vi "myRIO_BRig_RT_v0,60__PortC.vi"() -> ()   [LabVIEW 2014]
uses:
  myRIO_BRig_RT__Case_Exp_stateList.ctl
  myRIO_BRig_RT__Case_NonExp_stateList.ctl
  <vilib>/Platform/TimedLoop/XDataNode/timing_clust.ctl
  <vilib>/Platform/TimedLoop/XDataNode/nitl_modes.ctl
  <vilib>/Platform/TimedLoop/XDataNode/wakeup.ctl
  <vilib>/WebDAVClient/Advanced/SessionHandle.ctl
  <vilib>/myRIO/Common/Instrument Driver Framework/myRIO v1.0/UART/vis/myRIO v1.0 Close UART.vi
  <vilib>/FPGAPlugInAG/myRIO-1900/niLvFpga_Open_myRIO-1900.vi
  <vilib>/rvi/interface/common/dynamic/niFpgaDynamicAddResources.vi
  <vilib>/Utility/error.llb/Error Cluster From Error Code.vi
  <vilib>/rvi/errors/niLvFpgaAdjustHostInterfaceError.vi
  <vilib>/FPGAPlugInAG/Dynamic/niLvFpga_Close_Dynamic.vi
  <vilib>/myRIO/Common/Instrument Driver Framework/Utilities/vis/FPGA Ref Manager.vi
  <vilib>/myRIO/Common/Instrument Driver Framework/myRIO v1.0/myRIO v1.0 Reset FPGA.vi
  <vilib>/myRIO/Common/Instrument Driver Framework/myRIO v1.0/IRQ/vis/myRIO v1.0 IRQ Info FGV.vi
  <vilib>/myRIO/Common/Instrument Driver Framework/myRIO v1.0/IRQ/vis/myRIO v1.0 Timer IRQ Info FGV.vi
  <vilib>/myRIO/Common/Instrument Driver Framework/myRIO v1.0/IRQ/vis/myRIO v1.0 ISR Agent.vi
  <vilib>/rvi/interface/nirviOpenFPGA/nirviOpenFPGA.xnode
  FPGA Bitfiles/myRIOBRig_FPGATarget_myRIOBRigFPGAv3,_GOpVR-pcl6w.lvbitx
  myRIO_BRig_FPGA_v3,51__PortC__testWarmup.vi
  <vilib>/rvi/interface/nirviReadWriteControl/nirviReadWriteControl.xnode
  <vilib>/Platform/TimedLoop/XDataNode/XDataNode.xnode
  <vilib>/rvi/interface/nirviCloseFPGA/nirviCloseFPGA.xnode
  <vilib>/Platform/TimedLoop/XDataNode/XDNodeRunTimeDep.lvlib
  <vilib>/rvi/interface/Simulation/niFpgaSimulationCallBeginRW.vi
  <vilib>/myRIO/Instrument Drivers/Utilities/Utilities.lvlib
  <vilib>/WebDAVClient/NI_WebDAV.lvlib
  NiFpgaLv.dll
panel:
  in  "count_warmup_R_reset":bool
  in  "count_warmup_L_reset":bool
  out "count_warmup_R":u16
  out "count_warmup_L":u16
  out "SolenoidReward":bool
  in  "SolenoidProbability_L":u16=50 caption="Reward Time [ms]" min=1 max=1000 step=1
  in  "SolenoidProbability_R":u16=50 caption="Reward Time [ms]" min=1 max=1000 step=1
  out "output_PortA":dbl
  out "error out 4":errorcluster
  in  "laser_power_step":dbl
  in  "laser_power_max":dbl
  in  "Recording_p2":bool
  in  "Recording":bool
  out "error out 3":errorcluster
  out "error out 2":errorcluster
  in  "laser_power_min":dbl
  in  "f_millisec2count":dbl=159.0
  in  "laser_Tshutter":dbl=2.0
  in  "laser_Freq":dbl=10.0
  in  "laser_Tpeak":dbl=2.0
  in  "laser_duration":u16
  out "error out":errorcluster
  in  "LC_Cue1_All_Count":u16
  in  "LC_Cue1_First_Count":u16
  in  "LC_Cue1_All_delayOpt":bool
  in  "LC_ENL1_All_delayOpt":bool
  in  "LC_ENL1_All_Count":u16
  in  "LC_ENL1_First_Count":u16
  in  "LC_Cue1_First_delayOpt":bool
  in  "LC_ENL1_First_delayOpt":bool
  in  "Tcycle_Cue_max":u16=1000 caption="Max [ms]" min=5 max=5000 step=5
  in  "Tcycle_Cue_min":u16=1000 caption="Min [ms]" min=5 max=5000 step=5
  in  "SendData":bool
  out "cSpout":enum16{"Left", "Right"}(ring) caption="Left or Right Spout"
  out "A4":u32 caption="LickCounter_Right"
  out "A2":u32 caption="LickCounter_Left"
  in  "laserResponse_wrong_LED":bool
  out "error_initTrial":errorcluster
  out "error_Selection_pre":errorcluster
  out "error_Selection":errorcluster
  out "SelectWrong":bool
  out "SelectReward":bool
  in  "Left(F)_or_Right(T)":bool
  in  "ignoreWrong":bool
  in  "SelectionState":bool
  in  "laserResponse_wrong":bool
  in  "laserResponse_reward":bool
  in  "laserResponse_reward_LED":bool
  out "nRewards_Right":u16 caption="# Rewards Total (Right)"
  out "nRewards_Left":u16 caption="# Rewards Total (Left)"
  out "nRewards_cur":u16 caption="# Rewards in Current Block"
  out "TpB_target":u16 caption="Target Trials Per Block"
  out "cState_NonExp":T1 caption="NonExperimental State"
  out "iBlock":u16 caption="Current Block"
  out "cState":T2 caption="Experimental State"
  out "iTrial":u16 caption="Current Trial"
  in  "warmupType":u8(slide) max=2 step=1 scale=0.0..2.0
  in  "TestConnection":bool
  in  "warmup":bool caption="WarmUp"
  in  "Host Filename Prefix":string="Exp1_TM2"
  out "Connected To Host?":bool
  in  "Host Password":string="sabalab"
  in  "Host UserName":string="Test2"
  in  "sp_RightSpout":u16(slide)=2 max=2 step=1 scale=0.0..2.0
  in  "sp_LeftSpout":u16(slide)=2 max=2 step=1 scale=0.0..2.0
  in  "BUR_max":u16 caption="Count Reward Structure  (0 = off)"
  in  "LC_Wrong_Probability":u16
  in  "LC_Wrong_Trial":u16(slide) max=2 step=1 scale=0.0..2.0
  in  "LC_Wrong_Block":u16(slide) max=2 step=1 scale=0.0..2.0
  in  "LC_Wrong_OnOff":bool
  in  "LC_Reward_Probability":u16
  in  "LC_Reward_Trial":u16(slide) max=2 step=1 scale=0.0..2.0
  in  "LC_Reward_Block":u16(slide) max=2 step=1 scale=0.0..2.0
  in  "LC_Reward_OnOff":bool
  in  "LC_Cue1_All_Probability":u16
  in  "LC_Cue1_All_Block":u16(slide) max=2 step=1 scale=0.0..2.0
  in  "LC_Cue1_All_OnOff":bool
  in  "LC_Cue1_First_Probability":u16
  in  "LC_Cue1_First_Block":u16(slide) max=2 step=1 scale=0.0..2.0
  in  "LC_Cue1_First_OnOff":bool
  in  "LC_ENL1_All_Probability":u16 max=100 step=1
  in  "LC_ENL1_All_Block":u16(slide) max=2 step=1 scale=0.0..2.0
  in  "LC_ENL1_All_OnOff":bool
  in  "LC_ENL1_First_Probability":u16 max=100 step=1
  in  "LC_ENL1_First_Block":u16(slide) max=2 step=1 scale=0.0..2.0
  in  "Tcycle_Timeout":u16=1000 caption="Timeout Time [ms]" min=10 max=10000 step=1
  in  "Tcycle_Wrong":u16=1000 caption="Wrong Time [ms]" min=10 max=10000 step=1
  in  "Tcycle_Selection":u16=1000 caption="Answer Time [ms]" min=1 max=10000 step=1
  in  "Tcycle_RewardPost":u16=1000 caption="Consumption Time [ms]" min=250 max=10000 step=250
  in  "Tcycle_Reward_L":u16=500 caption="Reward Time [ms]" min=1 max=1000 step=1
  in  "Tcycle_Reward_R":u16=500 caption="Reward Time [ms]" min=1 max=1000 step=1
  in  "TpB_Max_R":u16=4 caption="Max TrialsPerBlock" min=1 max=12 step=1
  in  "TpB_Min_R":u16=4 caption="Min TrialsPerBlock" min=1 max=12 step=1
  in  "TpB_Max_L":u16=4 caption="Max TrialsPerBlock" min=1 max=12 step=1
  in  "TpB_Min_L":u16=4 caption="Min TrialsPerBlock" min=1 max=12 step=1
  in  "BUR_min":u16 caption="Count Reward Structure  (0 = off)"
  in  "TrialUntilReward":bool caption="Ignore Wrong \nSelection"
  in  "CueCycles":u16=1 caption="Cue Structure" min=1 max=1 step=1
  in  "MTrig_Laser_Tcycle":u16=10 caption="Time [ms]"
  in  "MTrig_Laser_trig":bool
  in  "MTrig_Audio_trig__R":bool caption="Trigger Audio"
  in  "MTrig_Audio_trig__L":bool caption="Trigger Audio"
  in  "RewCalib_Trig_R":bool caption="Calibrate_R"
  in  "RewCalib_Trig_L":bool caption="Calibrate_L"
  in  "MTrig_Solenoid_Tcycle__R":u16=300 caption="Time [ms]"
  in  "MTrig_Solenoid_Tcycle__L":u16=300 caption="Time [ms]"
  in  "MTrig_Solenoid_trig__R":bool caption="Solenoid"
  in  "MTrig_Solenoid_trig__L":bool caption="Solenoid"
  in  "STOP_abort":bool caption="Stop LabView\n(Stops myRio and FPGA)"
  in  "STOP_endBlock":bool caption="Stop Experiment\n@ End of Block"
  in  "STOP_endTrial":bool caption="Stop Experiment\n@ End of Trial"
  in  "START":bool caption="Start Experiment"
  in  "Tcycle_CuePenalty":u16=1000 caption="Penalty [ms]" min=1 max=10000 step=1
  in  "Audio_Amp__R":u16=100 caption="Amp"
  in  "Audio_Freq__R":u8=5 caption="Freq [kHz]" max=14 step=1
  in  "Audio_Amp__L":u16=100 caption="Amp"
  in  "Audio_Freq__L":u8=5 caption="Freq [kHz]" max=14 step=1
  in  "LC_Wrong_Tdelay":u16
  in  "LC_Cue1_All_Tdelay":u16
  in  "LC_ENL1_All_Tdelay":u16
  in  "LC_Reward_Tdelay":u16
  in  "LC_Cue1_First_Tdelay":u16
  in  "LC_ENL1_First_Tdelay":u16
  in  "LC_ENL1_First_OnOff":bool
  in  "Tcycle_ENLPenalty":u16=100 caption="Penalty [ms]" min=10 max=10000 step=10
  in  "Tcycle_ENL_max":u16=1000 caption="Max [ms]" min=250 max=10000 step=250
  in  "Tcycle_ENL_min":u16=1000 caption="Min [ms]" min=250 max=10000 step=250
  # "Manual Control"
  # "Task Structure"
  # "Task Timing"
  # "Laser Control\n\n                                                    On/Off      Block        Probability [%]   Delay [ms]                              Count"
  # "Manual Solenoid Trigger\nLeft              Right"
  # "Master Structure"
  # "Enforced NonLick"
  # "Enforced NonLick 1"
  # "from end"
  # "Time = Cue Min"
  # "Min\n \n  \nMax"
  # "Switch Trial"
  # "from start"
  # "(1) = Switching\n(2) = Two Choice"
  # "from end"
  # "NonSwitch Trials"
  # "Cue"
  # "from start"
  # "Cue 1"
  # "from end"
  # "Switch Trial"
  # "from start"
  # "Min"
  # "Max"
  # "from end"
  # "NonSwitch Trials"
  # "Trial Per Block Structure\n       Left                    Right"
  # "from start"
  # "Spout Selection Control"
  # "Manual Speaker Trigger\nLeft              Right"
  # "Selection Reward"
  # "Answer Time\n         [ms]\n\n  \nWrong Choice Penalty\n         [ms]\n \n \nChoice Timeout Penalty\n         [ms]"
  # "Selection Wrong"
  # "Cue Control"
  # "Left              Right"
  # "State"
  # "Manual Laser Trigger"
  # "Freq [kHz]\n \n \nAmp\n \n\n \n\nSpeaker\nSetting"
  # "Reward Control\n                 Left              Right"
  # "Min = 1\nMax = 32k"
  # "Reward Time\n         [ms]\n\nWater Prob"
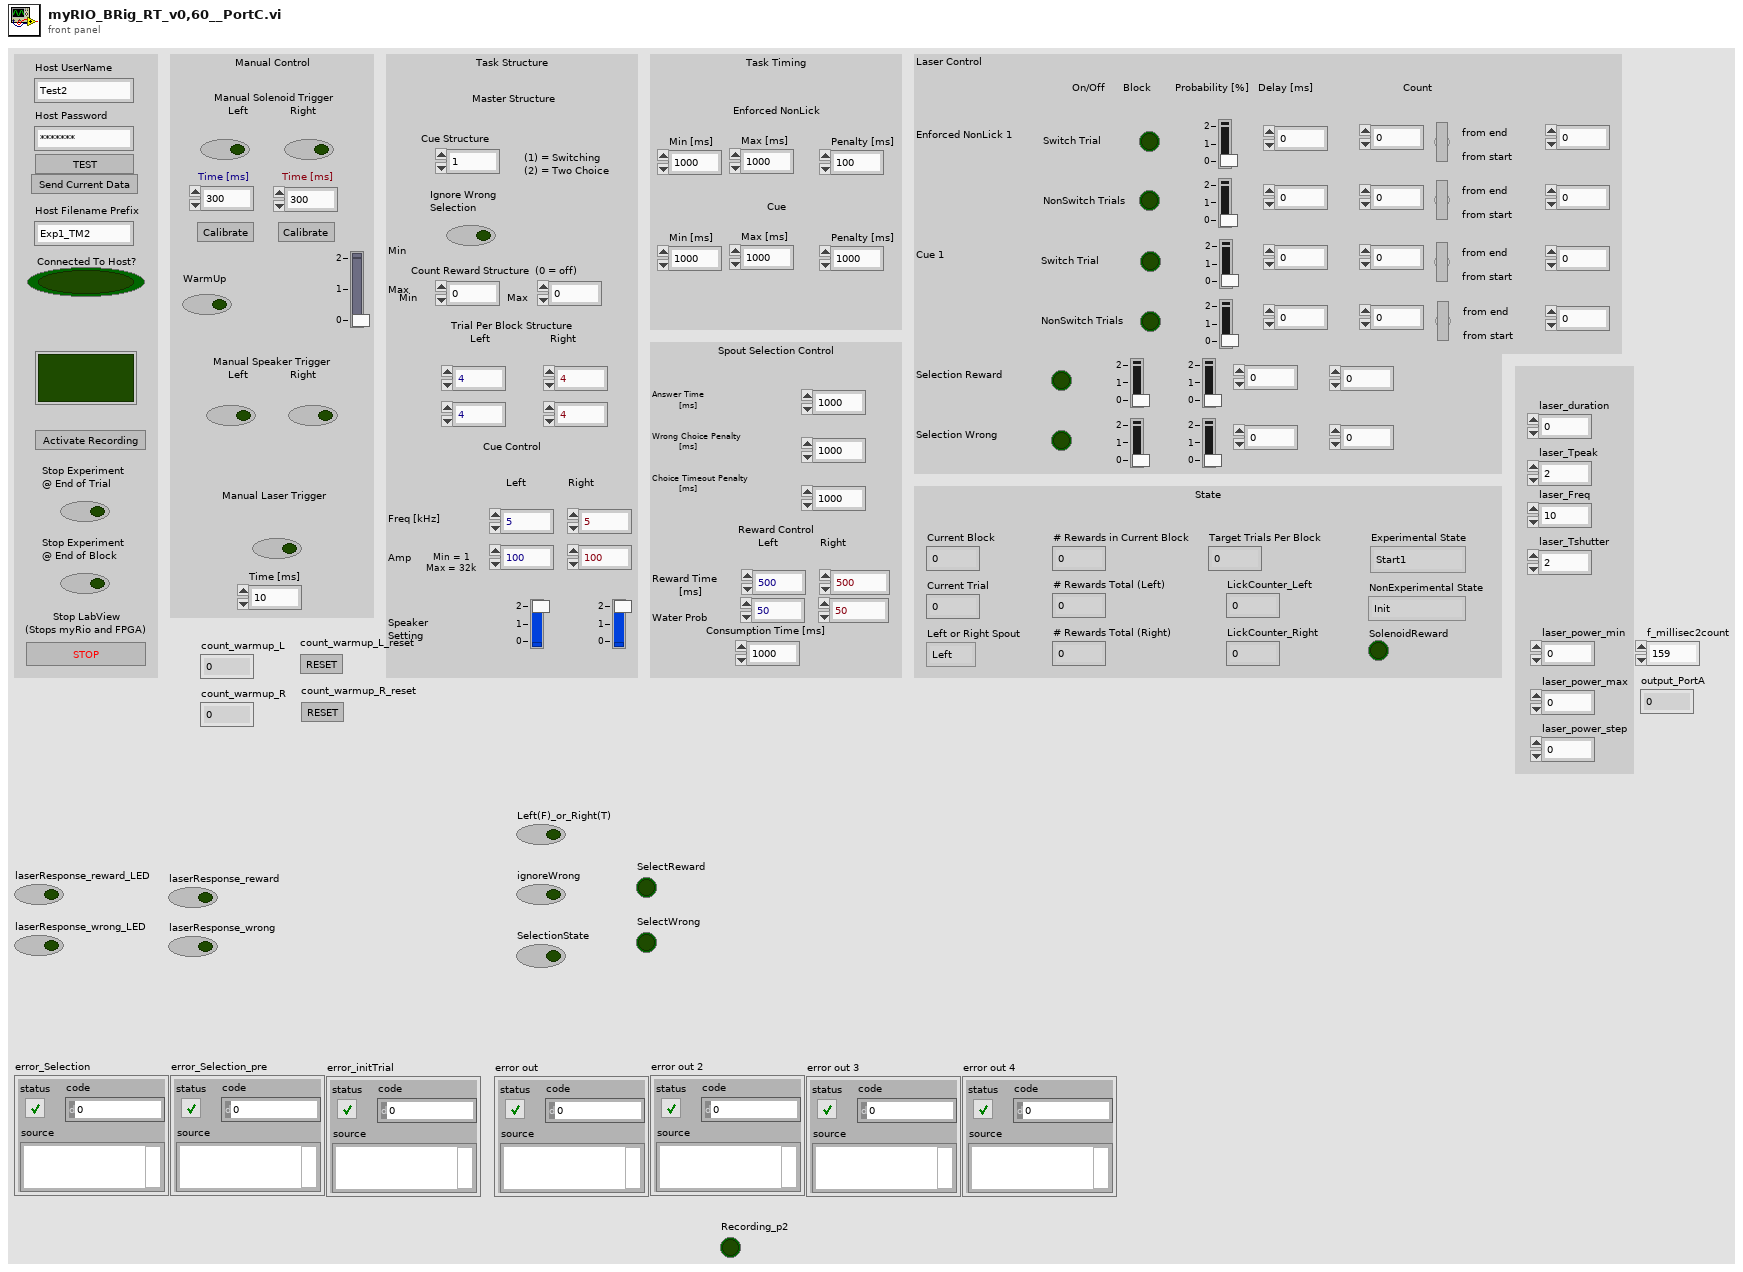
[diagram p1: front panel]
types:
  T1 = typedef "myRIO_BRig_RT__Case_NonExp_stateList.ctl" = enum16{"Init", "UploadSettings_pre", "UploadSettings_Read_dataExp", "UploadSettings_dataExp_1", "UploadSettings_Read_dataLC", "UploadSettings_dataLC_1", "UploadSettings_dataLC_2", "UploadSettings_Read_dataMTrig", "UploadSettings_dataMTrig_1", "UploadSettings_post", "Idle_pre", "IdleEmpty", "IdleEmpty2", "IdleEmpty3", "IdleEmpty4", "Idle", "Idle_2", "Idle_3", "Idle_4", "Idle_post", "Cue_pre__pre", "Cue_pre", "Cue", "Cue_post", "RewardCalibration_pre", "DispenseWater_pre__pre", "DispenseWater_pre", "DispenseWater", "DispenseWater_post", "TestConnection", "SendData", "End"}
  T2 = typedef "myRIO_BRig_RT__Case_Exp_stateList.ctl" = enum16{"Start1", "Start2", "Start3", "saveSettings1", "saveSettings2", "saveSettings3", "saveSettings4_LC_ENL", "saveSettings5_LC_Cue", "saveSettings6_LC_Other", "setSettings_Audio", "setSettings_Laser", "initBlock_pre", "initBlock", "initBlock2", "initBlock_post", "initTrial_pre", "initTrial", "initTrial2", "initTrial3", "initTrial4", "initTrial_LC_ENL1", "initTrial_LC_Cue1", "initTrial_post", "ENL1_pre", "ENL1", "ENL1_post", "ENL1Penalty_pre", "ENL1Penalty", "ENL2_pre", "ENL2", "ENL2Penalty_pre", "ENL2Penalty", "Cue1_pre", "Cue1", "Cue1_post", "Cue1Penalty_pre", "Cue1Penalty", "Cue2_pre", "Cue2", "Cue2Penalty_pre", "Cue2Penalty", "Selection_pre", "Selection", "Select_post", "SelectReward_pre", "SelectReward", "SelectRewardPost_pre", "SelectRewardPost", "SelectWrong_pre", "SelectWrong", "SelectWrong_post", "SelectTimeout_pre", "SelectTimeout", "SelectTimeout_post", "endTrial_pre", "endTrial1", "endTrial2", "endTrial3", "endTrial_post", "endBlock_pre", "endBlock", "endBlock_post", "endExp", "commConnect", "commUpload_pre", "commUpload_dataBlock", "commUpload_dataCurrent", "commUpload_dataExp", "commUpload_dataLC", "commUpload_dataTrial", "commUpload_post", "saveData_pre", "saveData_dataBlock", "saveData_dataCurrent", "saveData_dataExp", "saveData_dataLC", "saveData_dataTrial", "saveData_post", "empty_endBlock1", "empty_endBlock2", "empty_endTrial1", "empty_endTrial2", "empty_endTrial3", "empty_endTrial4", "empty_endTrial5"}
  T3 = typedef "XDNodeRunTimeDep.lvlib/timing_clust.ctl" = cluster{"Expected End [f-1]":u64, "Actual End [f-1]":u64, "Finished Late? [f-1]":bool, "Expected End [i-1]":u64, "Actual End [i-1]":u64, "Finished Late? [i-1]":bool, "Expected Start [i]":u64, "Actual Start [i]":u64, "Expected Start [f]":u64, "Actual Start [f]":u64, "Source Name":string, "Structure Name":string, "Period":i64, "Deadline":i64, "Offset":i64, "Start":i64, "Priority":i32, "Timeout":i32, "Mode":T4, "Wakeup Reason":T5, "Error":errorcluster, "Source Type":string, "Secondary Source Type":string, "Global End Time":u64, "Global Start Time":u64, "Frame Duration":u64, "Iteration Duration":u64, "Assigned CPU":i32, "I/O Scan Engine Mode":u32}
  T4 = typedef "XDNodeRunTimeDep.lvlib/nitl_modes.ctl" = enum32{"No Change", "Process missed periods, maintain original phase", "Discard missed periods, maintain original phase", "Process missed periods, ignore original phase", "Discard missed periods, ignore original phase"}
  T5 = typedef "XDNodeRunTimeDep.lvlib/wakeup.ctl" = enum32{"Normal", "Aborted", "Asynchronous wakeup", "Timing source error", "Timed loop error", "Timeout"}
  T6 = typedef "NI_WebDAV.lvlib/SessionHandle.ctl" = refnum<k1>
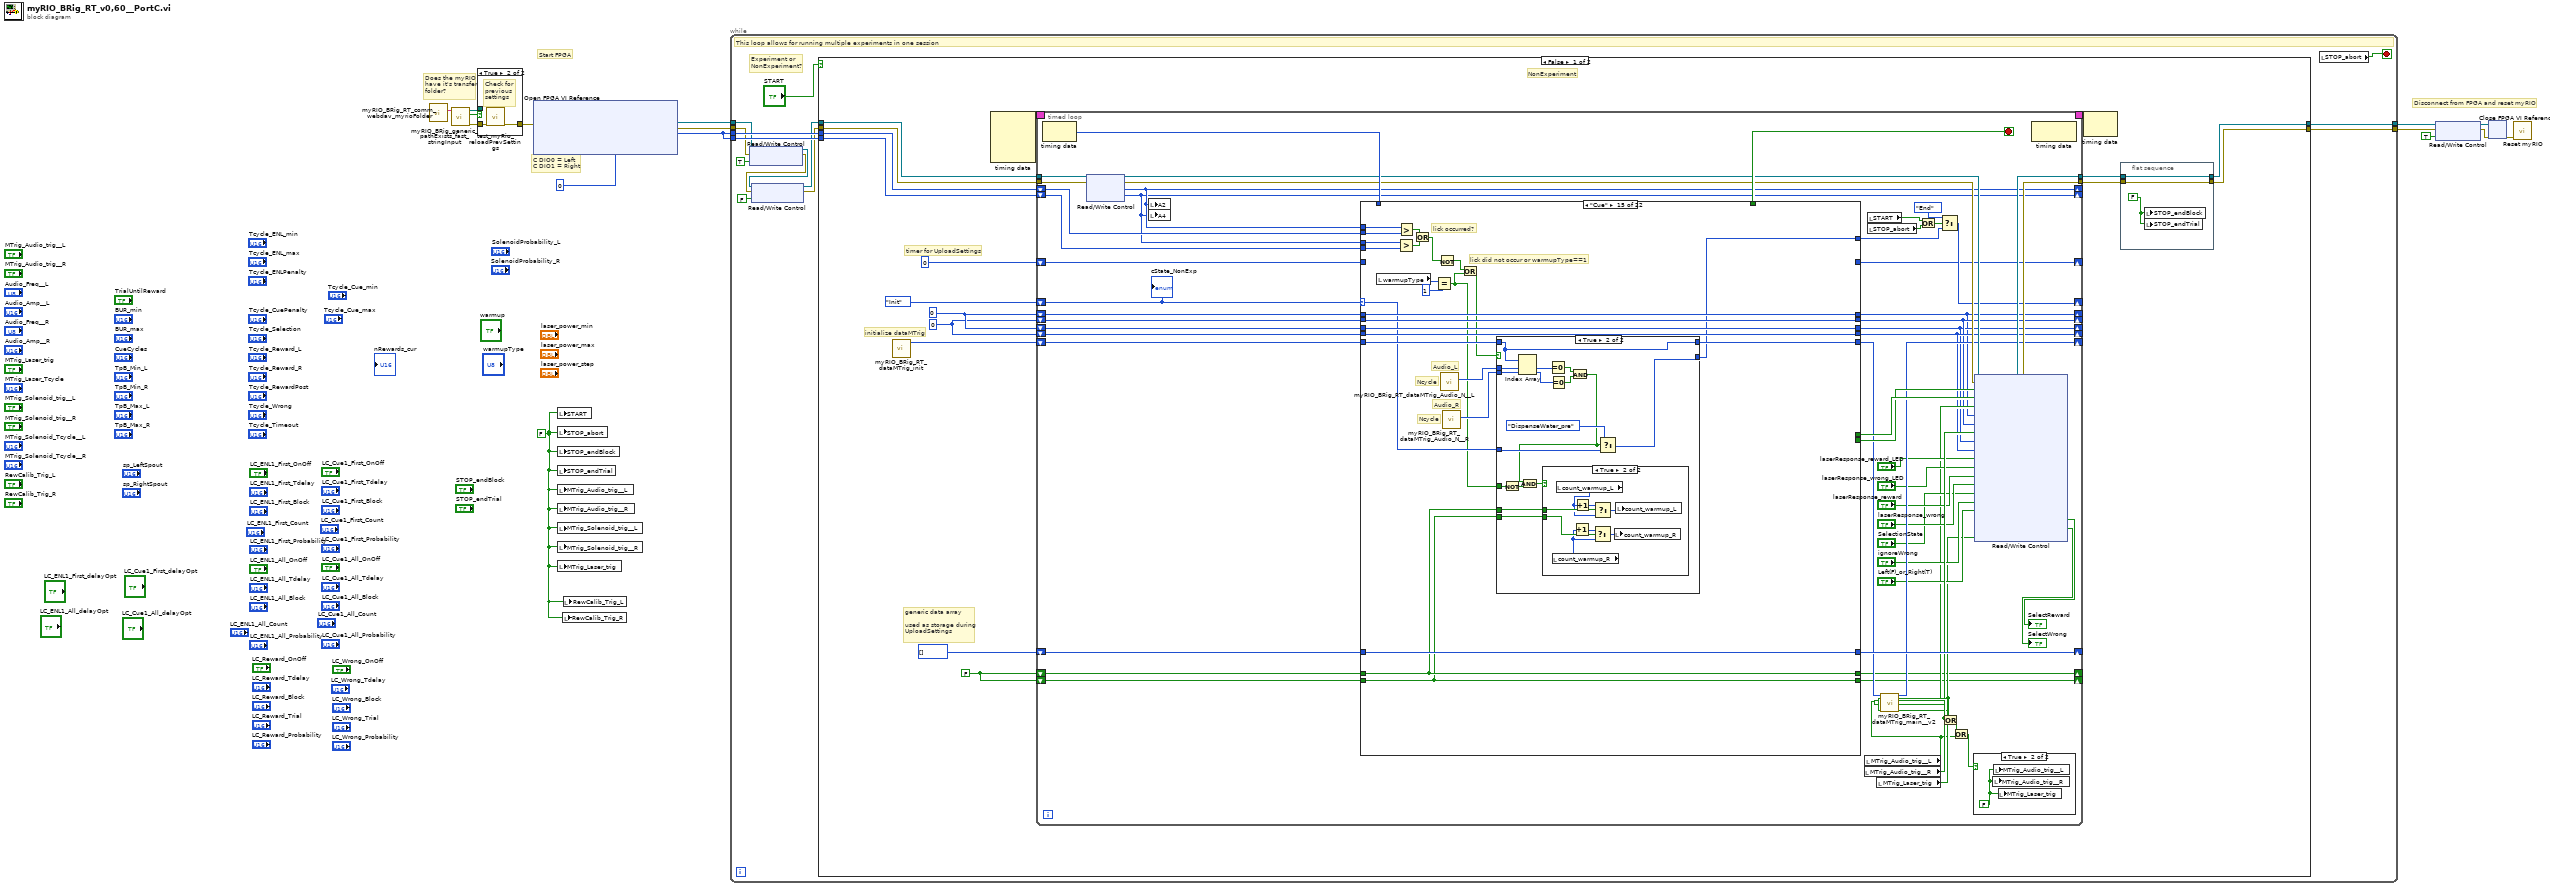
[diagram p0: block diagram]
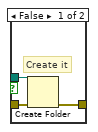
[diagram p2: hidden frame]
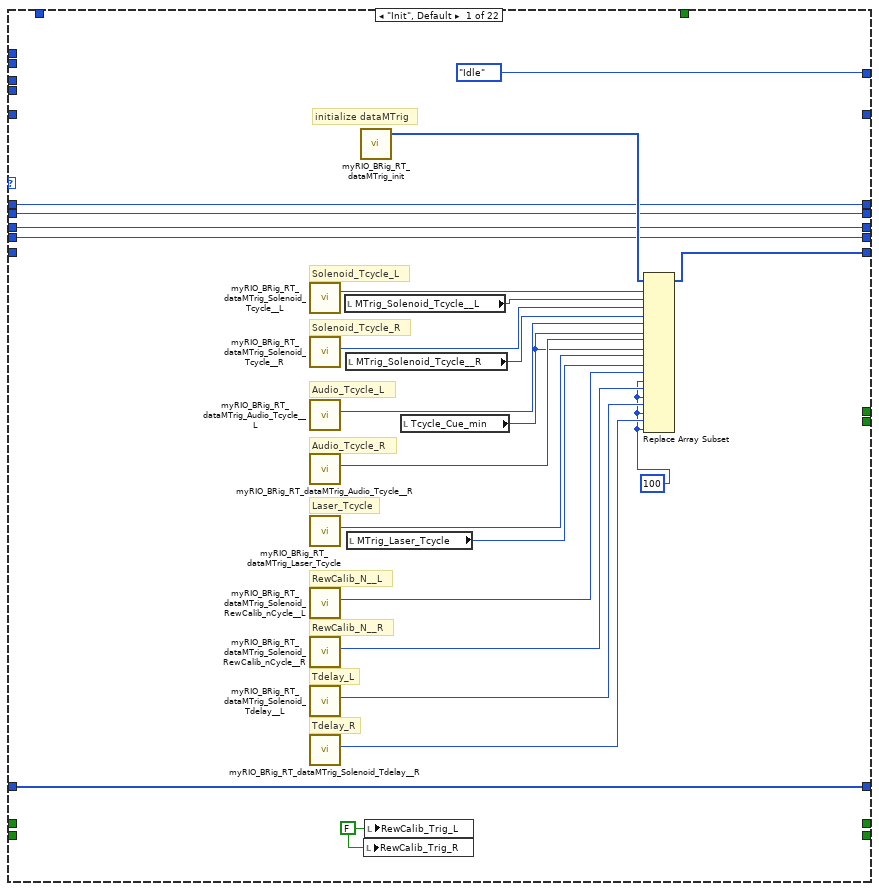
[diagram p4: hidden frame]
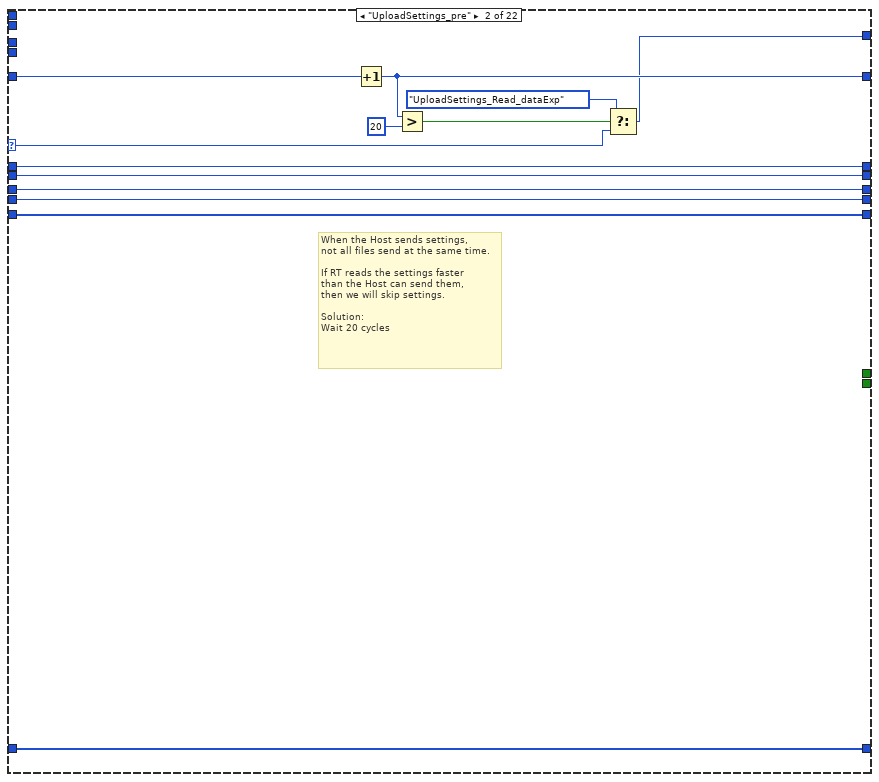
[diagram p5: hidden frame]
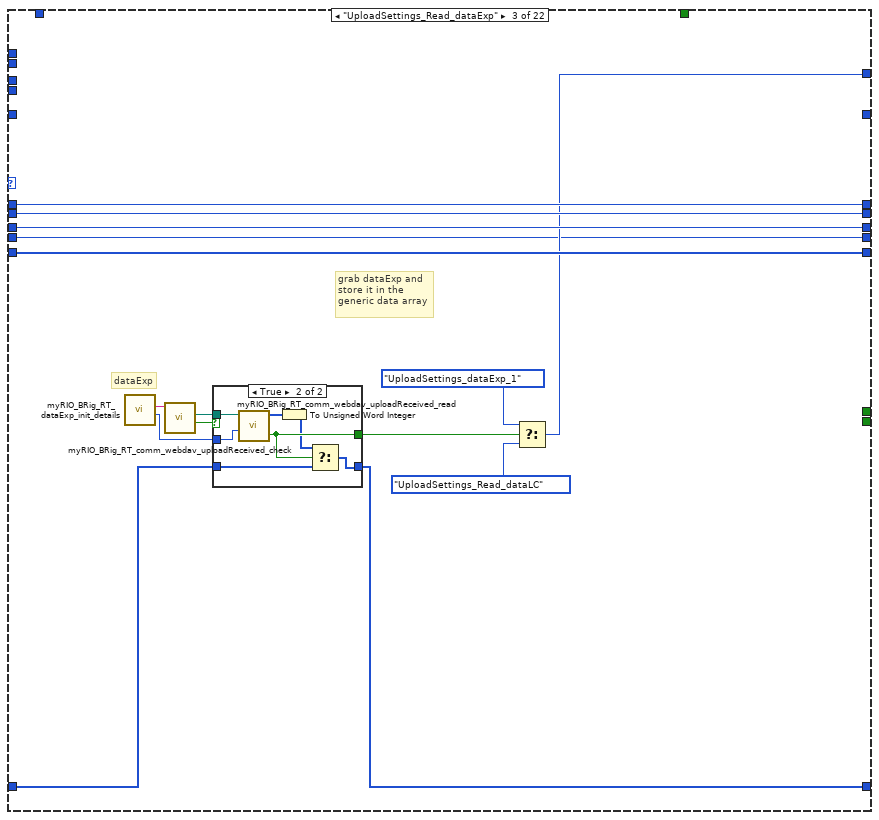
[diagram p6: hidden frame]
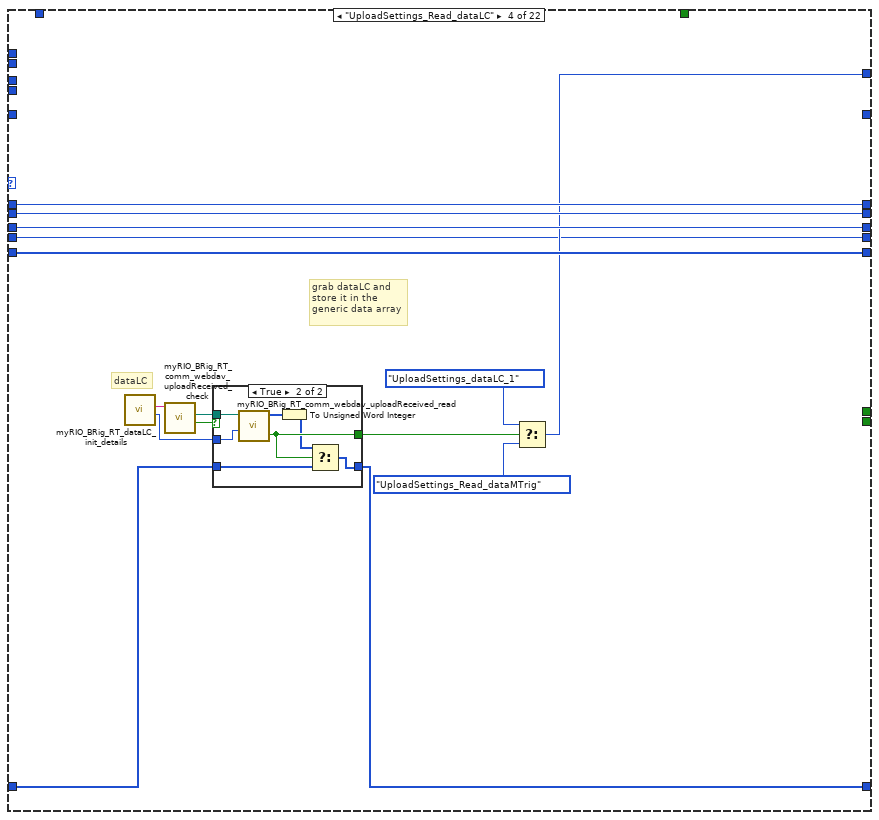
[diagram p8: hidden frame]
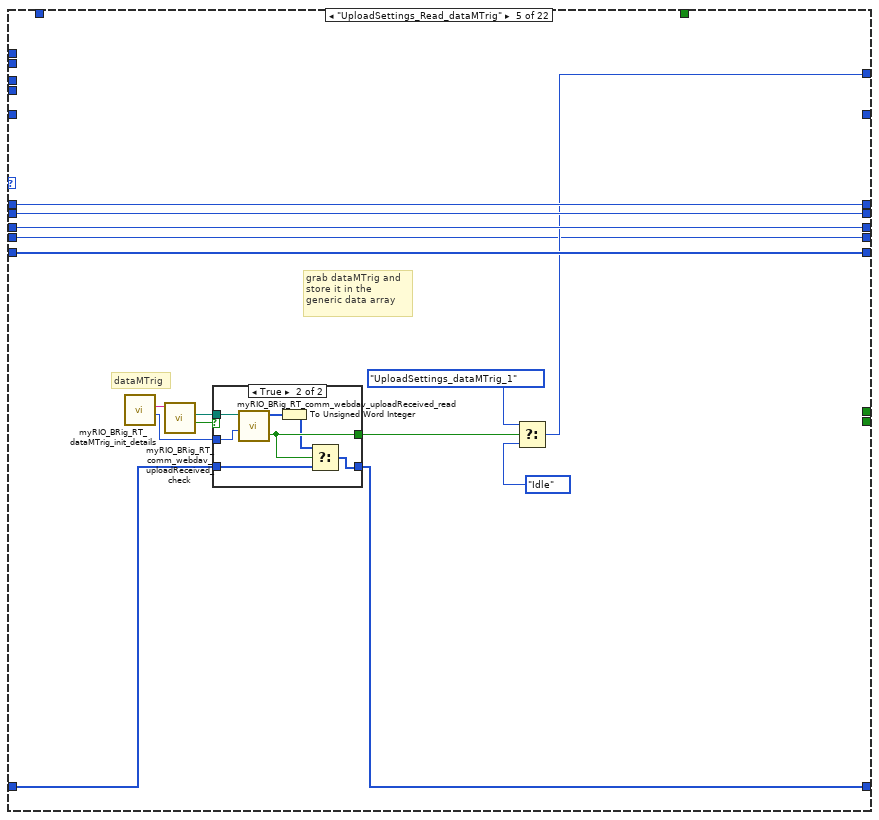
[diagram p10: hidden frame]
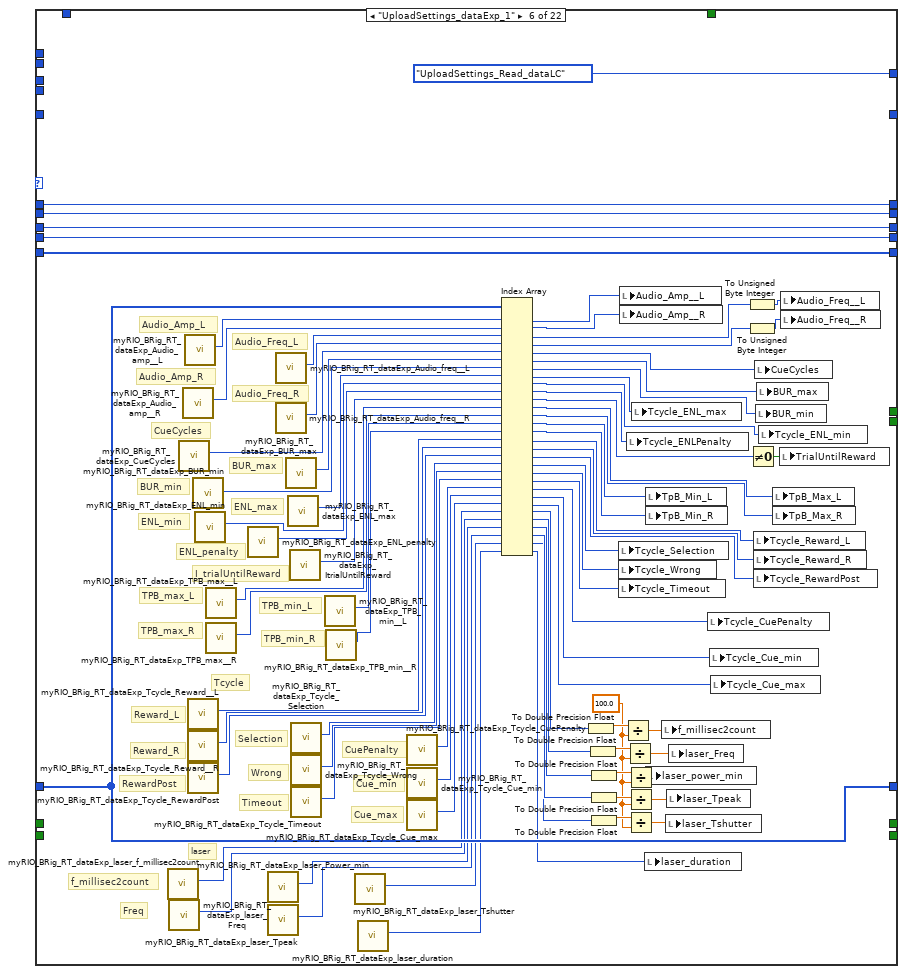
[diagram p12: hidden frame]
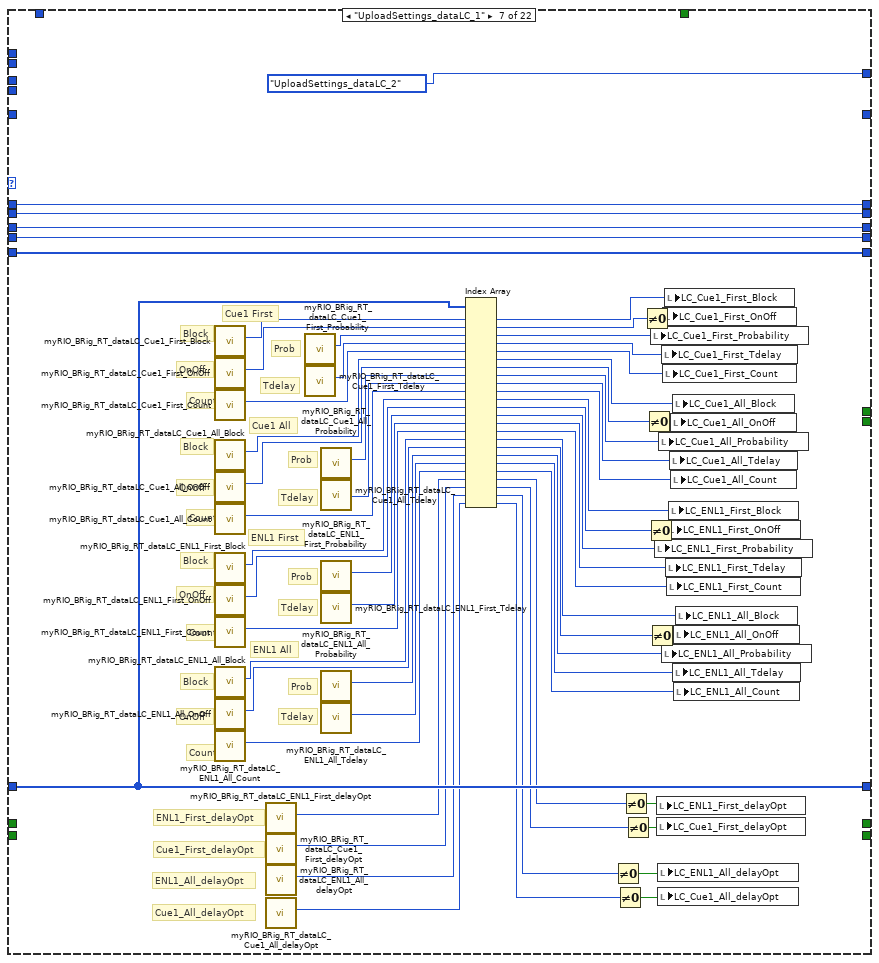
[diagram p13: hidden frame]
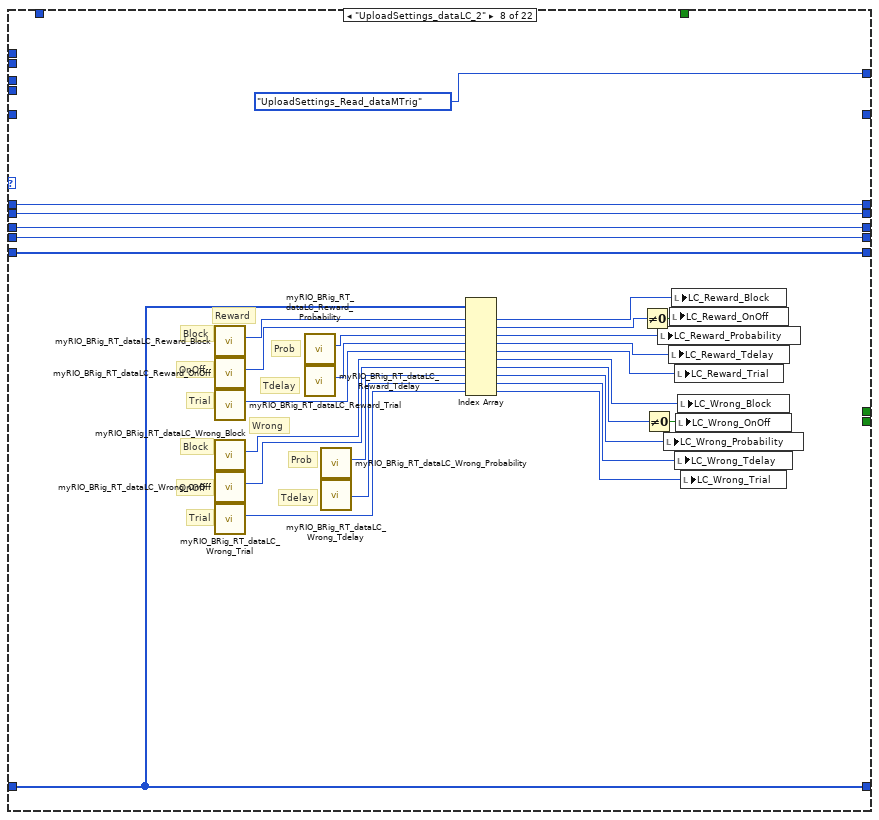
[diagram p14: hidden frame]
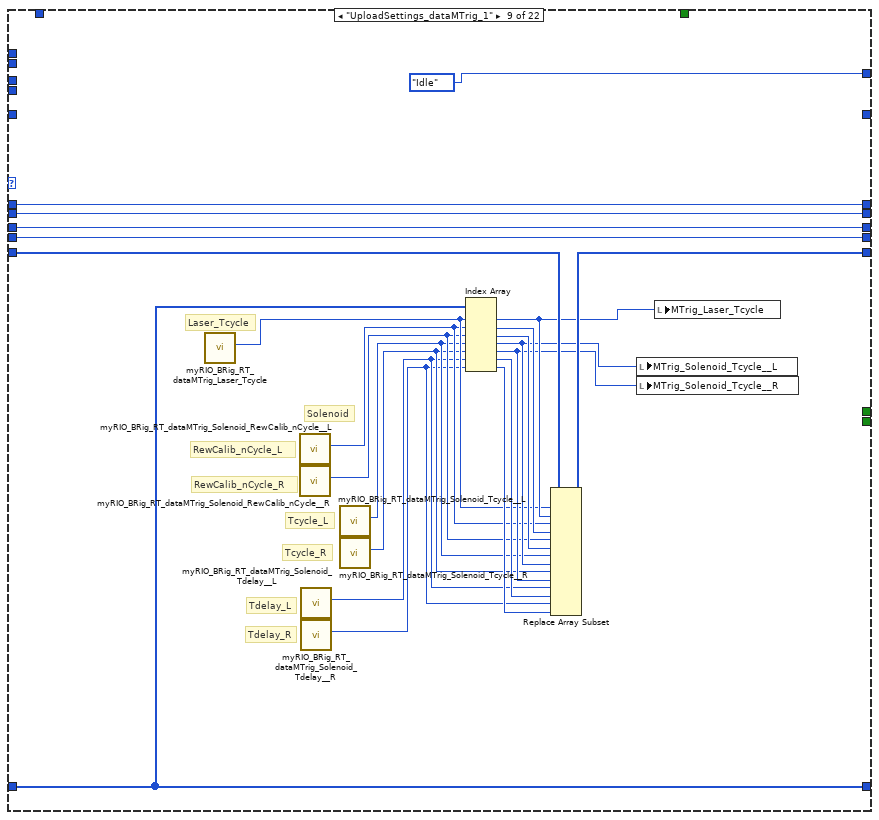
[diagram p15: hidden frame]
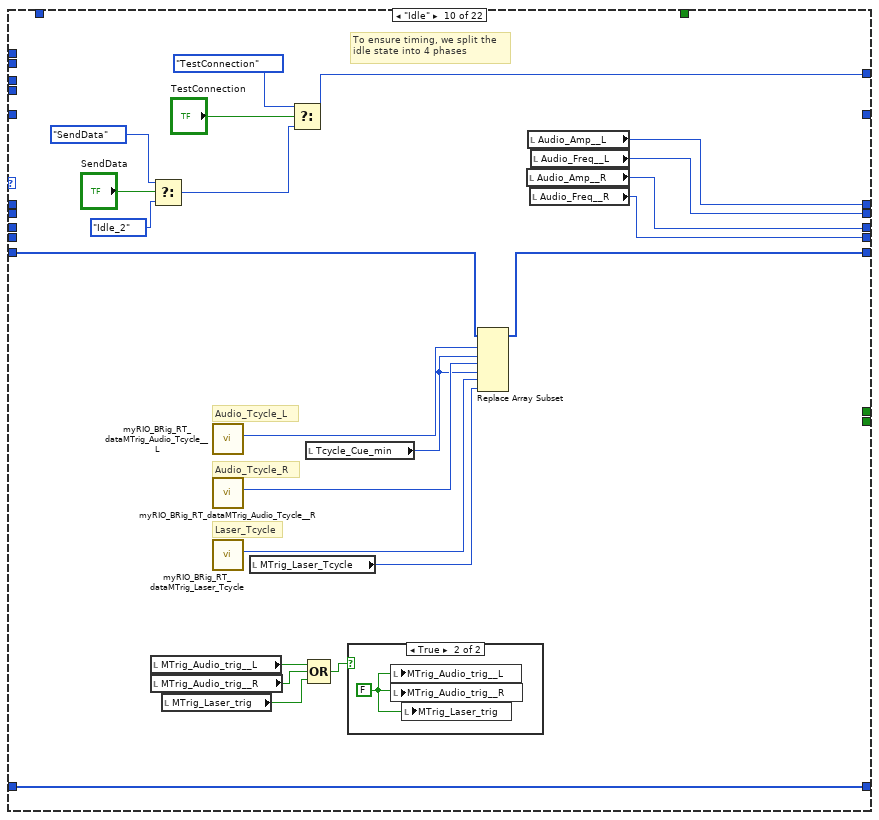
[diagram p16: hidden frame]
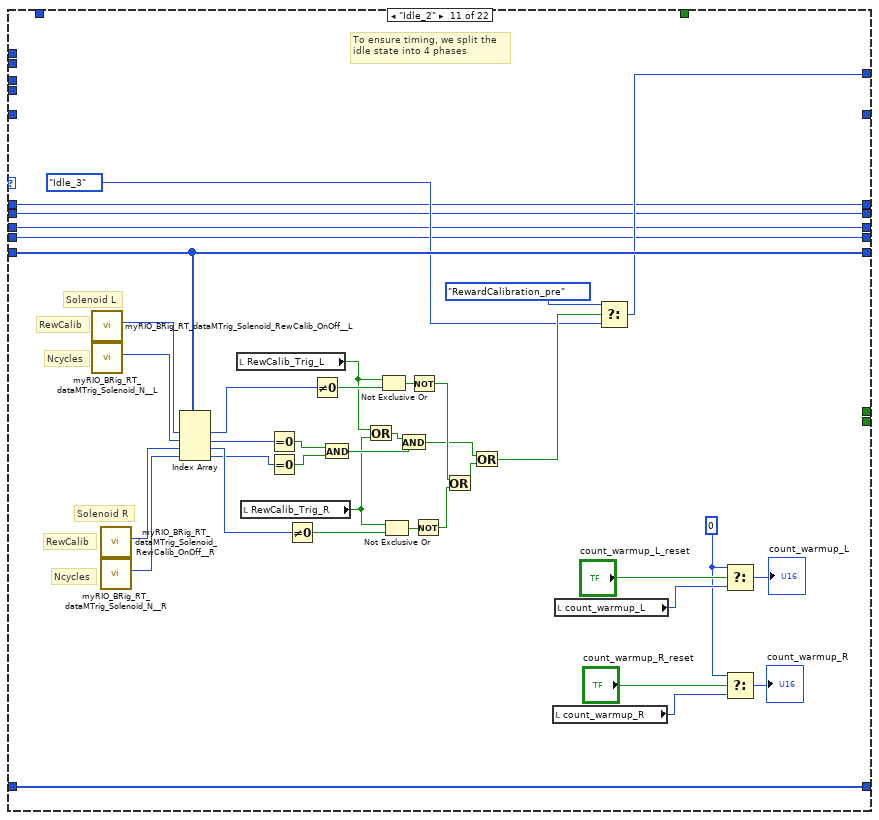
[diagram p18: hidden frame]
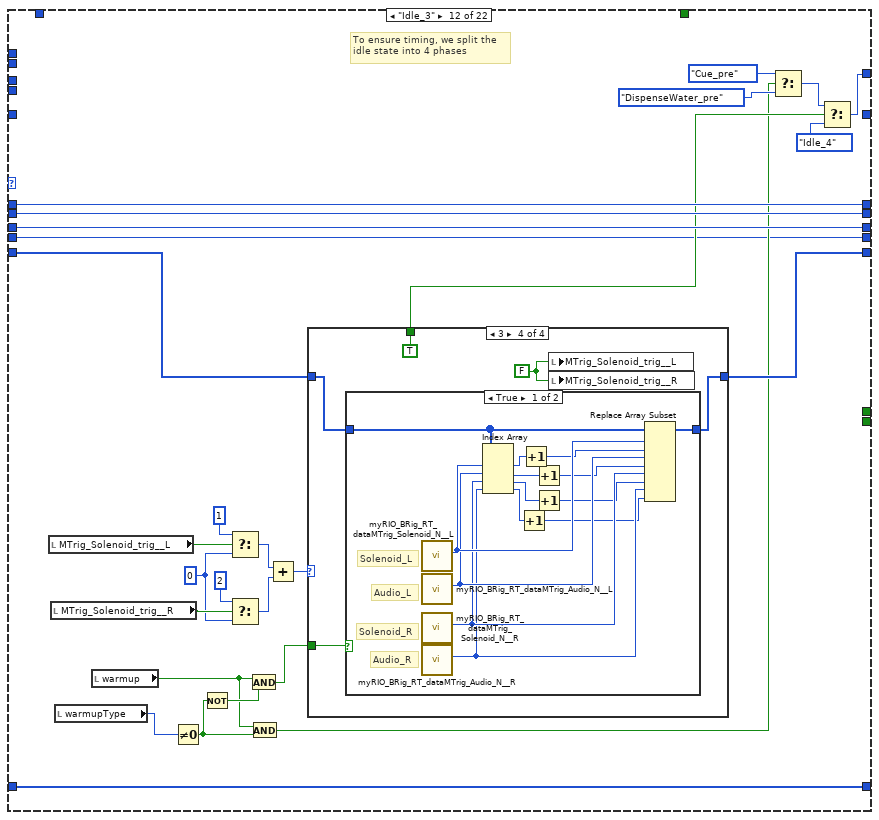
[diagram p19: hidden frame]
diagram:
  w9 = u32 0
  w6 = FALSE
  # "Does the myRIO\nhave it's transfer\nfolder?"
  # "C DIO0 = Left\nC DIO1 = Right"
  # "Start FPGA"
  # "Disconnect from FPGA and reset myRIO"
  n1 = call "myRIO_BRig_RT_comm_webdav_myrioFolder.vi"() -> ("output_myrioFolder"=w4:string)  [unwired: 11 in]
  n2 = call "myRIO_BRig_generic_pathExists_fast_stringInput.vi"("input_filePath"=w4) -> ("output_error"=w3:errorcluster, "output_Iexist"=w2:bool, "output_filePath"=w1:path)  [unwired: 8 in]
  n3 = case shown="True" w2 {
    tunnel: w1 -> [w18 _]
    tunnel: w3 -> [w17 w20]
    tunnel: [w16 w19] -> w5
    frame False {
      # "Create it"
      n4 = Create Folder(path (use dialog)=w18, error in=w17) -> (error out=w16:errorcluster)  [unwired: 1 in, 2 out]
    }
    frame True {
      # "Check for\nprevious\nsettings"
      n5 = call "test_myRio_reloadPrevSettings.vi"("input_error"=w20) -> ("output_error"=w19:errorcluster)  [unwired: 10 in]
    }
  }
  n6 = xnode "Open FPGA VI Reference"("error in"=w5) -> ("FPGA VI Reference Out"=w11:refnum<k20>, "error out"=w10:errorcluster)  [unwired: 1 in]
  n7 = local write "START"(w6) -> ()
  n8 = local write "STOP_abort"(w6) -> ()
  n9 = local write "STOP_endBlock"(w6) -> ()
  n10 = local write "STOP_endTrial"(w6) -> ()
  n11 = local write "MTrig_Audio_trig__L"(w6) -> ()
  n12 = local write "MTrig_Audio_trig__R"(w6) -> ()
  n13 = local write "MTrig_Solenoid_trig__L"(w6) -> ()
  n14 = local write "MTrig_Solenoid_trig__R"(w6) -> ()
  n15 = local write "MTrig_Laser_trig"(w6) -> ()
  n16 = local write "RewCalib_Trig_R"(w6) -> ()
  n17 = local write "RewCalib_Trig_L"(w6) -> ()
  n18 = while {
    tunnel: w11 -> [w24]
    tunnel: w10 -> [w29]
    tunnel: w9 -> [w32]
    tunnel: w9 -> [w31]
    tunnel: [w22] -> w8
    tunnel: [w21] -> w7
    stop <- w30 stop-if-true
    # "Experiment or\nNonExperiment?"
    # "This loop allows for running multiple experiments in one session"
    n19 = xnode "Read/Write Control"("FPGA VI Reference In"=w24, "error in"=w29, "Counts_Reset"=TRUE) -> ("FPGA VI Reference Out"=w26:refnum<k20>, "error out"=w27:errorcluster)
    n20 = xnode "Read/Write Control"("FPGA VI Reference In"=w26, "error in"=w27, "Counts_Reset"=FALSE) -> ("FPGA VI Reference Out"=w23:refnum<k20>, "error out"=w25:errorcluster)
    n21 = case shown="False" "START" {
      tunnel: w32 -> [w47 w987]
      tunnel: w31 -> [w46 w986]
      tunnel: w25 -> [w44 w937]
      tunnel: w23 -> [w45 w936]
      tunnel: [w42 w983] -> w22
      tunnel: [w40 w978] -> w21
      frame False {
        w35 = FALSE
        w36 = u8 0 ("Audio_Amp__L")
        w39 = u16 0 ("Audio_Amp__L")
        # "generic data array\n\nused as storage during\nUploadSettings"
        # "timer for UploadSettings"
        # "initialize dataMTrig"
        # "NonExperiment"
        n22 = call "myRIO_BRig_RT_dataMTrig_init.vi"() -> ("output_dataMTrig"=w48:u16[])  [unwired: 5 in]
        n23 = node-c288() -> (w51:T3)  [unwired: 4 in]
        n24 = timed-loop {
          timing: w51 -> [_]
          timing-out: [_] -> w50
          shift-right: [w93] -> _
          shift-left: w48 -> [w110]
          shift-right: [w82] -> _
          shift-left: myRIO_BRig_RT__Case_NonExp_stateList."Init" ("Enum") -> [w102]
          shift-right: [w61] -> _
          shift-left: w47 -> [w62]
          shift-right: [w59] -> _
          shift-left: w46 -> [w60]
          tunnel: [w105] -> w43
          tunnel: [w103] -> w41
          tunnel: w44 -> [w108]
          tunnel: w45 -> [w107]
          shift-right: [w101] -> _
          shift-left: u16[] [] ("output_data") -> [w100]
          shift-right: [w63] -> _
          shift-left: w39 -> [w99]
          shift-right: [w65] -> _
          shift-left: w36 -> [w98]
          shift-right: [w64] -> _
          shift-left: w39 -> [w97]
          shift-right: [w66] -> _
          shift-left: w36 -> [w67]
          shift-right: [w68] -> _
          shift-left: u16 0 ("Audio_Amp__L") -> [w69]
          shift-right: [w56] -> _
          shift-left: w35 -> [w58]
          shift-right: [w55] -> _
          shift-left: w35 -> [w57]
          stop <- w111 stop-if-true
          n25 = node-c288() -> (w109:i64)  [unwired: 1 in]
          n26 = xnode "Read/Write Control"("FPGA VI Reference In"=w107, "error in"=w108) -> ("FPGA VI Reference Out"=w106:refnum<k20>, "error out"=w104:errorcluster, "A2_LickL"=w61:u32, "A4_LickR"=w59:u32)
          n27 = local write "A2"(w61) -> ()
          n28 = local write "A4"(w59) -> ()
          n29 = case shown="\"Cue\"" w102 {
            selector: w102 -> [_ w144 _ _ _ _ _ _ _ _ _ _ _ _ w610 _ _ w831 _ _ _ w927]
            tunnel: [myRIO_BRig_RT__Case_NonExp_stateList."Idle" ("Enum") w142 w150 w173 w196 myRIO_BRig_RT__Case_NonExp_stateList."UploadSettings_Read_dataLC" ("Enum") myRIO_BRig_RT__Case_NonExp_stateList."UploadSettings_dataLC_2" ("Enum") myRIO_BRig_RT__Case_NonExp_stateList."UploadSettings_Read_dataMTrig" ("f") myRIO_BRig_RT__Case_NonExp_stateList."Idle" ("Enum") w426 w449 w485 w574 myRIO_BRig_RT__Case_NonExp_stateList."Cue" ("t") w605 myRIO_BRig_RT__Case_NonExp_stateList."DispenseWater_pre" ("Enum") w772 w829 w856 myRIO_BRig_RT__Case_NonExp_stateList."Idle" ("Enum") myRIO_BRig_RT__Case_NonExp_stateList."Idle" ("Enum") w927] -> w83
            tunnel: [w127 w138 w160 w183 w206 w298 w361 w390 w410 w432 w464 w494 w572 w591 w611 w681 w809 w836 w867 w909 w919 w925] -> w94
            tunnel: [_ _ _ _ _ _ _ _ _ _ _ _ _ _ _ _ _ _ _ _ _ TRUE] -> w111
            tunnel: w110 -> [_ w138 w160 w183 w206 w298 w361 w390 w411 w431 w464 w495 w572 w592 w612 w667 w805 w837 w868 w909 w919 w925]
            tunnel: w109 -> [_ _ _ _ _ _ _ _ _ _ _ _ _ _ _ _ _ w841 _ _ _ _]
            tunnel: [w117 w137 w151 w174 w197 w244 w314 w363 w392 w421 w445 w479 w568 w581 w620 w659 w757 w814 w849 w898 w914 w921] -> w101
            tunnel: w100 -> [w117 w137 w152 w175 w198 w244 w314 w363 w392 w421 w445 w479 w568 w581 w620 w659 w757 w814 w849 w898 w914 w921]
            tunnel: [w120 w140 w162 w185 w208 w295 w359 w365 w408 w414 w447 w489 w570 w598 w624 w661 w811 w846 w873 w900 w916 w923] -> w65
            tunnel: [w121 w141 w163 w186 w209 w296 w360 w366 w409 w428 w448 w488 w569 w600 w623 w662 w812 w847 w874 w901 w917 w924] -> w63
            tunnel: [w119 w139 w161 w184 w207 w294 w358 w364 w407 w427 w446 w490 w571 w597 w625 w660 w810 w845 w872 w899 w915 w922] -> w64
            tunnel: w99 -> [w121 w141 w163 w186 w209 w296 w360 w366 w409 _ w448 w488 w569 w600 w623 w662 w812 w847 w874 w901 w917 w924]
            tunnel: w98 -> [w120 w140 w162 w185 w208 w295 w359 w365 w408 _ w447 w489 w570 w598 w624 w661 w811 w846 w873 w900 w916 w923]
            tunnel: w97 -> [w119 w139 w161 w184 w207 w294 w358 w364 w407 _ w446 w490 w571 w597 w625 w660 w810 w845 w872 w899 w915 w922]
            tunnel: [_ _ _ _ _ _ _ _ _ _ _ _ _ _ _ _ _ w838 _ _ _ _] -> w96
            tunnel: [_ _ _ _ _ _ _ _ _ _ _ _ _ _ _ _ _ w820 _ _ _ _] -> w95
            tunnel: w69 -> [_ w148 _ _ _ _ _ _ _ _ _ _ _ _ _ _ _ _ _ _ _ _]
            tunnel: [_ w147 _ _ _ _ _ _ _ _ _ _ _ _ _ _ _ _ _ _ _ _] -> w68
            tunnel: w67 -> [w113 w136 w149 w172 w195 w218 w299 w362 w391 _ w444 w478 w567 w580 w619 w658 w756 w813 w848 w897 w910 w920]
            tunnel: [w113 w136 w149 w172 w195 w218 w299 w362 w391 w413 w444 w478 w567 w580 w619 w658 w756 w813 w848 w897 w910 w920] -> w66
            tunnel: w62 -> [_ _ _ _ _ _ _ _ _ _ _ _ _ _ w616 _ _ _ _ _ _ _]
            tunnel: w61 -> [_ _ _ _ _ _ _ _ _ _ _ _ _ _ w617 _ _ _ _ _ _ _]
            tunnel: w60 -> [_ _ _ _ _ _ _ _ _ _ _ _ _ _ w614 _ _ _ _ _ _ _]
            tunnel: w59 -> [_ _ _ _ _ _ _ _ _ _ _ _ _ _ w615 _ _ _ _ _ _ _]
            tunnel: w58 -> [_ _ _ _ _ _ _ _ _ _ _ _ _ _ w602 _ _ _ _ _ _ _]
            tunnel: w57 -> [_ _ _ _ _ _ _ _ _ _ _ _ _ _ w601 _ _ _ _ _ _ _]
            tunnel: [_ _ _ _ _ _ _ _ _ _ _ _ _ w579 w602 _ _ _ _ _ _ _] -> w56
            tunnel: [_ _ _ _ _ _ _ _ _ _ _ _ _ w578 w601 _ _ _ _ _ _ _] -> w55
            frame "Init", Default {
              w118 = FALSE ("RewCalib_Trig_L")
              w114 = u16 100 ("new element/subarray")
              # "Tdelay_R"
              # "Tdelay_L"
              # "RewCalib_N__R"
              # "RewCalib_N__L"
              # "Solenoid_Tcycle_R"
              # "Solenoid_Tcycle_L"
              # "Laser_Tcycle"
              # "Audio_Tcycle_R"
              # "Audio_Tcycle_L"
              # "initialize dataMTrig"
              n30 = call "myRIO_BRig_RT_dataMTrig_Solenoid_Tcycle__L.vi"() -> ("output_Solenoid_Tcycle__L"=w129:i32)  [unwired: 11 in]
              n31 = call "myRIO_BRig_RT_dataMTrig_Solenoid_Tcycle__R.vi"() -> ("output_Solenoid_Tcycle__R"=w130:i32)  [unwired: 11 in]
              n32 = call "myRIO_BRig_RT_dataMTrig_Audio_Tcycle__L.vi"() -> ("output_Audio_Tcycle__L"=w131:i32)  [unwired: 11 in]
              n33 = call "myRIO_BRig_RT_dataMTrig_Audio_Tcycle__R.vi"() -> ("output_Audio_Tcycle__R"=w132:i32)  [unwired: 11 in]
              n34 = call "myRIO_BRig_RT_dataMTrig_Laser_Tcycle.vi"() -> ("output_Laser_Tcycle"=w133:i32)  [unwired: 11 in]
              n35 = call "myRIO_BRig_RT_dataMTrig_Solenoid_RewCalib_nCycle__L.vi"() -> ("output_Solenoid_RewCalib_nCycle__L"=w125:i32)  [unwired: 11 in]
              n36 = call "myRIO_BRig_RT_dataMTrig_Solenoid_RewCalib_nCycle__R.vi"() -> ("output_Solenoid_RewCalib_nCycle__R"=w124:i32)  [unwired: 11 in]
              n37 = call "myRIO_BRig_RT_dataMTrig_Solenoid_Tdelay__L.vi"() -> ("output_Solenoid_Tdelay__L"=w123:i32)  [unwired: 11 in]
              n38 = call "myRIO_BRig_RT_dataMTrig_Solenoid_Tdelay__R.vi"() -> ("output_Solenoid_Tdelay__R"=w122:i32)  [unwired: 11 in]
              n39 = local read "MTrig_Solenoid_Tcycle__L"() -> (w134:u16)
              n40 = local read "MTrig_Solenoid_Tcycle__R"() -> (w135:u16)
              n41 = local read "MTrig_Laser_Tcycle"() -> (w115:u16)
              n42 = call "myRIO_BRig_RT_dataMTrig_init.vi"() -> ("output_dataMTrig"=w128:u16[])  [unwired: 5 in]
              n43 = local write "RewCalib_Trig_R"(w118) -> ()
              n44 = local write "RewCalib_Trig_L"(w118) -> ()
              n45 = local read "Tcycle_Cue_min"() -> (w116:u16)
              n46 = Replace Array Subset(array=w128, new element #1=w134, index #1=w129, new element #2=w135, index #2=w130, new element #3=w116, index #3=w131, new element #4=w116, index #4=w132, new element #5=w115, index #5=w133, new element #6=w114, index #6=w125, new element #7=w114, index #7=w124, new element #8=w114, index #8=w123, new element #9=w114, index #9=w122) -> (w127:u16[])
            }
            frame "UploadSettings_pre" {
              # "When the Host sends settings,\nnot all files send at the same time.\n\nIf RT reads the settings faster\nthan the Host can send them,\nthen we will skip settings.\n\nSolution:\nWait 20 cycles"
              n47 = Increment(x=w148) -> (x+1=w147:u16)
              n48 = Greater?(x=w147, y=u16 20) -> (0:w145:bool)
              n49 = Select(t=myRIO_BRig_RT__Case_NonExp_stateList."UploadSettings_Read_dataExp", s=w145, f=w144) -> (s? t:f=w142:T1)
            }
            frame "UploadSettings_Read_dataExp" {
              # "grab dataExp and\nstore it in the\ngeneric data array"
              # "dataExp"
              n50 = call "myRIO_BRig_RT_dataExp_init_details.vi"() -> ("output_dataSize"=w156:i32, "output_dataName"=w159:string)  [unwired: 10 in]
              n51 = call "myRIO_BRig_RT_comm_webdav_uploadReceived_check.vi"("input_dataName"=w159) -> ("output_Iexist"=w158:bool, "output_dataPath"=w157:path)  [unwired: 9 in]
              n52 = case shown="True" w158 {
                tunnel: w157 -> [_ w171]
                tunnel: w156 -> [_ w170]
                tunnel: [_ w169] -> w155
                tunnel: w152 -> [w164 w168]
                tunnel: [w164 w165] -> w151
                frame False {
                }
                frame True {
                  n53 = call "myRIO_BRig_RT_comm_webdav_uploadReceived_read.vi"("input_dataSize"=w170, "input_filePath"=w171) -> ("output_Ivalid"=w169:bool, "output_data"=w167:i64[])  [unwired: 8 in]
                  n54 = To Unsigned Word Integer(number=w167) -> (unsigned 16bit integer=w166:u16[])
                  n55 = Select(t=w166, s=w169, f=w168) -> (s? t:f=w165:u16[])
                }
              }
              n56 = Select(t=myRIO_BRig_RT__Case_NonExp_stateList."UploadSettings_dataExp_1", s=w155, f=myRIO_BRig_RT__Case_NonExp_stateList."UploadSettings_Read_dataLC" ("t")) -> (s? t:f=w150:T1)
            }
            frame "UploadSettings_Read_dataLC" {
              # "grab dataLC and\nstore it in the\ngeneric data array"
              # "dataLC"
              n57 = call "myRIO_BRig_RT_dataLC_init_details.vi"() -> ("output_dataSize"=w179:i32, "output_dataName"=w182:string)  [unwired: 10 in]
              n58 = call "myRIO_BRig_RT_comm_webdav_uploadReceived_check.vi"("input_dataName"=w182) -> ("output_Iexist"=w181:bool, "output_dataPath"=w180:path)  [unwired: 9 in]
              n59 = case shown="True" w181 {
                tunnel: w180 -> [_ w194]
                tunnel: w179 -> [_ w193]
                tunnel: [_ w192] -> w178
                tunnel: w175 -> [w187 w191]
                tunnel: [w187 w188] -> w174
                frame False {
                }
                frame True {
                  n60 = call "myRIO_BRig_RT_comm_webdav_uploadReceived_read.vi"("input_dataSize"=w193, "input_filePath"=w194) -> ("output_Ivalid"=w192:bool, "output_data"=w190:i64[])  [unwired: 8 in]
                  n61 = To Unsigned Word Integer(number=w190) -> (unsigned 16bit integer=w189:u16[])
                  n62 = Select(t=w189, s=w192, f=w191) -> (s? t:f=w188:u16[])
                }
              }
              n63 = Select(t=myRIO_BRig_RT__Case_NonExp_stateList."UploadSettings_dataLC_1", s=w178, f=myRIO_BRig_RT__Case_NonExp_stateList."UploadSettings_Read_dataMTrig" ("t")) -> (s? t:f=w173:T1)
            }
            frame "UploadSettings_Read_dataMTrig" {
              # "grab dataMTrig and\nstore it in the\ngeneric data array"
              # "dataMTrig"
              n64 = call "myRIO_BRig_RT_dataMTrig_init_details.vi"() -> ("output_dataSize"=w202:i32, "output_dataName"=w205:string)  [unwired: 10 in]
              n65 = call "myRIO_BRig_RT_comm_webdav_uploadReceived_check.vi"("input_dataName"=w205) -> ("output_Iexist"=w204:bool, "output_dataPath"=w203:path)  [unwired: 9 in]
              n66 = case shown="True" w204 {
                tunnel: w203 -> [_ w217]
                tunnel: w202 -> [_ w216]
                tunnel: [_ w215] -> w201
                tunnel: w198 -> [w210 w214]
                tunnel: [w210 w211] -> w197
                frame False {
                }
                frame True {
                  n67 = call "myRIO_BRig_RT_comm_webdav_uploadReceived_read.vi"("input_dataSize"=w216, "input_filePath"=w217) -> ("output_Ivalid"=w215:bool, "output_data"=w213:i64[])  [unwired: 8 in]
                  n68 = To Unsigned Word Integer(number=w213) -> (unsigned 16bit integer=w212:u16[])
                  n69 = Select(t=w212, s=w215, f=w214) -> (s? t:f=w211:u16[])
                }
              }
              n70 = Select(t=myRIO_BRig_RT__Case_NonExp_stateList."UploadSettings_dataMTrig_1", s=w201, f=myRIO_BRig_RT__Case_NonExp_stateList."Idle" ("t")) -> (s? t:f=w196:T1)
            }
            frame "UploadSettings_dataExp_1" {
              w227 = 100.0 ("y")
              # "Freq"
              # "f_millisec2count"
              # "laser"
              # "Cue_max"
              # "Cue_min"
              # "CuePenalty"
              # "Timeout"
              # "Wrong"
              # "Selection"
              # "RewardPost"
              # "Reward_R"
              # "Reward_L"
              # "Tcycle"
              # "TPB_min_R"
              # "TPB_min_L"
              # "TPB_max_R"
              # "TPB_max_L"
              # "I_trialUntilReward"
              # "ENL_penalty"
              # "ENL_min"
              # "ENL_max"
              # "BUR_max"
              # "BUR_min"
              # "CueCycles"
              # "Audio_Freq_R"
              # "Audio_Freq_L"
              # "Audio_Amp_R"
              # "Audio_Amp_L"
              n71 = call "myRIO_BRig_RT_dataExp_laser_f_millisec2count.vi"() -> ("output_laser_f_millisec2count"=w241:i32)  [unwired: 11 in]
              n72 = call "myRIO_BRig_RT_dataExp_laser_Freq.vi"() -> ("output_laser_Freq"=w240:i32)  [unwired: 11 in]
              n73 = call "myRIO_BRig_RT_dataExp_CueCycles.vi"() -> ("output_CueCycles"=w287:i32)  [unwired: 11 in]
              n74 = call "myRIO_BRig_RT_dataExp_Audio_amp__R.vi"() -> ("output_Audio_amp__R"=w291:i32)  [unwired: 11 in]
              n75 = call "myRIO_BRig_RT_dataExp_Audio_amp__L.vi"() -> ("output_Audio_amp__L"=w293:i32)  [unwired: 11 in]
              n76 = call "myRIO_BRig_RT_dataExp_Tcycle_Reward__L.vi"() -> ("output_Tcycle_Reward__L"=w264:i32)  [unwired: 11 in]
              n77 = call "myRIO_BRig_RT_dataExp_Tcycle_Reward__R.vi"() -> ("output_Tcycle_Reward__R"=w263:i32)  [unwired: 11 in]
              n78 = call "myRIO_BRig_RT_dataExp_Tcycle_RewardPost.vi"() -> ("output_Tcycle_RewardPost"=w262:i32)  [unwired: 11 in]
              n79 = call "myRIO_BRig_RT_dataExp_BUR_min.vi"() -> ("output_BUR_min"=w284:i32)  [unwired: 11 in]
              n80 = call "myRIO_BRig_RT_dataExp_ENL_min.vi"() -> ("output_ENL_min"=w280:i32)  [unwired: 11 in]
              n81 = call "myRIO_BRig_RT_dataExp_TPB_max__L.vi"() -> ("output_TPB_max__L"=w272:i32)  [unwired: 11 in]
              n82 = call "myRIO_BRig_RT_dataExp_TPB_max__R.vi"() -> ("output_TPB_max__R"=w271:i32)  [unwired: 11 in]
              n83 = call "myRIO_BRig_RT_dataExp_ENL_penalty.vi"() -> ("output_ENL_penalty"=w279:i32)  [unwired: 11 in]
              n84 = call "myRIO_BRig_RT_dataExp_laser_Power_min.vi"() -> ("output_laser_Power_min"=w239:i32)  [unwired: 11 in]
              n85 = call "myRIO_BRig_RT_dataExp_laser_Tpeak.vi"() -> ("output_laser_Tpeak"=w238:i32)  [unwired: 11 in]
              n86 = call "myRIO_BRig_RT_dataExp_Audio_freq__L.vi"() -> ("output_Audio_freq__L"=w289:i32)  [unwired: 11 in]
              n87 = call "myRIO_BRig_RT_dataExp_Audio_freq__R.vi"() -> ("output_Audio_freq__R"=w288:i32)  [unwired: 11 in]
              n88 = call "myRIO_BRig_RT_dataExp_BUR_max.vi"() -> ("output_BUR_max"=w285:i32)  [unwired: 11 in]
              n89 = call "myRIO_BRig_RT_dataExp_ENL_max.vi"() -> ("output_ENL_max"=w281:i32)  [unwired: 11 in]
              n90 = call "myRIO_BRig_RT_dataExp_ItrialUntilReward.vi"() -> ("output_I_trialUntilReward"=w275:i32)  [unwired: 11 in]
              n91 = call "myRIO_BRig_RT_dataExp_Tcycle_Selection.vi"() -> ("output_Tcycle_Selection"=w261:i32)  [unwired: 11 in]
              n92 = call "myRIO_BRig_RT_dataExp_Tcycle_Wrong.vi"() -> ("output_Tcycle_Wrong"=w260:i32)  [unwired: 11 in]
              n93 = call "myRIO_BRig_RT_dataExp_Tcycle_Timeout.vi"() -> ("output_Tcycle_Timeout"=w259:i32)  [unwired: 11 in]
              n94 = call "myRIO_BRig_RT_dataExp_TPB_min__L.vi"() -> ("output_TPB_min__L"=w270:i32)  [unwired: 11 in]
              n95 = call "myRIO_BRig_RT_dataExp_TPB_min__R.vi"() -> ("output_TPB_min__R"=w269:i32)  [unwired: 11 in]
              n96 = call "myRIO_BRig_RT_dataExp_laser_Tshutter.vi"() -> ("output_laser_Tshutter"=w237:i32)  [unwired: 11 in]
              n97 = call "myRIO_BRig_RT_dataExp_laser_duration.vi"() -> ("output_laser_duration"=w236:i32)  [unwired: 11 in]
              n98 = call "myRIO_BRig_RT_dataExp_Tcycle_CuePenalty.vi"() -> ("output_Tcycle_CuePenalty"=w252:i32)  [unwired: 11 in]
              n99 = call "myRIO_BRig_RT_dataExp_Tcycle_Cue_min.vi"() -> ("output_Tcycle_Cue_min"=w251:i32)  [unwired: 11 in]
              n100 = call "myRIO_BRig_RT_dataExp_Tcycle_Cue_max.vi"() -> ("output_Tcycle_Cue_max"=w250:i32)  [unwired: 11 in]
              n101 = Index Array(array=w244, index #1=w293, index #2=w291, index #3=w289, index #4=w288, index #5=w287, index #6=w285, index #7=w284, index #8=w281, index #9=w280, index #10=w279, index #11=w275, index #12=w272, index #13=w271, index #14=w270, index #15=w269, index #16=w264, index #17=w263, index #18=w262, index #19=w261, index #20=w260, index #21=w259, index #22=w252, index #23=w251, index #24=w250, index #25=w241, index #26=w240, index #27=w239, index #28=w238, index #29=w237, index #30=w236) -> (element #1=w292:u16, element #2=w290:u16, element #3=w247:u16, element #4=w246:u16, element #5=w286:u16, element #6=w283:u16, element #7=w282:u16, element #8=w278:u16, element #9=w277:u16, element #10=w276:u16, element #11=w273:u16, element #12=w268:u16, element #13=w267:u16, element #14=w266:u16, element #15=w265:u16, element #16=w258:u16, element #17=w257:u16, element #18=w256:u16, element #19=w255:u16, element #20=w254:u16, element #21=w253:u16, element #22=w249:u16, element #23=w243:u16, element #24=w242:u16, element #25=w235:u16, element #26=w226:u16, element #27=w225:u16, element #28=w224:u16, element #29=w223:u16, element #30=w219:u16)
              n102 = To Double Precision Float(number=w235) -> (double precision float=w234:dbl)
              n103 = To Double Precision Float(number=w226) -> (double precision float=w232:dbl)
              n104 = To Double Precision Float(number=w225) -> (double precision float=w230:dbl)
              n105 = To Double Precision Float(number=w224) -> (double precision float=w229:dbl)
              n106 = To Double Precision Float(number=w223) -> (double precision float=w228:dbl)
              n107 = local write "Tcycle_Selection"(w255) -> ()
              n108 = local write "Tcycle_Wrong"(w254) -> ()
              n109 = local write "Tcycle_Timeout"(w253) -> ()
              n110 = local write "Audio_Amp__L"(w292) -> ()
              n111 = local write "Audio_Amp__R"(w290) -> ()
              n112 = Divide(x=w234, y=w227) -> (x/y=w233:dbl)
              n113 = Divide(x=w232, y=w227) -> (x/y=w231:dbl)
              n114 = Divide(x=w230, y=w227) -> (x/y=w222:dbl)
              n115 = Divide(x=w229, y=w227) -> (x/y=w221:dbl)
              n116 = Divide(x=w228, y=w227) -> (x/y=w220:dbl)
              n117 = local write "Tcycle_ENLPenalty"(w276) -> ()
              n118 = local write "Tcycle_ENL_max"(w278) -> ()
              n119 = local write "laser_duration"(w219) -> ()
              n120 = local write "TpB_Min_L"(w266) -> ()
              n121 = local write "TpB_Min_R"(w265) -> ()
              n122 = local write "laser_power_min"(w222) -> ()
              n123 = local write "f_millisec2count"(w233) -> ()
              n124 = local write "laser_Tshutter"(w220) -> ()
              n125 = local write "laser_Tpeak"(w221) -> ()
              n126 = local write "laser_Freq"(w231) -> ()
              n127 = local write "Tcycle_CuePenalty"(w249) -> ()
              n128 = local write "Tcycle_Cue_min"(w243) -> ()
              n129 = local write "Tcycle_Cue_max"(w242) -> ()
              n130 = To Unsigned Byte Integer(number=w247) -> (unsigned 8bit integer=w248:u8)
              n131 = To Unsigned Byte Integer(number=w246) -> (unsigned 8bit integer=w245:u8)
              n132 = Not Equal To 0?(x=w273) -> (x != 0?=w274:bool)
              n133 = local write "Tcycle_Reward_L"(w258) -> ()
              n134 = local write "Tcycle_Reward_R"(w257) -> ()
              n135 = local write "Tcycle_RewardPost"(w256) -> ()
              n136 = local write "CueCycles"(w286) -> ()
              n137 = local write "BUR_min"(w282) -> ()
              n138 = local write "BUR_max"(w283) -> ()
              n139 = local write "Tcycle_ENL_min"(w277) -> ()
              n140 = local write "TpB_Max_L"(w268) -> ()
              n141 = local write "TpB_Max_R"(w267) -> ()
              n142 = local write "TrialUntilReward"(w274) -> ()
              n143 = local write "Audio_Freq__L"(w248) -> ()
              n144 = local write "Audio_Freq__R"(w245) -> ()
            }
            frame "UploadSettings_dataLC_1" {
              # "Cue1_All_delayOpt"
              # "ENL1_All_delayOpt"
              # "Cue1_First_delayOpt"
              # "ENL1_First_delayOpt"
              # "ENL1 First"
              # "Cue1 All"
              # "Cue1 First"
              # "Count"
              # "Tdelay"
              # "Prob"
              # "OnOff"
              # "Block"
              # "ENL1 All"
              # "Count"
              # "Tdelay"
              # "Prob"
              # "OnOff"
              # "Block"
              # "Count"
              # "Tdelay"
              # "Prob"
              # "Block"
              # "OnOff"
              # "Count"
              # "Tdelay"
              # "Prob"
              # "OnOff"
              # "Block"
              n145 = call "myRIO_BRig_RT_dataLC_Cue1_First_Block.vi"() -> ("output_Cue1_First_Block"=w356:i32)  [unwired: 11 in]
              n146 = call "myRIO_BRig_RT_dataLC_Cue1_First_OnOff.vi"() -> ("output_Cue1_First_OnOff"=w354:i32)  [unwired: 11 in]
              n147 = call "myRIO_BRig_RT_dataLC_Cue1_First_Count.vi"() -> ("output_Cue1_First_Count"=w351:i32)  [unwired: 11 in]
              n148 = call "myRIO_BRig_RT_dataLC_Cue1_All_Block.vi"() -> ("output_Cue1_All_Block"=w338:i32)  [unwired: 11 in]
              n149 = call "myRIO_BRig_RT_dataLC_Cue1_All_OnOff.vi"() -> ("output_Cue1_All_OnOff"=w337:i32)  [unwired: 11 in]
              n150 = call "myRIO_BRig_RT_dataLC_Cue1_All_Count.vi"() -> ("output_Cue1_All_Count"=w348:i32)  [unwired: 11 in]
              n151 = call "myRIO_BRig_RT_dataLC_ENL1_First_Block.vi"() -> ("output_ENL1_First_Block"=w336:i32)  [unwired: 11 in]
              n152 = call "myRIO_BRig_RT_dataLC_ENL1_First_OnOff.vi"() -> ("output_ENL1_First_OnOff"=w347:i32)  [unwired: 11 in]
              n153 = call "myRIO_BRig_RT_dataLC_ENL1_First_Count.vi"() -> ("output_ENL1_First_Count"=w344:i32)  [unwired: 11 in]
              n154 = call "myRIO_BRig_RT_dataLC_ENL1_All_Block.vi"() -> ("output_ENL1_All_Block"=w343:i32)  [unwired: 11 in]
              n155 = call "myRIO_BRig_RT_dataLC_ENL1_All_OnOff.vi"() -> ("output_ENL1_All_OnOff"=w342:i32)  [unwired: 11 in]
              n156 = call "myRIO_BRig_RT_dataLC_ENL1_All_Count.vi"() -> ("output_ENL1_All_Count"=w339:i32)  [unwired: 11 in]
              n157 = call "myRIO_BRig_RT_dataLC_ENL1_First_delayOpt.vi"() -> ("output_ENL1_First_delayOpt"=w313:i32)  [unwired: 11 in]
              n158 = call "myRIO_BRig_RT_dataLC_Cue1_First_delayOpt.vi"() -> ("output_Cue1_First_delayOpt"=w312:i32)  [unwired: 11 in]
              n159 = call "myRIO_BRig_RT_dataLC_ENL1_All_delayOpt.vi"() -> ("output_ENL1_All_delayOpt"=w305:i32)  [unwired: 11 in]
              n160 = call "myRIO_BRig_RT_dataLC_Cue1_All_delayOpt.vi"() -> ("output_Cue1_All_delayOpt"=w304:i32)  [unwired: 11 in]
              n161 = call "myRIO_BRig_RT_dataLC_Cue1_First_Probability.vi"() -> ("output_Cue1_First_Probability"=w353:i32)  [unwired: 11 in]
              n162 = call "myRIO_BRig_RT_dataLC_Cue1_First_Tdelay.vi"() -> ("output_Cue1_First_Tdelay"=w352:i32)  [unwired: 11 in]
              n163 = call "myRIO_BRig_RT_dataLC_Cue1_All_Probability.vi"() -> ("output_Cue1_All_Probability"=w350:i32)  [unwired: 11 in]
              n164 = call "myRIO_BRig_RT_dataLC_Cue1_All_Tdelay.vi"() -> ("output_Cue1_All_Tdelay"=w349:i32)  [unwired: 11 in]
              n165 = call "myRIO_BRig_RT_dataLC_ENL1_First_Probability.vi"() -> ("output_ENL1_First_Probability"=w346:i32)  [unwired: 11 in]
              n166 = call "myRIO_BRig_RT_dataLC_ENL1_First_Tdelay.vi"() -> ("output_ENL1_First_Tdelay"=w345:i32)  [unwired: 11 in]
              n167 = call "myRIO_BRig_RT_dataLC_ENL1_All_Probability.vi"() -> ("output_ENL1_All_Probability"=w341:i32)  [unwired: 11 in]
              n168 = call "myRIO_BRig_RT_dataLC_ENL1_All_Tdelay.vi"() -> ("output_ENL1_All_Tdelay"=w340:i32)  [unwired: 11 in]
              n169 = Index Array(array=w314, index #1=w356, index #2=w354, index #3=w353, index #4=w352, index #5=w351, index #6=w338, index #7=w337, index #8=w350, index #9=w349, index #10=w348, index #11=w336, index #12=w347, index #13=w346, index #14=w345, index #15=w344, index #16=w343, index #17=w342, index #18=w341, index #19=w340, index #20=w339, index #21=w313, index #22=w312, index #23=w305, index #24=w304) -> (element #1=w355:u16, element #2=w334:u16, element #3=w333:u16, element #4=w332:u16, element #5=w331:u16, element #6=w327:u16, element #7=w326:u16, element #8=w325:u16, element #9=w324:u16, element #10=w323:u16, element #11=w322:u16, element #12=w321:u16, element #13=w320:u16, element #14=w319:u16, element #15=w306:u16, element #16=w318:u16, element #17=w317:u16, element #18=w316:u16, element #19=w315:u16, element #20=w307:u16, element #21=w310:u16, element #22=w308:u16, element #23=w301:u16, element #24=w300:u16)
              n170 = Not Equal To 0?(x=w301) -> (x != 0?=w303:bool)
              n171 = Not Equal To 0?(x=w300) -> (x != 0?=w302:bool)
              n172 = Not Equal To 0?(x=w310) -> (x != 0?=w311:bool)
              n173 = Not Equal To 0?(x=w308) -> (x != 0?=w309:bool)
              n174 = Not Equal To 0?(x=w334) -> (x != 0?=w335:bool)
              n175 = Not Equal To 0?(x=w326) -> (x != 0?=w330:bool)
              n176 = Not Equal To 0?(x=w321) -> (x != 0?=w329:bool)
              n177 = Not Equal To 0?(x=w317) -> (x != 0?=w328:bool)
              n178 = local write "LC_Cue1_First_Probability"(w333) -> ()
              n179 = local write "LC_ENL1_First_Probability"(w320) -> ()
              n180 = local write "LC_ENL1_First_delayOpt"(w311) -> ()
              n181 = local write "LC_Cue1_First_delayOpt"(w309) -> ()
              n182 = local write "LC_ENL1_All_delayOpt"(w303) -> ()
              n183 = local write "LC_Cue1_All_delayOpt"(w302) -> ()
              n184 = local write "LC_Cue1_All_Probability"(w325) -> ()
              n185 = local write "LC_Cue1_First_Tdelay"(w332) -> ()
              n186 = local write "LC_ENL1_All_Probability"(w316) -> ()
              n187 = local write "LC_Cue1_First_OnOff"(w335) -> ()
              n188 = local write "LC_Cue1_First_Count"(w331) -> ()
              n189 = local write "LC_Cue1_First_Block"(w355) -> ()
              n190 = local write "LC_ENL1_First_Tdelay"(w319) -> ()
              n191 = local write "LC_ENL1_First_OnOff"(w329) -> ()
              n192 = local write "LC_ENL1_First_Count"(w306) -> ()
              n193 = local write "LC_ENL1_First_Block"(w322) -> ()
              n194 = local write "LC_Cue1_All_Tdelay"(w324) -> ()
              n195 = local write "LC_Cue1_All_OnOff"(w330) -> ()
              n196 = local write "LC_Cue1_All_Count"(w323) -> ()
              n197 = local write "LC_Cue1_All_Block"(w327) -> ()
              n198 = local write "LC_ENL1_All_Tdelay"(w315) -> ()
              n199 = local write "LC_ENL1_All_OnOff"(w328) -> ()
              n200 = local write "LC_ENL1_All_Count"(w307) -> ()
              n201 = local write "LC_ENL1_All_Block"(w318) -> ()
            }
            frame "UploadSettings_dataLC_2" {
              # "Wrong"
              # "Reward"
              # "Trial"
              # "Tdelay"
              # "Prob"
              # "Block"
              # "OnOff"
              # "Trial"
              # "Tdelay"
              # "Prob"
              # "OnOff"
              # "Block"
              n202 = call "myRIO_BRig_RT_dataLC_Reward_Block.vi"() -> ("output_Reward_Block"=w388:i32)  [unwired: 11 in]
              n203 = call "myRIO_BRig_RT_dataLC_Reward_OnOff.vi"() -> ("output_Reward_OnOff"=w386:i32)  [unwired: 11 in]
              n204 = call "myRIO_BRig_RT_dataLC_Reward_Trial.vi"() -> ("output_Reward_Trial"=w383:i32)  [unwired: 11 in]
              n205 = call "myRIO_BRig_RT_dataLC_Wrong_Block.vi"() -> ("output_Wrong_Block"=w379:i32)  [unwired: 11 in]
              n206 = call "myRIO_BRig_RT_dataLC_Wrong_OnOff.vi"() -> ("output_Wrong_OnOff"=w378:i32)  [unwired: 11 in]
              n207 = call "myRIO_BRig_RT_dataLC_Wrong_Trial.vi"() -> ("output_Wrong_Trial"=w380:i32)  [unwired: 11 in]
              n208 = call "myRIO_BRig_RT_dataLC_Reward_Probability.vi"() -> ("output_Reward_Probability"=w385:i32)  [unwired: 11 in]
              n209 = call "myRIO_BRig_RT_dataLC_Reward_Tdelay.vi"() -> ("output_Reward_Tdelay"=w384:i32)  [unwired: 11 in]
              n210 = call "myRIO_BRig_RT_dataLC_Wrong_Probability.vi"() -> ("output_Wrong_Probability"=w382:i32)  [unwired: 11 in]
              n211 = call "myRIO_BRig_RT_dataLC_Wrong_Tdelay.vi"() -> ("output_Wrong_Tdelay"=w381:i32)  [unwired: 11 in]
              n212 = Index Array(array=w363, index #1=w388, index #2=w386, index #3=w385, index #4=w384, index #5=w383, index #6=w379, index #7=w378, index #8=w382, index #9=w381, index #10=w380) -> (element #1=w387:u16, element #2=w376:u16, element #3=w375:u16, element #4=w374:u16, element #5=w373:u16, element #6=w371:u16, element #7=w370:u16, element #8=w369:u16, element #9=w368:u16, element #10=w367:u16)
              n213 = Not Equal To 0?(x=w376) -> (x != 0?=w377:bool)
              n214 = Not Equal To 0?(x=w370) -> (x != 0?=w372:bool)
              n215 = local write "LC_Reward_Probability"(w375) -> ()
              n216 = local write "LC_Wrong_Probability"(w369) -> ()
              n217 = local write "LC_Reward_Tdelay"(w374) -> ()
              n218 = local write "LC_Reward_OnOff"(w377) -> ()
              n219 = local write "LC_Reward_Block"(w387) -> ()
              n220 = local write "LC_Reward_Trial"(w373) -> ()
              n221 = local write "LC_Wrong_Tdelay"(w368) -> ()
              n222 = local write "LC_Wrong_OnOff"(w372) -> ()
              n223 = local write "LC_Wrong_Block"(w371) -> ()
              n224 = local write "LC_Wrong_Trial"(w367) -> ()
            }
            frame "UploadSettings_dataMTrig_1" {
              # "Tdelay_R"
              # "Tdelay_L"
              # "Tcycle_R"
              # "Tcycle_L"
              # "RewCalib_nCycle_R"
              # "RewCalib_nCycle_L"
              # "Solenoid"
              # "Laser_Tcycle"
              n225 = call "myRIO_BRig_RT_dataMTrig_Laser_Tcycle.vi"() -> ("output_Laser_Tcycle"=w399:i32)  [unwired: 11 in]
              n226 = call "myRIO_BRig_RT_dataMTrig_Solenoid_RewCalib_nCycle__L.vi"() -> ("output_Solenoid_RewCalib_nCycle__L"=w398:i32)  [unwired: 11 in]
              n227 = call "myRIO_BRig_RT_dataMTrig_Solenoid_RewCalib_nCycle__R.vi"() -> ("output_Solenoid_RewCalib_nCycle__R"=w397:i32)  [unwired: 11 in]
              n228 = call "myRIO_BRig_RT_dataMTrig_Solenoid_Tdelay__L.vi"() -> ("output_Solenoid_Tdelay__L"=w394:i32)  [unwired: 11 in]
              n229 = call "myRIO_BRig_RT_dataMTrig_Solenoid_Tdelay__R.vi"() -> ("output_Solenoid_Tdelay__R"=w393:i32)  [unwired: 11 in]
              n230 = call "myRIO_BRig_RT_dataMTrig_Solenoid_Tcycle__L.vi"() -> ("output_Solenoid_Tcycle__L"=w396:i32)  [unwired: 11 in]
              n231 = call "myRIO_BRig_RT_dataMTrig_Solenoid_Tcycle__R.vi"() -> ("output_Solenoid_Tcycle__R"=w395:i32)  [unwired: 11 in]
              n232 = Index Array(array=w392, index #1=w399, index #2=w398, index #3=w397, index #4=w396, index #5=w395, index #6=w394, index #7=w393) -> (element #1=w406:u16, element #2=w405:u16, element #3=w404:u16, element #4=w403:u16, element #5=w402:u16, element #6=w401:u16, element #7=w400:u16)
              n233 = Replace Array Subset(array=w411, new element #1=w406, index #1=w399, new element #2=w405, index #2=w398, new element #3=w404, index #3=w397, new element #4=w403, index #4=w396, new element #5=w402, index #5=w395, new element #6=w401, index #6=w394, new element #7=w400, index #7=w393) -> (w410:u16[])
              n234 = local write "MTrig_Solenoid_Tcycle__L"(w403) -> ()
              n235 = local write "MTrig_Solenoid_Tcycle__R"(w402) -> ()
              n236 = local write "MTrig_Laser_Tcycle"(w406) -> ()
            }
            frame "Idle" {
              # "To ensure timing, we split the\nidle state into 4 phases"
              # "Laser_Tcycle"
              # "Audio_Tcycle_R"
              # "Audio_Tcycle_L"
              n237 = local read "MTrig_Audio_trig__L"() -> (w422:bool)
              n238 = local read "MTrig_Audio_trig__R"() -> (w424:bool)
              n239 = Select(t=myRIO_BRig_RT__Case_NonExp_stateList."SendData" ("Enum"), s="SendData", f=myRIO_BRig_RT__Case_NonExp_stateList."Idle_2" ("Enum")) -> (s? t:f=w417:T1)
              n240 = local read "MTrig_Laser_trig"() -> (w423:bool)
              n241 = call "myRIO_BRig_RT_dataMTrig_Audio_Tcycle__L.vi"() -> ("output_Audio_Tcycle__L"=w435:i32)  [unwired: 11 in]
              n242 = call "myRIO_BRig_RT_dataMTrig_Audio_Tcycle__R.vi"() -> ("output_Audio_Tcycle__R"=w434:i32)  [unwired: 11 in]
              n243 = call "myRIO_BRig_RT_dataMTrig_Laser_Tcycle.vi"() -> ("output_Laser_Tcycle"=w433:i32)  [unwired: 11 in]
              n244 = local read "MTrig_Laser_Tcycle"() -> (w415:u16)
              n245 = Select(t=myRIO_BRig_RT__Case_NonExp_stateList."TestConnection" ("Enum"), s="TestConnection", f=w417) -> (s? t:f=w426:T1)
              n246 = local read "Tcycle_Cue_min"() -> (w416:u16)
              n247 = Compound Arithmetic op=OR(w422, w424, w423) -> (w425:bool)
              n248 = case shown="True" w425 {
                frame False {
                }
                frame True {
                  w436 = FALSE
                  n249 = local write "MTrig_Audio_trig__L"(w436) -> ()
                  n250 = local write "MTrig_Audio_trig__R"(w436) -> ()
                  n251 = local write "MTrig_Laser_trig"(w436) -> ()
                }
              }
              n252 = Replace Array Subset(array=w431, new element #1=w416, index #1=w435, new element #2=w416, index #2=w434, new element #3=w415, index #3=w433) -> (w432:u16[])
              n253 = local read "Audio_Amp__R"() -> (w427:u16)
              n254 = local read "Audio_Amp__L"() -> (w428:u16)
              n255 = local read "Audio_Freq__R"() -> (w413:u8)
              n256 = local read "Audio_Freq__L"() -> (w414:u8)
            }
            frame "Idle_2" {
              w438 = u16 0 ("t")
              # "To ensure timing, we split the\nidle state into 4 phases"
              # "Ncycles"
              # "Ncycles"
              # "RewCalib"
              # "RewCalib"
              # "Solenoid R"
              # "Solenoid L"
              n257 = call "myRIO_BRig_RT_dataMTrig_Solenoid_RewCalib_OnOff__L.vi"() -> ("output_Solenoid_RewCalib_OnOff__L"=w473:i32)  [unwired: 11 in]
              n258 = call "myRIO_BRig_RT_dataMTrig_Solenoid_N__L.vi"() -> ("output_Solenoid_N__L"=w461:i32)  [unwired: 11 in]
              n259 = call "myRIO_BRig_RT_dataMTrig_Solenoid_RewCalib_OnOff__R.vi"() -> ("output_Solenoid_RewCalib_OnOff__R"=w458:i32)  [unwired: 11 in]
              n260 = call "myRIO_BRig_RT_dataMTrig_Solenoid_N__R.vi"() -> ("output_Solenoid_N__R"=w457:i32)  [unwired: 11 in]
              n261 = Index Array(array=w464, index #1=w473, index #2=w461, index #3=w458, index #4=w457) -> (element #1=w460:u16, element #2=w455:u16, element #3=w456:u16, element #4=w454:u16)
              n262 = local read "RewCalib_Trig_L"() -> (w453:bool)
              n263 = local read "RewCalib_Trig_R"() -> (w452:bool)
              n264 = Equal To 0?(x=w455) -> (x = 0?=w463:bool)
              n265 = Equal To 0?(x=w454) -> (x = 0?=w462:bool)
              n266 = Not Equal To 0?(x=w456) -> (x != 0?=w474:bool)
              n267 = Not Equal To 0?(x=w460) -> (x != 0?=w475:bool)
              n268 = And(x=w463, y=w462) -> (x .and. y?=w467:bool)
              n269 = Or(x=w453, y=w452) -> (x .or. y?=w468:bool)
              n270 = Not Exclusive Or(1:w475, 2:w453) -> (0:w470:bool)
              n271 = Not Exclusive Or(1:w474, 2:w452) -> (0:w472:bool)
              n272 = And(x=w468, y=w467) -> (x .and. y?=w450:bool)
              n273 = Not(x=w470) -> (.not. x?=w469:bool)
              n274 = Not(x=w472) -> (.not. x?=w471:bool)
              n275 = Or(x=w469, y=w471) -> (x .or. y?=w451:bool)
              n276 = Or(x=w450, y=w451) -> (x .or. y?=w466:bool)
              n277 = local read "count_warmup_R"() -> (w437:u16)
              n278 = local read "count_warmup_L"() -> (w442:u16)
              n279 = Select(t=myRIO_BRig_RT__Case_NonExp_stateList."RewardCalibration_pre" ("Enum"), s=w466, f=myRIO_BRig_RT__Case_NonExp_stateList."Idle_3" ("Enum")) -> (s? t:f=w449:T1)
              n280 = Select(t=w438, s="count_warmup_L_reset", f=w442) -> (s? t:f=→"count_warmup_L":u16)
              n281 = Select(t=w438, s="count_warmup_R_reset", f=w437) -> (s? t:f=→"count_warmup_R":u16)
            }
            frame "Idle_3" {
              w499 = u8 0 ("f")
              # "To ensure timing, we split the\nidle state into 4 phases"
              n282 = local read "MTrig_Solenoid_trig__L"() -> (w487:bool)
              n283 = local read "MTrig_Solenoid_trig__R"() -> (w500:bool)
              n284 = local read "warmupType"() -> (w477:u8)
              n285 = local read "warmup"() -> (w492:bool)
              n286 = Not Equal To 0?(x=w477) -> (x != 0?=w476:bool)
              n287 = Not(x=w476) -> (.not. x?=w493:bool)
              n288 = Select(t=u8 1, s=w487, f=w499) -> (s? t:f=w498:u8)
              n289 = Select(t=u8 2, s=w500, f=w499) -> (s? t:f=w497:u8)
              n290 = And(x=w492, y=w493) -> (x .and. y?=w491:bool)
              n291 = And(x=w492, y=w476) -> (x .and. y?=w482:bool)
              n292 = Add(x=w498, y=w497) -> (x+y=w496:u8)
              n293 = case shown="3" w496 {
                tunnel: w495 -> [w503 w507 w525 w543]
                tunnel: [w503 w506 w524 w542] -> w494
                tunnel: w491 -> [_ w505 w523 w541]
                tunnel: [_ TRUE TRUE TRUE] -> w484
                frame 0, Default {
                }
                frame 1 {
                  n294 = case shown="True" w505 {
                    tunnel: w507 -> [w516 w521]
                    tunnel: [w515 w520] -> w506
                    frame True {
                      # "Audio_L"
                      # "Solenoid_L"
                      n295 = call "myRIO_BRig_RT_dataMTrig_Solenoid_N__L.vi"() -> ("output_Solenoid_N__L"=w512:i32)  [unwired: 11 in]
                      n296 = call "myRIO_BRig_RT_dataMTrig_Audio_N__L.vi"() -> ("output_Audio_N__L"=w510:i32)  [unwired: 11 in]
                      n297 = Index Array(array=w516, index #1=w512, index #2=w510) -> (element #1=w514:u16, element #2=w513:u16)
                      n298 = Increment(x=w514) -> (x+1=w511:u16)
                      n299 = Increment(x=w513) -> (x+1=w509:u16)
                      n300 = Replace Array Subset(array=w516, new element #1=w511, index #1=w512, new element #2=w509, index #2=w510) -> (w515:u16[])
                    }
                    frame False {
                      # "Solenoid_L"
                      n301 = call "myRIO_BRig_RT_dataMTrig_Solenoid_N__L.vi"() -> ("output_Solenoid_N__L"=w518:i32)  [unwired: 11 in]
                      n302 = Index Array(array=w521, index=w518) -> (element=w519:u16)
                      n303 = Increment(x=w519) -> (x+1=w517:u16)
                      n304 = Replace Array Subset(array=w521, new element=w517, index=w518) -> (w520:u16[])
                    }
                  }
                  n305 = local write "MTrig_Solenoid_trig__L"(FALSE) -> ()
                }
                frame 2 {
                  n306 = case shown="True" w523 {
                    tunnel: w525 -> [w534 w539]
                    tunnel: [w533 w538] -> w524
                    frame True {
                      # "Audio_R"
                      # "Solenoid_R"
                      n307 = call "myRIO_BRig_RT_dataMTrig_Solenoid_N__R.vi"() -> ("output_Solenoid_N__R"=w530:i32)  [unwired: 11 in]
                      n308 = call "myRIO_BRig_RT_dataMTrig_Audio_N__R.vi"() -> ("output_Audio_N__R"=w529:i32)  [unwired: 11 in]
                      n309 = Index Array(array=w534, index #1=w530, index #2=w529) -> (element #1=w532:u16, element #2=w531:u16)
                      n310 = Increment(x=w531) -> (x+1=w527:u16)
                      n311 = Increment(x=w532) -> (x+1=w528:u16)
                      n312 = Replace Array Subset(array=w534, new element #1=w528, index #1=w530, new element #2=w527, index #2=w529) -> (w533:u16[])
                    }
                    frame False {
                      # "Solenoid_R"
                      n313 = call "myRIO_BRig_RT_dataMTrig_Solenoid_N__R.vi"() -> ("output_Solenoid_N__R"=w535:i32)  [unwired: 11 in]
                      n314 = Index Array(array=w539, index=w535) -> (element=w537:u16)
                      n315 = Increment(x=w537) -> (x+1=w536:u16)
                      n316 = Replace Array Subset(array=w539, new element=w536, index=w535) -> (w538:u16[])
                    }
                  }
                  n317 = local write "MTrig_Solenoid_trig__R"(FALSE) -> ()
                }
                frame 3 {
                  w544 = FALSE
                  n318 = case shown="True" w541 {
                    tunnel: w543 -> [w558 w566]
                    tunnel: [w557 w565] -> w542
                    frame True {
                      # "Audio_R"
                      # "Solenoid_R"
                      # "Audio_L"
                      # "Solenoid_L"
                      n319 = call "myRIO_BRig_RT_dataMTrig_Solenoid_N__L.vi"() -> ("output_Solenoid_N__L"=w552:i32)  [unwired: 11 in]
                      n320 = call "myRIO_BRig_RT_dataMTrig_Audio_N__L.vi"() -> ("output_Audio_N__L"=w550:i32)  [unwired: 11 in]
                      n321 = call "myRIO_BRig_RT_dataMTrig_Solenoid_N__R.vi"() -> ("output_Solenoid_N__R"=w548:i32)  [unwired: 11 in]
                      n322 = call "myRIO_BRig_RT_dataMTrig_Audio_N__R.vi"() -> ("output_Audio_N__R"=w547:i32)  [unwired: 11 in]
                      n323 = Index Array(array=w558, index #1=w552, index #2=w550, index #3=w548, index #4=w547) -> (element #1=w556:u16, element #2=w555:u16, element #3=w554:u16, element #4=w553:u16)
                      n324 = Increment(x=w553) -> (x+1=w545:u16)
                      n325 = Increment(x=w556) -> (x+1=w551:u16)
                      n326 = Increment(x=w555) -> (x+1=w549:u16)
                      n327 = Increment(x=w554) -> (x+1=w546:u16)
                      n328 = Replace Array Subset(array=w558, new element #1=w551, index #1=w552, new element #2=w549, index #2=w550, new element #3=w546, index #3=w548, new element #4=w545, index #4=w547) -> (w557:u16[])
                    }
                    frame False {
                      # "Solenoid_R"
                      # "Solenoid_L"
                      n329 = call "myRIO_BRig_RT_dataMTrig_Solenoid_N__L.vi"() -> ("output_Solenoid_N__L"=w562:i32)  [unwired: 11 in]
                      n330 = call "myRIO_BRig_RT_dataMTrig_Solenoid_N__R.vi"() -> ("output_Solenoid_N__R"=w559:i32)  [unwired: 11 in]
                      n331 = Index Array(array=w566, index #1=w562, index #2=w559) -> (element #1=w564:u16, element #2=w563:u16)
                      n332 = Increment(x=w564) -> (x+1=w561:u16)
                      n333 = Increment(x=w563) -> (x+1=w560:u16)
                      n334 = Replace Array Subset(array=w566, new element #1=w561, index #1=w562, new element #2=w560, index #2=w559) -> (w565:u16[])
                    }
                  }
                  n335 = local write "MTrig_Solenoid_trig__L"(w544) -> ()
                  n336 = local write "MTrig_Solenoid_trig__R"(w544) -> ()
                }
              }
              n337 = Select(t=myRIO_BRig_RT__Case_NonExp_stateList."Cue_pre", s=w482, f=myRIO_BRig_RT__Case_NonExp_stateList."DispenseWater_pre" ("Enum")) -> (s? t:f=w480:T1)
              n338 = Select(t=w480, s=w484, f=myRIO_BRig_RT__Case_NonExp_stateList."Idle_4" ("Enum")) -> (s? t:f=w485:T1)
            }
            frame "Idle_4" {
              # "use dataMTrig as it is one of the last to transfer"
              # "To ensure timing, we split the\nidle state into 4 phases"
              n339 = call "myRIO_BRig_RT_comm_webdav_uploadReceived_check_v2,0.vi"("input_dataName"="dataMTrig") -> ("output_Iexist"=w576:bool)  [unwired: 9 in, 1 out]
              n340 = Select(t=myRIO_BRig_RT__Case_NonExp_stateList."UploadSettings_pre" ("Enum"), s=w576, f=myRIO_BRig_RT__Case_NonExp_stateList."Idle") -> (s? t:f=w574:T1)
            }
            frame "Cue_pre" {
              w587 = u16 1 ("t")
              w586 = u16 0 ("new element/subarray")
              w583 = u16 0 ("new element/subarray")
              # "Ncycle"
              # "count"
              # "Audio_R"
              # "Solenoid_R"
              # "Solenoid_L"
              # "Ncycle"
              # "count"
              # "Audio_L"
              n341 = call "myRIO_BRig_RT_dataMTrig_Solenoid_N__L.vi"() -> ("output_Solenoid_N__L"=w596:i32)  [unwired: 11 in]
              n342 = call "myRIO_BRig_RT_dataMTrig_Solenoid_N__R.vi"() -> ("output_Solenoid_N__R"=w595:i32)  [unwired: 11 in]
              n343 = Index Array(array=w592, index #1=w596, index #2=w595) -> (element #1=w594:u16, element #2=w593:u16)
              n344 = Not Equal To 0?(x=w593) -> (x != 0?=w578:bool)
              n345 = Not Equal To 0?(x=w594) -> (x != 0?=w579:bool)
              n346 = Select(t=w587, s=w579, f=w586) -> (s? t:f=w588:u16)
              n347 = Select(t=w587, s=w578, f=w586) -> (s? t:f=w582:u16)
              n348 = call "myRIO_BRig_RT_dataMTrig_Audio_c__L.vi"() -> ("output_Audio_c__L"=w590:i32)  [unwired: 11 in]
              n349 = call "myRIO_BRig_RT_dataMTrig_Audio_N__L.vi"() -> ("output_Audio_N__L"=w589:i32)  [unwired: 11 in]
              n350 = call "myRIO_BRig_RT_dataMTrig_Audio_c__R.vi"() -> ("output_Audio_c__R"=w585:i32)  [unwired: 11 in]
              n351 = call "myRIO_BRig_RT_dataMTrig_Audio_N__R.vi"() -> ("output_Audio_N__R"=w584:i32)  [unwired: 11 in]
              n352 = Replace Array Subset(array=w592, new element #1=w583, index #1=w590, new element #2=w588, index #2=w589, new element #3=w583, index #3=w585, new element #4=w582, index #4=w584) -> (w591:u16[])
            }
            frame "Cue" {
              # "lick did not occur or warmupType==1"
              # "lick occurred?"
              # "Ncycle"
              # "Audio_R"
              # "Ncycle"
              # "Audio_L"
              n353 = local read "warmupType"() -> (w609:u8)
              n354 = Greater?(x=w615, y=w614) -> (0:w618:bool)
              n355 = Greater?(x=w617, y=w616) -> (0:w613:bool)
              n356 = Or(x=w613, y=w618) -> (x .or. y?=w607:bool)
              n357 = Equal?(x=w609, y=u8 1) -> (x = y?=w603:bool)
              n358 = Not(x=w607) -> (.not. x?=w606:bool)
              n359 = call "myRIO_BRig_RT_dataMTrig_Audio_N__L.vi"() -> ("output_Audio_N__L"=w622:i32)  [unwired: 11 in]
              n360 = call "myRIO_BRig_RT_dataMTrig_Audio_N__R.vi"() -> ("output_Audio_N__R"=w621:i32)  [unwired: 11 in]
              n361 = Or(x=w606, y=w603) -> (x .or. y?=w604:bool)
              n362 = case shown="True" w604 {
                tunnel: w622 -> [w631 w649]
                tunnel: w621 -> [w630 w648]
                tunnel: w612 -> [w633 w643]
                tunnel: [w632 w643] -> w611
                tunnel: w610 -> [_ w641]
                tunnel: [myRIO_BRig_RT__Case_NonExp_stateList."Idle" ("t") w640] -> w605
                tunnel: w603 -> [_ w639]
                tunnel: w602 -> [_ w635]
                tunnel: w601 -> [_ w634]
                frame False {
                  w626 = u16 0 ("new element/subarray")
                  # "lick occurred and warmupType==2"
                  n363 = call "myRIO_BRig_RT_dataMTrig_Solenoid_N__R.vi"() -> ("output_Solenoid_N__R"=w627:i32)  [unwired: 11 in]
                  n364 = call "myRIO_BRig_RT_dataMTrig_Solenoid_N__L.vi"() -> ("output_Solenoid_N__L"=w628:i32)  [unwired: 11 in]
                  n365 = Replace Array Subset(array=w633, new element #1=w626, index #1=w631, new element #2=w626, index #2=w630, new element #3=w626, index #3=w628, new element #4=w626, index #4=w627) -> (w632:u16[])
                }
                frame True {
                  n366 = Not(x=w639) -> (.not. x?=w638:bool)
                  n367 = Index Array(array=w643, index #1=w649, index #2=w648) -> (element #1=w647:u16, element #2=w646:u16)
                  n368 = Equal To 0?(x=w647) -> (x = 0?=w645:bool)
                  n369 = Equal To 0?(x=w646) -> (x = 0?=w644:bool)
                  n370 = And(x=w645, y=w644) -> (x .and. y?=w637:bool)
                  n371 = And(x=w637, y=w638) -> (x .and. y?=w636:bool)
                  n372 = case shown="True" w636 {
                    tunnel: w635 -> [_ w657]
                    tunnel: w634 -> [_ w652]
                    frame False {
                    }
                    frame True {
                      n373 = local read "count_warmup_R"() -> (w650:u16)
                      n374 = local read "count_warmup_L"() -> (w655:u16)
                      n375 = Increment(x=w650) -> (x+1=w653:u16)
                      n376 = Increment(x=w655) -> (x+1=w656:u16)
                      n377 = Select(t=w653, s=w652, f=w650) -> (s? t:f=w651:u16)
                      n378 = Select(t=w656, s=w657, f=w655) -> (s? t:f=w654:u16)
                      n379 = local write "count_warmup_R"(w651) -> ()
                      n380 = local write "count_warmup_L"(w654) -> ()
                    }
                  }
                  n381 = Select(t=myRIO_BRig_RT__Case_NonExp_stateList."DispenseWater_pre", s=w637, f=w641) -> (s? t:f=w640:T1)
                }
              }
            }
            frame "RewardCalibration_pre" {
              (unwired) FALSE
              w663 = FALSE
              w674 = u8 0
              w690 = u8 0
              # "Are we starting a RewardCalibration?\nOr are we stopping a RewardCalibration?\nOr is a RewardCalibration over?"
              # "RewCalib\nOnOff"
              # "N"
              # "Solenoid R"
              # "RewCalib\nOnOff"
              # "N"
              # "Solenoid L"
              n382 = local read "RewCalib_Trig_L"() -> (w697:bool)
              n383 = local read "RewCalib_Trig_R"() -> (w666:bool)
              n384 = call "myRIO_BRig_RT_dataMTrig_Solenoid_N__R.vi"() -> ("output_Solenoid_N__R"=w668:i32)  [unwired: 11 in]
              n385 = call "myRIO_BRig_RT_dataMTrig_Solenoid_RewCalib_OnOff__R.vi"() -> ("output_Solenoid_RewCalib_OnOff__R"=w665:i32)  [unwired: 11 in]
              n386 = call "myRIO_BRig_RT_dataMTrig_Solenoid_N__L.vi"() -> ("output_Solenoid_N__L"=w683:i32)  [unwired: 11 in]
              n387 = call "myRIO_BRig_RT_dataMTrig_Solenoid_RewCalib_OnOff__L.vi"() -> ("output_Solenoid_RewCalib_OnOff__L"=w684:i32)  [unwired: 11 in]
              n388 = Index Array(array=w667, index #1=w668, index #2=w665) -> (element #1=w678:u16, element #2=w673:u16)
              n389 = Index Array(array=w667, index #1=w683, index #2=w684) -> (element #1=w694:u16, element #2=w689:u16)
              n390 = Equal To 0?(x=w678) -> (x = 0?=w679:bool)
              n391 = Not Equal To 0?(x=w673) -> (x != 0?=w676:bool)
              n392 = Equal To 0?(x=w694) -> (x = 0?=w695:bool)
              n393 = Not Equal To 0?(x=w689) -> (x != 0?=w692:bool)
              n394 = local write "MTrig_Solenoid_trig__L"(w663) -> ()
              n395 = local write "MTrig_Solenoid_trig__R"(w663) -> ()
              n396 = Select(t=u8 1, s=w666, f=w674) -> (s? t:f=w670:u8)
              n397 = Select(t=u8 1, s=w697, f=w690) -> (s? t:f=w686:u8)
              n398 = Select(t=u8 2, s=w679, f=w674) -> (s? t:f=w671:u8)
              n399 = Select(t=u8 4, s=w676, f=w674) -> (s? t:f=w672:u8)
              n400 = Select(t=u8 2, s=w695, f=w690) -> (s? t:f=w687:u8)
              n401 = Select(t=u8 4, s=w692, f=w690) -> (s? t:f=w688:u8)
              n402 = Compound Arithmetic op=ADD(w670, w671, w672) -> (w669:u8)
              n403 = Compound Arithmetic op=ADD(w686, w687, w688) -> (w685:u8)
              n404 = case shown="7" w685 {
                tunnel: w667 -> [w727 w732 w734 w739 w744 w746 w749 w754]
                tunnel: [w727 w733 w734 w740 w745 w746 w750 w755] -> w682
                tunnel: w684 -> [_ w730 _ w737 w742 _ w748 w753]
                tunnel: w683 -> [_ w731 _ w738 w743 _ _ _]
                frame 0, Default {
                }
                frame 1 {
                  n405 = Replace Array Subset(array=w732, new element #1=u16 100 ("new element/subarray"), index #1=w731, new element #2=u16 1 ("new element/subarray"), index #2=w730) -> (w733:u16[])
                }
                frame 2 {
                }
                frame 3 {
                  n406 = Replace Array Subset(array=w739, new element #1=u16 100 ("new element/subarray"), index #1=w738, new element #2=u16 1 ("new element/subarray"), index #2=w737) -> (w740:u16[])
                }
                frame 4 {
                  w741 = u16 0 ("new element/subarray")
                  n407 = Replace Array Subset(array=w744, new element #1=w741, index #1=w743, new element #2=w741, index #2=w742) -> (w745:u16[])
                }
                frame 5 {
                }
                frame 6 {
                  n408 = Replace Array Subset(array=w749, new element=u16 0 ("new element/subarray"), index=w748) -> (w750:u16[])
                }
                frame 7 {
                  n409 = local write "RewCalib_Trig_L"(FALSE ("RewCalib_Trig_L")) -> ()
                  n410 = Replace Array Subset(array=w754, new element=u16 0 ("new element/subarray"), index=w753) -> (w755:u16[])
                }
              }
              n411 = case shown="7" w669 {
                tunnel: w682 -> [w698 w703 w705 w710 w715 w717 w720 w725]
                tunnel: [w698 w704 w705 w711 w716 w717 w721 w726] -> w681
                tunnel: w665 -> [_ w701 _ w708 w713 _ w719 w724]
                tunnel: w668 -> [_ w702 _ w709 w714 _ _ _]
                frame 0, Default {
                }
                frame 1 {
                  n412 = Replace Array Subset(array=w703, new element #1=u16 100 ("new element/subarray"), index #1=w702, new element #2=u16 1 ("new element/subarray"), index #2=w701) -> (w704:u16[])
                }
                frame 2 {
                }
                frame 3 {
                  n413 = Replace Array Subset(array=w710, new element #1=u16 100 ("new element/subarray"), index #1=w709, new element #2=u16 1 ("new element/subarray"), index #2=w708) -> (w711:u16[])
                }
                frame 4 {
                  w712 = u16 0 ("new element/subarray")
                  n414 = Replace Array Subset(array=w715, new element #1=w712, index #1=w714, new element #2=w712, index #2=w713) -> (w716:u16[])
                }
                frame 5 {
                }
                frame 6 {
                  n415 = Replace Array Subset(array=w720, new element=u16 0 ("new element/subarray"), index=w719) -> (w721:u16[])
                }
                frame 7 {
                  n416 = local write "RewCalib_Trig_R"(FALSE ("RewCalib_Trig_L")) -> ()
                  n417 = Replace Array Subset(array=w725, new element=u16 0 ("new element/subarray"), index=w724) -> (w726:u16[])
                }
              }
            }
            frame "DispenseWater_pre" {
              w763 = u16 0 ("t")
              w806 = u16 0 ("new element/subarray")
              # "just trust me on this one"
              # "RewCalib\nOnOff"
              # "RewCalib\nOnOff"
              # "nCycle"
              # "Solenoid__R"
              # "Tdelay"
              # "delay"
              # "nCycle"
              # "Solenoid__L"
              # "Tdelay"
              # "delay"
              # "Solenoid__R"
              # "count"
              # "Solenoid_Tcycle_R"
              # "Solenoid_Tcycle_L"
              # "Solenoid__L"
              # "count"
              n418 = call "myRIO_BRig_RT_dataMTrig_Solenoid_RewCalib_OnOff__L.vi"() -> ("output_Solenoid_RewCalib_OnOff__L"=w770:i32)  [unwired: 11 in]
              n419 = call "myRIO_BRig_RT_dataMTrig_Solenoid_N__L.vi"() -> ("output_Solenoid_N__L"=w761:i32)  [unwired: 11 in]
              n420 = call "myRIO_BRig_RT_dataMTrig_Solenoid_delay__L.vi"() -> ("output_Solenoid_delay__L"=w804:i32)  [unwired: 11 in]
              n421 = call "myRIO_BRig_RT_dataMTrig_Solenoid_Tdelay__L.vi"() -> ("output_Solenoid_Tdelay__L"=w803:i32)  [unwired: 11 in]
              n422 = call "myRIO_BRig_RT_dataMTrig_Solenoid_N__R.vi"() -> ("output_Solenoid_N__R"=w759:i32)  [unwired: 11 in]
              n423 = call "myRIO_BRig_RT_dataMTrig_Solenoid_delay__R.vi"() -> ("output_Solenoid_delay__R"=w793:i32)  [unwired: 11 in]
              n424 = call "myRIO_BRig_RT_dataMTrig_Solenoid_Tdelay__R.vi"() -> ("output_Solenoid_Tdelay__R"=w792:i32)  [unwired: 11 in]
              n425 = call "myRIO_BRig_RT_dataMTrig_Solenoid_RewCalib_OnOff__R.vi"() -> ("output_Solenoid_RewCalib_OnOff__R"=w766:i32)  [unwired: 11 in]
              n426 = Index Array(array=w805, index #1=w761, index #2=w804, index #3=w803, index #4=w759, index #5=w793, index #6=w792, index #7=w770, index #8=w766) -> (element #1=w762:u16, element #2=w802:u16, element #3=w797:u16, element #4=w765:u16, element #5=w787:u16, element #6=w786:u16, element #7=w771:u16, element #8=w768:u16)
              n427 = Equal To 0?(x=w802) -> (x = 0?=w801:bool)
              n428 = Equal To 0?(x=w787) -> (x = 0?=w791:bool)
              n429 = local read "RewCalib_Trig_L"() -> (w782:bool)
              n430 = local read "RewCalib_Trig_R"() -> (w777:bool)
              n431 = Not Equal To 0?(x=w762) -> (x != 0?=w800:bool)
              n432 = Not Equal To 0?(x=w765) -> (x != 0?=w790:bool)
              n433 = local read "MTrig_Solenoid_Tcycle__L"() -> (w799:u16)
              n434 = local read "MTrig_Solenoid_Tcycle__R"() -> (w785:u16)
              n435 = Not Equal To 0?(x=w771) -> (x != 0?=w781:bool)
              n436 = Not Equal To 0?(x=w768) -> (x != 0?=w779:bool)
              n437 = Not(x=w782) -> (.not. x?=w780:bool)
              n438 = Not(x=w777) -> (.not. x?=w778:bool)
              n439 = And(x=w781, y=w780) -> (x .and. y?=w776:bool)
              n440 = And(x=w779, y=w778) -> (x .and. y?=w775:bool)
              n441 = call "myRIO_BRig_RT_dataMTrig_Solenoid_c__L.vi"() -> ("output_Solenoid_c__L"=w808:i32)  [unwired: 11 in]
              n442 = call "myRIO_BRig_RT_dataMTrig_Solenoid_c__R.vi"() -> ("output_Solenoid_c__R"=w807:i32)  [unwired: 11 in]
              n443 = Select(t=w799, s=w800, f=u16 0) -> (s? t:f=w796:u16)
              n444 = Or(x=w776, y=w775) -> (x .or. y?=w764:bool)
              n445 = Select(t=w785, s=w790, f=u16 0) -> (s? t:f=w788:u16)
              n446 = Select(t=w796, s=w801, f=w797) -> (s? t:f=w794:u16)
              n447 = Select(t=w788, s=w791, f=w786) -> (s? t:f=w783:u16)
              n448 = call "myRIO_BRig_RT_dataMTrig_Solenoid_Tcycle__L.vi"() -> ("output_Solenoid_Tcycle__L"=w795:i32)  [unwired: 11 in]
              n449 = call "myRIO_BRig_RT_dataMTrig_Solenoid_Tcycle__R.vi"() -> ("output_Solenoid_Tcycle__R"=w784:i32)  [unwired: 11 in]
              n450 = Select(t=w763, s=w764, f=w762) -> (s? t:f=w760:u16)
              n451 = Select(t=w763, s=w764, f=w765) -> (s? t:f=w758:u16)
              n452 = Select(t=myRIO_BRig_RT__Case_NonExp_stateList."Idle" ("Enum"), s=w764, f=myRIO_BRig_RT__Case_NonExp_stateList."DispenseWater" ("Enum")) -> (s? t:f=w772:T1)
              n453 = Select(t=w763, s=w764, f=w771) -> (s? t:f=w769:u16)
              n454 = Select(t=w763, s=w764, f=w768) -> (s? t:f=w767:u16)
              n455 = Replace Array Subset(array=w805, new element #1=w806, index #1=w808, new element #2=w806, index #2=w807, new element #3=w794, index #3=w795, new element #4=w783, index #4=w784, new element #5=w769, index #5=w770, new element #6=w767, index #6=w766, new element #7=w760, index #7=w761, new element #8=w758, index #8=w759) -> (w809:u16[])
            }
            frame "DispenseWater" {
              # "D"
              # "C"
              # "B"
              # "A"
              # "(A) Add COUNT and INCREMENT\n(B) Is (A) smaller than Tcycle?\n(C) Are we dispensing water or in the delay phase?\n(D) If (A) is smaller than Tcycle   AND   if we are dispensing water\n      then send TRUE to solenoid"
              # "delay"
              # "Tcycle"
              # "Solenoid__R"
              # "count"
              # "delay"
              # "Tcycle"
              # "Solenoid__L"
              # "count"
              n456 = To Unsigned Word Integer(number=w841) -> (unsigned 16bit integer=w823:u16)
              n457 = call "myRIO_BRig_RT_dataMTrig_Solenoid_delay__R.vi"() -> ("output_Solenoid_delay__R"=w827:i32)  [unwired: 11 in]
              n458 = call "myRIO_BRig_RT_dataMTrig_Solenoid_c__R.vi"() -> ("output_Solenoid_c__R"=w826:i32)  [unwired: 11 in]
              n459 = call "myRIO_BRig_RT_dataMTrig_Solenoid_Tcycle__R.vi"() -> ("output_Solenoid_Tcycle__R"=w828:i32)  [unwired: 11 in]
              n460 = call "myRIO_BRig_RT_dataMTrig_Solenoid_delay__L.vi"() -> ("output_Solenoid_delay__L"=w843:i32)  [unwired: 11 in]
              n461 = call "myRIO_BRig_RT_dataMTrig_Solenoid_c__L.vi"() -> ("output_Solenoid_c__L"=w835:i32)  [unwired: 11 in]
              n462 = call "myRIO_BRig_RT_dataMTrig_Solenoid_Tcycle__L.vi"() -> ("output_Solenoid_Tcycle__L"=w844:i32)  [unwired: 11 in]
              n463 = Index Array(array=w837, index #1=w835, index #2=w844, index #3=w843, index #4=w826, index #5=w828, index #6=w827) -> (element #1=w842:u16, element #2=w832:u16, element #3=w840:u16, element #4=w822:u16, element #5=w819:u16, element #6=w818:u16)
              n464 = Add(x=w842, y=w823) -> (x+y=w833:u16)
              n465 = Add(x=w822, y=w823) -> (x+y=w824:u16)
              n466 = Less?(x=w833, y=w832) -> (x < y?=w816:bool)
              n467 = Equal To 0?(x=w840) -> (x = 0?=w839:bool)
              n468 = Less?(x=w824, y=w819) -> (x < y?=w817:bool)
              n469 = Equal To 0?(x=w818) -> (x = 0?=w825:bool)
              n470 = And(x=w816, y=w839) -> (x .and. y?=w838:bool)
              n471 = Or(x=w816, y=w817) -> (x .or. y?=w815:bool)
              n472 = And(x=w817, y=w825) -> (x .and. y?=w820:bool)
              n473 = Select(t=w833, s=w816, f=w832) -> (s? t:f=w834:u16)
              n474 = Select(t=w824, s=w817, f=w819) -> (s? t:f=w821:u16)
              n475 = Replace Array Subset(array=w837, new element #1=w834, index #1=w835, new element #2=w821, index #2=w826) -> (w836:u16[])
              n476 = Select(t=w831, s=w815, f=myRIO_BRig_RT__Case_NonExp_stateList."DispenseWater_post" ("Enum")) -> (s? t:f=w829:T1)
            }
            frame "DispenseWater_post" {
              # "nCycle"
              # "delay"
              # "Solenoid__R"
              # "nCycle"
              # "delay"
              # "Solenoid__L"
              n477 = call "myRIO_BRig_RT_dataMTrig_Solenoid_N__L.vi"() -> ("output_Solenoid_N__L"=w866:i32)  [unwired: 11 in]
              n478 = call "myRIO_BRig_RT_dataMTrig_Solenoid_delay__L.vi"() -> ("output_Solenoid_delay__L"=w865:i32)  [unwired: 11 in]
              n479 = call "myRIO_BRig_RT_dataMTrig_Solenoid_N__R.vi"() -> ("output_Solenoid_N__R"=w862:i32)  [unwired: 11 in]
              n480 = call "myRIO_BRig_RT_dataMTrig_Solenoid_delay__R.vi"() -> ("output_Solenoid_delay__R"=w861:i32)  [unwired: 11 in]
              n481 = Index Array(array=w868, index #1=w866, index #2=w865, index #3=w862, index #4=w861) -> (element #1=w870:u16, element #2=w869:u16, element #3=w853:u16, element #4=w855:u16)
              n482 = Not Equal To 0?(x=w870) -> (x != 0?=w871:bool)
              n483 = Not Equal To 0?(x=w853) -> (x != 0?=w854:bool)
              n484 = case shown="True" w854 {
                selector: w854 -> [_ w878]
                tunnel: w853 -> [w876 w884]
                tunnel: w855 -> [_ w885]
                tunnel: [w876 w882] -> w852
                tunnel: [u16 0 w881] -> w851
                tunnel: [_ w878] -> w850
                frame False {
                }
                frame True {
                  n485 = Equal To 0?(x=w885) -> (x = 0?=w877:bool)
                  n486 = Decrement(x=w884) -> (x-1=w883:u16)
                  n487 = Select(t=w883, s=w877, f=w884) -> (s? t:f=w882:u16)
                  n488 = Select(t=u16 1, s=w877, f=u16 0) -> (s? t:f=w881:u16)
                }
              }
              n489 = case shown="True" w871 {
                selector: w871 -> [_ w889]
                tunnel: w870 -> [w887 w895]
                tunnel: w869 -> [_ w896]
                tunnel: [w887 w893] -> w864
                tunnel: [u16 0 w892] -> w863
                tunnel: [_ w889] -> w860
                frame False {
                }
                frame True {
                  n490 = Equal To 0?(x=w896) -> (x = 0?=w888:bool)
                  n491 = Decrement(x=w895) -> (x-1=w894:u16)
                  n492 = Select(t=w894, s=w888, f=w895) -> (s? t:f=w893:u16)
                  n493 = Select(t=u16 1, s=w888, f=u16 0) -> (s? t:f=w892:u16)
                }
              }
              n494 = Or(x=w860, y=w850) -> (x .or. y?=w859:bool)
              n495 = Replace Array Subset(array=w868, new element #1=w864, index #1=w866, new element #2=w863, index #2=w865, new element #3=w852, index #3=w862, new element #4=w851, index #4=w861) -> (w867:u16[])
              n496 = Select(t=myRIO_BRig_RT__Case_NonExp_stateList."DispenseWater_pre" ("Enum"), s=w859, f=myRIO_BRig_RT__Case_NonExp_stateList."Idle" ("Enum")) -> (s? t:f=w856:T1)
            }
            frame "TestConnection" {
              n497 = local read "Host Password"() -> (w907:string)
              n498 = local read "Host UserName"() -> (w908:string)
              n499 = call "myRIO_BRig_RT_comm_webdav_testConnect.vi"("input_password"=w907, "input_username"=w908) -> ("output_Iconnected"=w905:bool)  [unwired: 9 in]
              n500 = Select(t="Connection accepted!" ("message"), s=w905, f="Error!") -> (s? t:f=w903:string)
              n501 = One Button Dialog(message=w903) -> ()  [unwired: 1 in, 1 out]
            }
            frame "SendData" {
              n502 = local read "Host Filename Prefix"() -> (w911:string)
              n503 = local read "Host Password"() -> (w912:string)
              n504 = local read "Host UserName"() -> (w913:string)
              n505 = call "myRIO_BRig_RT_comm_webdav_sendData_all.vi"("Host Filename Prefix"=w911, "Host Password"=w912, "Host UserName"=w913) -> ()  [unwired: 9 in]
            }
            frame "End" {
            }
          }
          n506 = local read "MTrig_Audio_trig__R"() -> (w91:bool)
          n507 = local read "MTrig_Audio_trig__L"() -> (w90:bool)
          n508 = local read "START"() -> (w86:bool)
          n509 = local read "STOP_abort"() -> (w85:bool)
          n510 = local read "MTrig_Laser_trig"() -> (w92:bool)
          n511 = call "myRIO_BRig_RT_dataMTrig_main__v2.vi"("input_dataMTrig"=w94, "input_Audio_trig_L"=w90, "input_Audio_trig_R"=w91, "input_Laser_trig"=w92) -> ("output_dataMTrig"=w93:u16[], "output_Audio_L"=w70:bool, "output_Audio_R"=w81:bool, "output_Laser"=w73:bool)  [unwired: 12 in]
          n512 = Or(x=w86, y=w85) -> (x .or. y?=w84:bool)
          n513 = Select(t=myRIO_BRig_RT__Case_NonExp_stateList."End" ("Enum"), s=w84, f=w83) -> (s? t:f=w82:T1)
          n514 = Or(x=w91, y=w92) -> (x .or. y?=w89:bool)
          n515 = Or(x=w89, y=w90) -> (x .or. y?=w88:bool)
          n516 = case shown="True" w88 {
            frame False {
            }
            frame True {
              w112 = FALSE
              n517 = local write "MTrig_Audio_trig__R"(w112) -> ()
              n518 = local write "MTrig_Audio_trig__L"(w112) -> ()
              n519 = local write "MTrig_Laser_trig"(w112) -> ()
            }
          }
          n520 = xnode "Read/Write Control"("FPGA VI Reference In"=w106, "error in"=w104, "A1_SR"=w95, "A3_SL"=w96, "audioTrigger_L"=w70, "audioAmp_L"=w63, "audioFreq_L_kHz"=w65, "audioTrigger_R"=w81, "audioAmp_R"=w64, "audioFreq_R_kHz"=w66, "laserResponse_reward_LED"="laserResponse_reward_LED", "laserResponse_wrong_LED"="laserResponse_wrong_LED", "laserResponse_reward"="laserResponse_reward", "laserResponse_wrong"="laserResponse_wrong", "SelectionState"="SelectionState", "ignoreWrong"="ignoreWrong", "Left(F)_or_Right(T)"="Left(F)_or_Right(T)", "laserMTrig"=w73) -> ("FPGA VI Reference Out"=w105:refnum<k20>, "error out"=w103:errorcluster, "SelectReward"=→"SelectReward":bool, "SelectWrong"=→"SelectWrong":bool)
          n521 = node-c288() -> ()  [unwired: 1 in, 1 out]
          "cState_NonExp" <- w102
        }
        n522 = node-c288(w50) -> ()  [unwired: 1 out]
        n523 = flat-sequence {
          tunnel: w43 -> [w54]
          tunnel: [w54] -> w42
          tunnel: w41 -> [w53]
          tunnel: [w53] -> w40
          frame #0 {
            w52 = FALSE
            n524 = local write "STOP_endBlock"(w52) -> ()
            n525 = local write "STOP_endTrial"(w52) -> ()
          }
        }
      }
      frame True {
        w933 = u8 0
        w935 = FALSE ("SelectionState")
        w940 = u16 0 ("idxDataBlock")
        w942 = u16 100 ("new element/subarray")
        w943 = u16 100 ("new element/subarray")
        w963 = T6 refnum items=["Session NI_WebDAV"] ("output_hSession")
        w972 = FALSE
        w973 = u16 0
        w934 = FALSE
        # "audio__L\naudio__R"
        # "Audio params"
        # "nRewards"
        # "idxDataBlock"
        # "Solenoid_Tdelay_R"
        # "Solenoid_Tdelay_L"
        # "RewCalib_N__R"
        # "RewCalib_N__L"
        # "Save dataLick to file\nSend file to Host\nSave dataMTrig\nSend file to Host\nDisconnect"
        # "dataTrial"
        # "dataTrial"
        # "Solenoid_Tcycle_R"
        # "Solenoid_Tcycle_L"
        # "Laser_Tcycle"
        # "Audio_Tcycle_R"
        # "Audio_Tcycle_L"
        # "dataLick"
        # "dataLC"
        # "dataLC"
        # "dataBlock"
        # "dataBlock"
        # "dataMTrig"
        # "dataMTrig"
        # "dataExp"
        # "dataCurrent"
        # "dataExp"
        # "dataCurrent"
        # "spout"
        # "state"
        n526 = call "myRIO_BRig_RT_dataMTrig_Solenoid_Tcycle__L.vi"() -> ("output_Solenoid_Tcycle__L"=w969:i32)  [unwired: 11 in]
        n527 = call "myRIO_BRig_RT_dataMTrig_Solenoid_Tcycle__R.vi"() -> ("output_Solenoid_Tcycle__R"=w968:i32)  [unwired: 11 in]
        n528 = call "myRIO_BRig_RT_dataMTrig_Audio_Tcycle__L.vi"() -> ("output_Audio_Tcycle__L"=w967:i32)  [unwired: 11 in]
        n529 = call "myRIO_BRig_RT_dataMTrig_Audio_Tcycle__R.vi"() -> ("output_Audio_Tcycle__R"=w966:i32)  [unwired: 11 in]
        n530 = call "myRIO_BRig_RT_dataMTrig_Laser_Tcycle.vi"() -> ("output_Laser_Tcycle"=w965:i32)  [unwired: 11 in]
        n531 = local read "MTrig_Solenoid_Tcycle__L"() -> (w948:u16)
        n532 = local read "MTrig_Solenoid_Tcycle__R"() -> (w947:u16)
        n533 = local read "Tcycle_Reward_L"() -> (w944:u16)
        n534 = local read "Tcycle_Reward_R"() -> (w945:u16)
        n535 = local read "MTrig_Laser_Tcycle"() -> (w946:u16)
        n536 = call "myRIO_BRig_RT_dataMTrig_Solenoid_RewCalib_nCycle__L.vi"() -> ("output_Solenoid_RewCalib_nCycle__L"=w951:i32)  [unwired: 11 in]
        n537 = call "myRIO_BRig_RT_dataMTrig_Solenoid_Tdelay__L.vi"() -> ("output_Solenoid_Tdelay__L"=w953:i32)  [unwired: 11 in]
        n538 = call "myRIO_BRig_RT_dataMTrig_Solenoid_RewCalib_nCycle__R.vi"() -> ("output_Solenoid_RewCalib_nCycle__R"=w952:i32)  [unwired: 11 in]
        n539 = call "myRIO_BRig_RT_dataMTrig_Solenoid_Tdelay__R.vi"() -> ("output_Solenoid_Tdelay__R"=w954:i32)  [unwired: 11 in]
        n540 = call "myRIO_BRig_RT_dataLick_init.vi"() -> ("output_dataLick"=w975:u16[][])  [unwired: 11 in]
        n541 = call "myRIO_BRig_RT_dataCurrent_init.vi"() -> ("output_dataCurrent"=w982:u16[])  [unwired: 11 in]
        n542 = call "myRIO_BRig_RT_dataExp_init.vi"() -> ("output_dataExp"=w981:u16[])  [unwired: 11 in]
        n543 = call "myRIO_BRig_RT_dataMTrig_init.vi"() -> ("output_dataMTrig"=w971:u16[])  [unwired: 5 in]
        n544 = call "myRIO_BRig_RT_dataLC_init.vi"() -> ("output_dataLC"=w979:u16[])  [unwired: 11 in]
        n545 = call "myRIO_BRig_RT_dataBlock_init.vi"() -> ("output_dataBlock"=w980:u16[][])  [unwired: 11 in]
        n546 = call "myRIO_BRig_RT_dataTrial_init.vi"() -> ("output_dataTrial"=w964:u16[][])  [unwired: 11 in]
        n547 = xnode "Read/Write Control"("FPGA VI Reference In"=w936, "error in"=w937, "SelectionState"=w935, "laserResponse_reward"=w935, "laserResponse_wrong"=w935, "laserResponse_reward_LED"=w935, "laserResponse_wrong_LED"=w935, "Left(F)_or_Right(T)"=w935, "ignoreWrong"=w935, "SelectionState"=w935) -> ("FPGA VI Reference Out"=w938:refnum<k20>, "error out"=w939:errorcluster)
        n548 = Replace Array Subset(array=w971, new element #1=w943, index #1=w951, new element #2=w943, index #2=w952, new element #3=w942, index #3=w953, new element #4=w942, index #4=w954, new element #5=w948, index #5=w969, new element #6=w947, index #6=w968, new element #7=w944, index #7=w967, new element #8=w945, index #8=w966, new element #9=w946, index #9=w965) -> (w970:u16[])
        n549 = Get Date/Time In Seconds() -> (seconds since 1Jan1904=w950:timestamp)
        n550 = To Double Precision Float(number=w950) -> (double precision float=w949:dbl)
        n551 = node-c288() -> (w990:T3)  [unwired: 4 in]
        n552 = timed-loop {
          timing: w990 -> [_]
          timing-out: [_] -> w989
          shift-right: [w1069] -> _
          shift-left: myRIO_BRig_RT__Case_Exp_stateList."Start1" ("Enum") -> [w1100]
          shift-right: [w1121] -> _
          shift-left: enum16{"Left", "Right"}."Left" -> [w1123]
          tunnel: w938 -> [w1120]
          tunnel: w939 -> [w1119]
          shift-right: [w1114] -> _
          shift-left: w987 -> [w1118]
          shift-right: [w1113] -> _
          shift-left: w986 -> [w1117]
          tunnel: [w1094] -> w984
          tunnel: [w1095] -> w985
          shift-right: [w1096] -> w955
          shift-left: w982 -> [w1061]
          shift-right: [w1112] -> _
          shift-left: w981 -> [w1056]
          shift-right: [w1083] -> w959
          shift-left: w970 -> [w1084]
          shift-right: [w1110] -> _
          shift-left: w980 -> [w1111]
          shift-right: [w1108] -> _
          shift-left: w979 -> [w1109]
          shift-right: [w1042] -> _
          shift-left: w934 -> [w1107]
          shift-right: [w1098] -> w961
          shift-left: w975 -> [w1099]
          shift-right: [w1085] -> _
          shift-left: w973 -> [w1093]
          shift-right: [w1053] -> _
          shift-left: w933 -> [w1092]
          shift-right: [w1086] -> _
          shift-left: w973 -> [w1091]
          shift-right: [w1087] -> _
          shift-left: w933 -> [w1090]
          shift-right: [w1054] -> _
          shift-left: w972 -> [w1088]
          shift-right: [w1055] -> _
          shift-left: w972 -> [w1089]
          shift-right: [w1067] -> _
          shift-left: w964 -> [w1068]
          shift-right: [w1066] -> w957
          shift-left: w963 -> [w1064]
          shift-right: [w1065] -> w958
          shift-left: FALSE ("output_Iconnected") -> [w1063]
          tunnel: "Host Filename Prefix" -> [w1062]
          tunnel: [w1062] -> w956
          shift-right: [w1037] -> _
          shift-left: w934 -> [w1060]
          tunnel: w949 -> [w1057]
          shift-right: [w1051] -> _
          shift-left: 0 ("idxDataBlock") -> [w1052]
          shift-right: [w1048] -> _
          shift-left: w940 -> [w1050]
          shift-right: [w1047] -> _
          shift-left: w940 -> [w1049]
          shift-right: [w1036] -> _
          shift-left: w934 -> [w1043]
          shift-right: [w1039] -> _
          shift-left: w934 -> [w1041]
          shift-right: [w1038] -> _
          shift-left: w934 -> [w1040]
          shift-right: [w1029] -> _
          shift-left: w934 -> [w1030]
          stop <- w1106 stop-if-true
          # "Laser"
          # "Audio R"
          # "Audio L"
          # "Solenoid R"
          # "Solenoid L"
          # "manual triggering"
          # "dataTrial"
          # "dataBlock"
          # "nRewards"
          # "laserOccurred"
          # "dataExp"
          # "dataCurrent"
          # "audio__L\naudio__R"
          # "time stamp"
          # "Audio params"
          # "nRewards"
          # "idxDataBlock"
          # "idxDataBlock"
          # "activate"
          # "audio__L\naudio__R"
          # "amp__R\nfreq__R"
          # "amp__L\nfreq__L"
          # "dataLC"
          # "solenoid__R"
          # "solenoid__L"
          # "Did a lick occur?"
          # "Update lick counter"
          # "spout"
          # "spout"
          # "state"
          # "state"
          n553 = node-c288() -> ()  [unwired: 1 in, 1 out]
          n554 = local read "MTrig_Solenoid_trig__L"() -> (w1081:bool)
          n555 = local read "MTrig_Solenoid_trig__R"() -> (w1080:bool)
          n556 = local read "MTrig_Audio_trig__L"() -> (w1079:bool)
          n557 = local read "MTrig_Audio_trig__R"() -> (w1078:bool)
          n558 = xnode "Read/Write Control"("FPGA VI Reference In"=w1120, "error in"=w1119) -> ("FPGA VI Reference Out"=w1046:refnum<k20>, "error out"=w1045:errorcluster, "A2_LickL"=w1114:u32, "A4_LickR"=w1113:u32)
          "A2" <- w1114
          "A4" <- w1113
          n559 = local read "MTrig_Laser_trig"() -> (w1077:bool)
          n560 = Greater?(x=w1114, y=w1118) -> (0:w1116:bool)
          n561 = Greater?(x=w1113, y=w1117) -> (0:w1115:bool)
          n562 = Or(x=w1116, y=w1115) -> (x .or. y?=w1122:bool)
          n563 = call "myRIO_BRig_RT_dataMTrig_main.vi"("input_dataMTrig"=w1084, "input_Solenoid_trig_L"=w1081, "input_Solenoid_trig_R"=w1080, "input_Audio_trig_L"=w1079, "input_Audio_trig_R"=w1078, "input_Laser_trig"=w1077) -> ("output_Laser"=w1034:bool, "output_dataMTrig"=w1083:u16[], "output_Solenoid_L"=w1071:bool, "output_Solenoid_R"=w1073:bool, "output_Audio_L"=w1075:bool, "output_Audio_R"=w1076:bool)  [unwired: 8 in]
          n564 = Compound Arithmetic op=OR(w1081, w1080, w1079, w1078, w1077) -> (w1082:bool)
          n565 = case shown="True" w1082 {
            frame False {
            }
            frame True {
              w1124 = FALSE
              n566 = local write "MTrig_Solenoid_trig__L"(w1124) -> ()
              n567 = local write "MTrig_Solenoid_trig__R"(w1124) -> ()
              n568 = local write "MTrig_Audio_trig__L"(w1124) -> ()
              n569 = local write "MTrig_Audio_trig__R"(w1124) -> ()
              n570 = local write "MTrig_Laser_trig"(w1124) -> ()
            }
          }
          n571 = case shown="\"initTrial3\"" w1100 {
            selector: w1100 -> [_ _ _ _ _ _ _ _ _ _ _ _ _ _ _ _ _ _ _ _ w1861 _ w1926 _ _ _ _ _ w2068 _ w2143 _ _ _ _ _ w2272 _ w2348 _ w2412 _ w2456 _ _ w2526 _ _ _ _ _ w2698 _ _ _ _ _ _ _ _ _ _ _ _ _ _ _ _ _ _ _]
            tunnel: [myRIO_BRig_RT__Case_Exp_stateList."Start2" ("Enum") myRIO_BRig_RT__Case_Exp_stateList."Start3" ("Enum") myRIO_BRig_RT__Case_Exp_stateList."saveSettings1" ("Enum") myRIO_BRig_RT__Case_Exp_stateList."saveSettings2" ("Enum") myRIO_BRig_RT__Case_Exp_stateList."saveSettings3" ("Enum") myRIO_BRig_RT__Case_Exp_stateList."saveSettings4_LC_ENL" ("Enum") myRIO_BRig_RT__Case_Exp_stateList."saveSettings5_LC_Cue" ("Enum") myRIO_BRig_RT__Case_Exp_stateList."saveSettings6_LC_Other" ("Enum") myRIO_BRig_RT__Case_Exp_stateList."setSettings_Audio" ("Enum") myRIO_BRig_RT__Case_Exp_stateList."setSettings_Laser" ("Enum") myRIO_BRig_RT__Case_Exp_stateList."commConnect" ("Enum") w1622 myRIO_BRig_RT__Case_Exp_stateList."initTrial" ("Enum") w1666 myRIO_BRig_RT__Case_Exp_stateList."initTrial3" ("Enum") myRIO_BRig_RT__Case_Exp_stateList."initTrial_LC_ENL1" ("Enum") myRIO_BRig_RT__Case_Exp_stateList."ENL1_pre" ("Enum") myRIO_BRig_RT__Case_Exp_stateList."initTrial_LC_Cue1" ("Enum") myRIO_BRig_RT__Case_Exp_stateList."initTrial4" ("Enum") w1820 w1858 myRIO_BRig_RT__Case_Exp_stateList."ENL1Penalty" ("Enum") w1927 myRIO_BRig_RT__Case_Exp_stateList."endExp" ("Enum") myRIO_BRig_RT__Case_Exp_stateList."endExp" ("Enum") myRIO_BRig_RT__Case_Exp_stateList."endExp" ("Enum") myRIO_BRig_RT__Case_Exp_stateList."endExp" ("Enum") w2022 w2067 myRIO_BRig_RT__Case_Exp_stateList."Cue1Penalty" ("Enum") w2141 myRIO_BRig_RT__Case_Exp_stateList."endExp" ("Enum") myRIO_BRig_RT__Case_Exp_stateList."endExp" ("Enum") myRIO_BRig_RT__Case_Exp_stateList."endExp" ("Enum") myRIO_BRig_RT__Case_Exp_stateList."endExp" ("Enum") w2229 w2280 myRIO_BRig_RT__Case_Exp_stateList."SelectReward" ("Enum") w2349 myRIO_BRig_RT__Case_Exp_stateList."SelectRewardPost" ("Enum") w2413 myRIO_BRig_RT__Case_Exp_stateList."SelectWrong" ("Enum") w2452 myRIO_BRig_RT__Case_Exp_stateList."endTrial1" ("Enum") myRIO_BRig_RT__Case_Exp_stateList."SelectTimeout" ("Enum") w2528 myRIO_BRig_RT__Case_Exp_stateList."endTrial1" ("Enum") myRIO_BRig_RT__Case_Exp_stateList."endTrial2" ("Enum") myRIO_BRig_RT__Case_Exp_stateList."saveData_dataBlock" ("Enum") w2611 w2681 w2698 myRIO_BRig_RT__Case_Exp_stateList."initBlock" ("Enum") w2725 myRIO_BRig_RT__Case_Exp_stateList."commUpload_dataCurrent" ("Enum") myRIO_BRig_RT__Case_Exp_stateList."commUpload_dataExp" ("Enum") myRIO_BRig_RT__Case_Exp_stateList."commUpload_dataLC" ("Enum") myRIO_BRig_RT__Case_Exp_stateList."commUpload_dataTrial" ("Enum") myRIO_BRig_RT__Case_Exp_stateList."endTrial3" ("Enum") myRIO_BRig_RT__Case_Exp_stateList."saveData_dataCurrent" ("Enum") myRIO_BRig_RT__Case_Exp_stateList."saveData_dataExp" ("Enum") myRIO_BRig_RT__Case_Exp_stateList."saveData_dataLC" ("Enum") myRIO_BRig_RT__Case_Exp_stateList."saveData_dataTrial" ("Enum") myRIO_BRig_RT__Case_Exp_stateList."commUpload_pre" ("Enum") myRIO_BRig_RT__Case_Exp_stateList."empty_endBlock2" ("Enum") myRIO_BRig_RT__Case_Exp_stateList."initBlock" ("Enum") myRIO_BRig_RT__Case_Exp_stateList."empty_endTrial2" ("Enum") myRIO_BRig_RT__Case_Exp_stateList."empty_endTrial3" ("Enum") myRIO_BRig_RT__Case_Exp_stateList."empty_endTrial4" ("Enum") myRIO_BRig_RT__Case_Exp_stateList."empty_endTrial5" ("Enum") myRIO_BRig_RT__Case_Exp_stateList."initTrial" ("Enum")] -> w1069
            tunnel: [w1150 w1169 w1191 w1246 w1294 w1361 w1413 w1465 w1509 w1535 w1594 w1598 w1630 w1647 w1682 w1712 w1745 w1769 w1795 w1836 w1874 w1904 w1931 w1947 w1969 w1988 w2007 w2041 w2089 w2114 w2140 w2161 w2182 w2201 w2220 w2240 w2298 w2323 w2346 w2360 w2410 w2434 w2466 w2487 w2507 w2539 w2562 w2574 w2593 w2635 w2654 w2697 w2714 w2728 w2762 w2783 w2804 w2825 w2846 w2874 w2894 w2921 w2941 w2966 w2985 w3004 w3023 w3042 w3061 w3080 w3099] -> w1121
            tunnel: w1123 -> [w1150 w1169 w1191 w1246 w1294 w1361 w1413 w1465 w1509 w1535 w1594 w1621 w1630 w1647 w1682 w1712 w1745 w1769 w1795 w1836 w1874 w1904 w1931 w1947 w1969 w1988 w2007 w2041 w2089 w2114 w2140 w2161 w2182 w2201 w2220 w2240 w2298 w2323 w2346 w2360 w2410 w2434 w2466 w2487 w2507 w2539 w2562 w2574 w2593 w2635 w2654 w2697 w2714 w2728 w2762 w2783 w2804 w2825 w2846 w2874 w2894 w2921 w2941 w2966 w2985 w3004 w3023 w3042 w3061 w3080 w3099]
            tunnel: w1122 -> [w1153 w1172 w1188 w1249 w1297 w1364 w1416 w1468 w1512 w1538 w1597 w1615 w1641 w1667 w1700 w1728 w1759 w1782 w1808 w1823 w1855 w1907 w1934 w1953 w1972 w1991 w2010 w2021 w2066 w2122 w2147 w2166 w2185 w2204 w2223 w2238 w2296 w2333 w2356 w2391 w2418 w2445 w2469 w2486 w2519 w2544 w2559 w2582 w2592 w2646 w2680 w2701 w2711 w2737 w2765 w2786 w2807 w2828 w2849 w2877 w2897 w2924 w2944 w2969 w2988 w3007 w3026 w3045 w3064 w3083 w3102]
            tunnel: w1116 -> [w1152 w1171 w1189 w1248 w1296 w1363 w1415 w1467 w1511 w1537 w1596 w1614 w1640 w1668 w1699 w1729 w1760 w1783 w1809 w1846 w1876 w1906 w1933 w1952 w1971 w1990 w2009 w2055 w2090 w2121 w2146 w2165 w2184 w2203 w2222 w2239 w2295 w2332 w2355 w2390 w2417 w2444 w2468 w2485 w2518 w2543 w2560 w2583 w2591 w2645 w2679 w2700 w2712 w2738 w2764 w2785 w2806 w2827 w2848 w2876 w2896 w2923 w2943 w2968 w2987 w3006 w3025 w3044 w3063 w3082 w3101]
            tunnel: w1115 -> [w1151 w1170 w1190 w1247 w1295 w1362 w1414 w1466 w1510 w1536 w1595 w1613 w1639 w1669 w1698 w1730 w1761 w1784 w1810 w1845 w1875 w1905 w1932 w1951 w1970 w1989 w2008 w2054 w2091 w2120 w2145 w2164 w2183 w2202 w2221 w2258 w2299 w2331 w2354 w2389 w2416 w2443 w2467 w2484 w2517 w2542 w2561 w2584 w2590 w2644 w2678 w2699 w2713 w2739 w2763 w2784 w2805 w2826 w2847 w2875 w2895 w2922 w2942 w2967 w2986 w3005 w3024 w3043 w3062 w3081 w3100]
            tunnel: [w1153 w1172 w1188 w1249 w1297 w1364 w1416 w1468 w1512 w1538 w1597 w1615 w1641 w1667 w1700 w1728 w1759 w1782 w1808 w1823 w1855 w1907 w1934 w1953 w1972 w1991 w2010 w2021 w2066 w2122 w2147 w2166 w2185 w2204 w2223 w2238 w2296 w2333 w2356 w2391 w2418 w2445 w2469 w2486 w2519 w2544 w2559 w2582 w2592 w2646 w2680 w2701 w2711 w2737 w2765 w2786 w2807 w2828 w2849 w2877 w2897 w2924 w2944 w2969 w2988 w3007 w3026 w3045 w3064 w3083 w3102] -> w1103
            tunnel: [w1152 w1171 w1189 w1248 w1296 w1363 w1415 w1467 w1511 w1537 w1596 w1614 w1640 w1668 w1699 w1729 w1760 w1783 w1809 w1846 w1876 w1906 w1933 w1952 w1971 w1990 w2009 w2055 w2090 w2121 w2146 w2165 w2184 w2203 w2222 w2239 w2295 w2332 w2355 w2390 w2417 w2444 w2468 w2485 w2518 w2543 w2560 w2583 w2591 w2645 w2679 w2700 w2712 w2738 w2764 w2785 w2806 w2827 w2848 w2876 w2896 w2923 w2943 w2968 w2987 w3006 w3025 w3044 w3063 w3082 w3101] -> w1102
            tunnel: [w1151 w1170 w1190 w1247 w1295 w1362 w1414 w1466 w1510 w1536 w1595 w1613 w1639 w1669 w1698 w1730 w1761 w1784 w1810 w1845 w1875 w1905 w1932 w1951 w1970 w1989 w2008 w2054 w2091 w2120 w2145 w2164 w2183 w2202 w2221 w2258 w2299 w2331 w2354 w2389 w2416 w2443 w2467 w2484 w2517 w2542 w2561 w2584 w2590 w2644 w2678 w2699 w2713 w2739 w2763 w2784 w2805 w2826 w2847 w2875 w2895 w2922 w2942 w2967 w2986 w3005 w3024 w3043 w3062 w3081 w3100] -> w1101
            tunnel: w1061 -> [w1149 w1168 w1187 w1213 w1270 w1338 w1412 w1464 w1508 w1533 w1554 w1620 w1629 w1665 w1671 w1713 w1740 w1766 w1794 w1835 w1860 w1898 w1930 w1948 w1968 w1987 w2006 w2025 w2086 w2113 w2144 w2162 w2181 w2200 w2219 w2249 w2276 w2315 w2351 w2362 w2415 w2435 w2465 w2483 w2508 w2541 w2558 w2571 w2595 w2615 w2652 w2696 w2715 w2740 w2759 w2780 w2801 w2822 w2833 w2863 w2882 w2906 w2938 w2955 w2975 w2994 w3013 w3032 w3051 w3070 w3089]
            tunnel: w1056 -> [w1148 w1167 w1186 w1244 w1292 w1358 w1410 w1462 w1506 w1526 w1590 w1619 w1638 w1664 w1679 w1711 w1747 w1772 w1798 w1838 w1873 w1897 w1928 w1950 w1967 w1986 w2005 w2043 w2088 w2111 w2139 w2163 w2180 w2199 w2218 w2251 w2297 w2329 w2353 w2383 w2411 w2436 w2463 w2482 w2510 w2538 w2557 w2581 w2598 w2614 w2671 w2695 w2716 w2741 w2758 w2779 w2800 w2821 w2834 w2871 w2891 w2902 w2937 w2963 w2982 w3001 w3020 w3039 w3058 w3077 w3096]
            tunnel: [w1149 w1168 w1187 w1213 w1270 w1337 w1412 w1464 w1508 w1533 w1576 w1604 w1629 w1653 w1671 w1713 w1740 w1765 w1793 w1839 w1859 w1899 w1929 w1948 w1968 w1987 w2006 w2050 w2085 w2112 w2142 w2162 w2181 w2200 w2219 w2252 w2271 w2330 w2350 w2384 w2414 w2437 w2464 w2483 w2511 w2540 w2558 w2570 w2594 w2615 w2650 w2696 w2715 w2740 w2759 w2780 w2801 w2822 w2833 w2863 w2882 w2906 w2938 w2955 w2975 w2994 w3013 w3032 w3051 w3070 w3089] -> w1097
            tunnel: [w1148 w1167 w1186 w1243 w1291 w1353 w1410 w1462 w1506 w1526 w1590 w1618 w1638 w1663 w1679 w1711 w1747 w1772 w1798 w1838 w1873 w1897 w1928 w1950 w1967 w1986 w2005 w2043 w2088 w2111 w2139 w2163 w2180 w2199 w2218 w2251 w2297 w2329 w2353 w2383 w2411 w2436 w2463 w2482 w2510 w2538 w2557 w2581 w2598 w2614 w2671 w2695 w2716 w2741 w2758 w2779 w2800 w2821 w2834 w2871 w2891 w2905 w2937 w2963 w2982 w3001 w3020 w3039 w3058 w3077 w3096] -> w1112
            tunnel: [_ _ _ _ _ _ _ _ _ _ _ _ _ _ _ _ _ _ _ _ _ _ _ _ _ _ _ _ _ _ _ _ _ _ _ _ _ _ w2344 _ _ _ _ _ _ _ _ _ _ _ _ _ _ _ _ _ _ _ _ _ _ _ _ _ _ _ _ _ _ _ _] -> w1072
            tunnel: [_ _ _ _ _ _ _ _ _ _ _ _ _ _ _ _ _ _ _ _ _ _ _ _ _ _ _ _ _ _ _ _ _ _ _ _ _ _ w2345 _ _ _ _ _ _ _ _ _ _ _ _ _ _ _ _ _ _ _ _ _ _ _ _ _ _ _ _ _ _ _ _] -> w1074
            tunnel: w1111 -> [w1146 w1165 w1184 w1215 w1272 w1359 w1411 w1463 w1507 w1531 w1591 w1616 w1631 w1661 w1691 w1726 w1757 w1762 w1790 w1837 w1872 w1894 w1924 w1949 w1965 w1984 w2003 w2049 w2087 w2110 w2137 w2159 w2178 w2197 w2216 w2250 w2293 w2321 w2352 w2364 w2408 w2433 w2461 w2480 w2509 w2537 w2555 w2573 w2600 w2642 w2663 w2693 w2718 w2743 w2756 w2777 w2798 w2819 w2843 w2857 w2884 w2912 w2931 w2957 w2976 w2995 w3014 w3033 w3052 w3071 w3090]
            tunnel: [w1146 w1165 w1184 w1215 w1272 w1359 w1411 w1463 w1507 w1531 w1591 w1616 w1628 w1661 w1691 w1726 w1757 w1762 w1790 w1837 w1872 w1894 w1924 w1949 w1965 w1984 w2003 w2049 w2087 w2110 w2137 w2159 w2178 w2197 w2216 w2250 w2293 w2321 w2352 w2363 w2408 w2433 w2461 w2480 w2509 w2537 w2555 w2572 w2600 w2642 w2663 w2693 w2718 w2743 w2756 w2777 w2798 w2819 w2843 w2857 w2884 w2912 w2931 w2957 w2976 w2995 w3014 w3033 w3052 w3071 w3090] -> w1110
            tunnel: w1109 -> [w1147 w1166 w1185 w1214 w1271 w1360 w1408 w1460 w1504 w1532 w1592 w1617 w1637 w1662 w1670 w1727 w1758 w1770 w1796 w1834 w1854 w1895 w1925 w1946 w1966 w1985 w2004 w2048 w2065 w2109 w2138 w2160 w2179 w2198 w2217 w2248 w2294 w2322 w2347 w2381 w2409 w2432 w2462 w2481 w2506 w2535 w2556 w2580 w2599 w2643 w2670 w2694 w2717 w2742 w2757 w2778 w2799 w2820 w2844 w2870 w2890 w2918 w2929 w2962 w2981 w3000 w3019 w3038 w3057 w3076 w3095]
            tunnel: [w1147 w1166 w1185 w1214 w1271 w1360 w1409 w1461 w1505 w1532 w1592 w1617 w1637 w1662 w1670 w1727 w1758 w1770 w1796 w1834 w1854 w1895 w1925 w1946 w1966 w1985 w2004 w2048 w2065 w2109 w2138 w2160 w2179 w2198 w2217 w2248 w2294 w2322 w2347 w2381 w2409 w2432 w2462 w2481 w2506 w2535 w2556 w2580 w2599 w2643 w2670 w2694 w2717 w2742 w2757 w2778 w2799 w2820 w2844 w2870 w2890 w2918 w2929 w2962 w2981 w3000 w3019 w3038 w3057 w3076 w3095] -> w1108
            tunnel: w1107 -> [_ _ _ _ _ _ _ _ _ _ _ _ _ _ _ _ _ _ _ w1819 w1847 w1880 w1913 _ _ _ _ _ w2059 w2096 _ _ _ _ _ _ _ _ _ _ _ _ _ _ _ w2536 _ _ _ _ _ _ _ _ _ _ _ _ _ _ _ _ _ _ _ _ _ _ _ _ _]
            tunnel: [_ _ _ _ _ _ _ _ _ _ _ _ _ _ _ _ _ _ _ _ _ _ _ _ _ _ _ _ _ _ _ _ _ _ _ _ _ _ _ _ _ _ _ _ _ _ _ _ _ _ _ TRUE _ _ _ _ _ _ _ _ _ _ _ _ _ _ _ _ _ _ _] -> w1104
            tunnel: w1093 -> [w1144 w1163 w1182 w1205 w1265 w1348 w1395 w1447 w1476 _ w1582 w1612 w1636 w1660 w1690 w1725 w1756 w1781 w1807 w1833 w1871 w1892 w1923 w1944 w1963 w1982 w2001 w2047 w2082 w2107 w2136 w2157 w2176 w2195 w2214 w2247 w2292 w2311 w2343 w2379 w2407 w2430 w2460 w2479 w2504 w2534 w2554 w2578 w2604 w2641 w2667 w2691 w2709 w2736 w2754 w2775 w2796 w2817 w2841 w2868 w2888 w2916 w2935 w2961 w2980 w2999 w3018 w3037 w3056 w3075 w3094]
            tunnel: w1092 -> [w1143 w1162 w1181 w1204 w1264 w1347 w1394 w1446 w1477 _ w1581 w1611 w1635 w1659 w1689 w1724 w1755 w1780 w1806 w1832 w1870 w1891 w1922 w1943 w1962 w1981 w2000 w2046 w2081 w2106 w2135 w2156 w2175 w2194 w2213 w2246 w2291 w2310 w2342 w2378 w2406 w2429 w2459 w2478 w2503 w2533 w2553 w2577 w2603 w2640 w2666 w2690 w2708 w2735 w2753 w2774 w2795 w2816 w2840 w2867 w2887 w2915 w2934 w2960 w2979 w2998 w3017 w3036 w3055 w3074 w3093]
            tunnel: w1091 -> [w1142 w1161 w1180 w1203 w1263 w1346 w1393 w1445 w1478 _ w1580 w1610 w1634 w1658 w1688 w1723 w1754 w1779 w1805 w1831 w1869 w1890 w1921 w1942 w1961 w1980 w1999 w2045 w2080 w2105 w2134 w2155 w2174 w2193 w2212 w2245 w2290 w2309 w2341 w2377 w2405 w2428 w2458 w2477 w2502 w2532 w2552 w2576 w2602 w2639 w2665 w2689 w2707 w2734 w2752 w2773 w2794 w2815 w2839 w2866 w2886 w2914 w2933 w2959 w2978 w2997 w3016 w3035 w3054 w3073 w3092]
            tunnel: w1090 -> [w1141 w1160 w1179 w1202 w1262 w1345 w1392 w1444 w1479 _ w1579 w1609 w1633 w1657 w1687 w1722 w1753 w1778 w1804 w1830 w1868 w1889 w1920 w1941 w1960 w1979 w1998 w2044 w2079 w2104 w2133 w2154 w2173 w2192 w2211 w2244 w2289 w2308 w2340 w2376 w2404 w2427 w2457 w2476 w2501 w2531 w2551 w2575 w2601 w2638 w2664 w2688 w2706 w2733 w2751 w2772 w2793 w2814 w2838 w2865 w2885 w2913 w2932 w2958 w2977 w2996 w3015 w3034 w3053 w3072 w3091]
            tunnel: w1089 -> [_ _ _ _ _ _ _ _ _ _ _ _ _ _ _ _ _ _ _ _ _ _ _ _ _ _ _ _ w2084 _ _ _ _ _ _ _ _ _ _ _ _ _ _ _ _ _ _ _ _ _ _ _ _ _ _ _ _ _ _ _ _ _ _ _ _ _ _ _ _ _ _]
            tunnel: w1088 -> [_ _ _ _ _ _ _ _ _ _ _ _ _ _ _ _ _ _ _ _ _ _ _ _ _ _ _ _ w2083 _ _ _ _ _ _ _ _ _ _ _ _ _ _ _ _ _ _ _ _ _ _ _ _ _ _ _ _ _ _ _ _ _ _ _ _ _ _ _ _ _ _]
            tunnel: [w1144 w1163 w1182 w1205 w1265 w1348 w1395 w1447 w1476 w1525 w1582 w1612 w1636 w1660 w1690 w1725 w1756 w1781 w1807 w1833 w1871 w1892 w1923 w1944 w1963 w1982 w2001 w2047 w2082 w2107 w2136 w2157 w2176 w2195 w2214 w2247 w2292 w2311 w2343 w2379 w2407 w2430 w2460 w2479 w2504 w2534 w2554 w2578 w2604 w2641 w2667 w2691 w2709 w2736 w2754 w2775 w2796 w2817 w2841 w2868 w2888 w2916 w2935 w2961 w2980 w2999 w3018 w3037 w3056 w3075 w3094] -> w1085
            tunnel: [w1143 w1162 w1181 w1204 w1264 w1347 w1394 w1446 w1477 w1516 w1581 w1611 w1635 w1659 w1689 w1724 w1755 w1780 w1806 w1832 w1870 w1891 w1922 w1943 w1962 w1981 w2000 w2046 w2081 w2106 w2135 w2156 w2175 w2194 w2213 w2246 w2291 w2310 w2342 w2378 w2406 w2429 w2459 w2478 w2503 w2533 w2553 w2577 w2603 w2640 w2666 w2690 w2708 w2735 w2753 w2774 w2795 w2816 w2840 w2867 w2887 w2915 w2934 w2960 w2979 w2998 w3017 w3036 w3055 w3074 w3093] -> w1053
            tunnel: [w1142 w1161 w1180 w1203 w1263 w1346 w1393 w1445 w1478 w1524 w1580 w1610 w1634 w1658 w1688 w1723 w1754 w1779 w1805 w1831 w1869 w1890 w1921 w1942 w1961 w1980 w1999 w2045 w2080 w2105 w2134 w2155 w2174 w2193 w2212 w2245 w2290 w2309 w2341 w2377 w2405 w2428 w2458 w2477 w2502 w2532 w2552 w2576 w2602 w2639 w2665 w2689 w2707 w2734 w2752 w2773 w2794 w2815 w2839 w2866 w2886 w2914 w2933 w2959 w2978 w2997 w3016 w3035 w3054 w3073 w3092] -> w1086
            tunnel: [w1141 w1160 w1179 w1202 w1262 w1345 w1392 w1444 w1479 w1514 w1579 w1609 w1633 w1657 w1687 w1722 w1753 w1778 w1804 w1830 w1868 w1889 w1920 w1941 w1960 w1979 w1998 w2044 w2079 w2104 w2133 w2154 w2173 w2192 w2211 w2244 w2289 w2308 w2340 w2376 w2404 w2427 w2457 w2476 w2501 w2531 w2551 w2575 w2601 w2638 w2664 w2688 w2706 w2733 w2751 w2772 w2793 w2814 w2838 w2865 w2885 w2913 w2932 w2958 w2977 w2996 w3015 w3034 w3053 w3072 w3091] -> w1087
            tunnel: [_ _ _ _ _ _ _ _ _ _ _ _ _ _ _ _ _ _ _ _ _ _ _ _ _ _ _ w2034 w2084 _ _ _ _ _ _ _ _ _ _ _ _ _ _ _ _ _ _ _ _ _ _ _ _ _ _ _ _ _ _ _ _ _ _ _ _ _ _ _ _ _ _] -> w1055
            tunnel: [_ _ _ _ _ _ _ _ _ _ _ _ _ _ _ _ _ _ _ _ _ _ _ _ _ _ _ w2033 w2083 _ _ _ _ _ _ _ _ _ _ _ _ _ _ _ _ _ _ _ _ _ _ _ _ _ _ _ _ _ _ _ _ _ _ _ _ _ _ _ _ _ _] -> w1054
            tunnel: w1068 -> [w1140 w1159 w1178 w1201 w1261 w1344 w1391 w1443 w1475 w1523 w1589 w1608 w1632 w1656 w1673 w1715 w1739 w1764 w1792 w1829 w1867 w1888 w1919 w1940 w1959 w1978 w1997 w2032 w2078 w2103 w2132 w2153 w2172 w2191 w2210 w2243 w2288 w2305 w2339 w2375 w2403 w2424 w2451 w2475 w2498 w2525 w2550 w2569 w2597 w2631 w2662 w2687 w2719 w2744 w2755 w2776 w2797 w2818 w2842 w2869 w2889 w2917 w2936 w2952 w2974 w2993 w3012 w3031 w3050 w3069 w3088]
            tunnel: [w1140 w1159 w1178 w1201 w1261 w1344 w1391 w1443 w1475 w1523 w1589 w1608 w1632 w1656 w1672 w1714 w1732 w1763 w1791 w1829 w1867 w1888 w1919 w1940 w1959 w1978 w1997 w2032 w2078 w2103 w2132 w2153 w2172 w2191 w2210 w2243 w2288 w2305 w2339 w2375 w2403 w2424 w2451 w2475 w2498 w2525 w2550 w2569 w2596 w2631 w2662 w2687 w2719 w2744 w2755 w2776 w2797 w2818 w2842 w2869 w2889 w2917 w2936 w2952 w2974 w2993 w3012 w3031 w3050 w3069 w3088] -> w1067
            tunnel: [w1139 w1158 w1177 w1200 w1260 w1343 w1390 w1442 w1474 w1522 w1588 w1607 w1643 w1655 w1693 w1721 w1752 w1777 w1803 w1828 w1866 w1887 w1918 w1939 w1958 w1977 w1996 w2031 w2077 w2102 w2131 w2152 w2171 w2190 w2209 w2242 w2287 w2304 w2338 w2374 w2402 w2423 w2450 w2474 w2497 w2524 w2549 w2568 w2589 w2637 w2661 w2685 w2720 w2730 w2750 w2771 w2792 w2813 w2837 w2873 w2893 w2920 w2940 w2965 w2984 w3003 w3022 w3041 w3060 w3079 w3098] -> w1066
            tunnel: [w1138 w1157 w1176 w1199 w1259 w1342 w1389 w1441 w1473 w1521 w1587 w1606 w1642 w1654 w1692 w1720 w1751 w1776 w1802 w1827 w1865 w1886 w1917 w1938 w1957 w1976 w1995 w2030 w2076 w2101 w2130 w2151 w2170 w2189 w2208 w2241 w2286 w2303 w2337 w2373 w2401 w2422 w2449 w2473 w2496 w2523 w2548 w2567 w2588 w2636 w2660 w2686 w2702 w2727 w2760 w2781 w2802 w2823 w2845 w2872 w2892 w2919 w2939 w2964 w2983 w3002 w3021 w3040 w3059 w3078 w3097] -> w1065
            tunnel: w1064 -> [w1139 w1158 w1177 w1200 w1260 w1343 w1390 w1442 w1474 w1522 w1588 w1607 w1643 w1655 w1693 w1721 w1752 w1777 w1803 w1828 w1866 w1887 w1918 w1939 w1958 w1977 w1996 w2031 w2077 w2102 w2131 w2152 w2171 w2190 w2209 w2242 w2287 w2304 w2338 w2374 w2402 w2423 w2450 w2474 w2497 w2524 w2549 w2568 w2589 w2637 w2661 w2685 _ w2730 w2750 w2771 w2792 w2813 w2837 w2873 w2893 w2920 w2940 w2965 w2984 w3003 w3022 w3041 w3060 w3079 w3098]
            tunnel: w1063 -> [w1138 w1157 w1176 w1199 w1259 w1342 w1389 w1441 w1473 w1521 w1587 w1606 w1642 w1654 w1692 w1720 w1751 w1776 w1802 w1827 w1865 w1886 w1917 w1938 w1957 w1976 w1995 w2030 w2076 w2101 w2130 w2151 w2170 w2189 w2208 w2241 w2286 w2303 w2337 w2373 w2401 w2422 w2449 w2473 w2496 w2523 w2548 w2567 w2588 w2636 w2660 w2686 _ w2727 w2760 w2781 w2802 w2823 w2845 w2872 w2892 w2919 w2939 w2964 w2983 w3002 w3021 w3040 w3059 w3078 w3097]
            tunnel: w1062 -> [_ _ _ _ _ _ _ _ _ _ _ _ _ _ _ _ _ _ _ _ _ _ _ _ _ _ _ _ _ _ _ _ _ _ _ _ _ _ _ _ _ _ _ _ _ _ _ _ _ _ _ _ _ _ w2748 w2769 w2790 w2811 w2835 _ _ _ _ _ _ _ _ _ _ _ _]
            tunnel: w1060 -> [_ _ _ _ _ _ _ _ _ _ _ _ _ _ _ _ w1744 _ w1787 w1816 w1852 w1878 w1909 _ _ _ _ w2012 w2057 w2095 w2124 _ _ _ _ _ _ _ _ _ _ _ _ _ _ _ _ _ _ _ _ _ _ _ _ _ _ _ _ _ _ _ _ _ _ _ _ _ _ _ _]
            tunnel: w1057 -> [_ _ _ _ _ _ _ _ _ _ _ _ _ _ _ _ _ _ _ _ _ _ _ _ _ _ _ _ _ _ _ _ _ _ _ _ _ _ _ _ _ _ _ _ _ _ _ _ _ _ _ _ _ _ _ _ _ _ _ _ _ w2907 _ _ _ _ _ _ _ _ _]
            tunnel: [w1137 w1156 w1175 w1198 w1258 w1341 w1388 w1440 w1472 w1520 w1586 w1601 w1626 w1650 w1694 w1719 w1750 w1775 w1801 w1826 w1864 w1885 w1916 w1937 w1956 w1975 w1994 w2029 w2075 w2100 w2129 w2150 w2169 w2188 w2207 w2237 w2285 w2302 w2336 w2358 w2400 w2421 w2448 w2472 w2495 w2522 w2547 w2566 w2587 w2634 w2647 w2684 w2705 w2729 w2747 w2768 w2789 w2810 w2832 w2852 w2881 w2901 w2928 w2948 w2973 w2992 w3011 w3030 w3049 w3068 w3087] -> w1051
            tunnel: w1052 -> [w1137 w1156 w1175 w1198 w1258 w1341 w1388 w1440 w1472 w1520 w1586 w1601 _ w1650 w1694 w1719 w1750 w1775 w1801 w1826 w1864 w1885 w1916 w1937 w1956 w1975 w1994 w2029 w2075 w2100 w2129 w2150 w2169 w2188 w2207 w2237 w2285 w2302 w2336 w2358 w2400 w2421 w2448 w2472 w2495 w2522 w2547 w2566 w2587 w2634 w2648 w2684 w2705 w2729 w2747 w2768 w2789 w2810 w2832 w2852 w2881 w2901 w2928 w2948 w2973 w2992 w3011 w3030 w3049 w3068 w3087]
            tunnel: w1050 -> [w1136 w1155 w1174 w1197 w1257 w1340 w1387 w1439 w1471 w1519 w1585 w1600 w1625 w1649 w1686 w1718 w1749 w1774 w1800 w1825 w1863 w1884 w1915 w1936 w1955 w1974 w1993 w2028 w2074 w2099 w2128 w2149 w2168 w2187 w2206 w2236 w2284 w2301 w2335 w2372 w2399 w2420 w2447 w2471 w2494 w2521 w2546 w2565 w2586 w2633 w2659 w2683 w2704 w2732 w2746 w2767 w2788 w2809 w2831 w2851 w2880 w2900 w2927 w2947 w2972 w2991 w3010 w3029 w3048 w3067 w3086]
            tunnel: w1049 -> [w1135 w1154 w1173 w1196 w1256 w1339 w1386 w1438 w1470 w1518 w1584 w1599 w1624 w1648 w1685 w1717 w1748 w1773 w1799 w1824 w1862 w1883 w1914 w1935 w1954 w1973 w1992 w2027 w2073 w2098 w2127 w2148 w2167 w2186 w2205 w2235 w2283 w2300 w2334 w2369 w2398 w2419 w2446 w2470 w2493 w2520 w2545 w2564 w2585 w2632 w2658 w2682 w2703 w2731 w2745 w2766 w2787 w2808 w2830 w2850 w2879 w2899 w2926 w2946 w2971 w2990 w3009 w3028 w3047 w3066 w3085]
            tunnel: [w1136 w1155 w1174 w1197 w1257 w1340 w1387 w1439 w1471 w1519 w1585 w1600 w1625 w1649 w1686 w1718 w1749 w1774 w1800 w1825 w1863 w1884 w1915 w1936 w1955 w1974 w1993 w2028 w2074 w2099 w2128 w2149 w2168 w2187 w2206 w2236 w2284 w2301 w2335 w2371 w2399 w2420 w2447 w2471 w2494 w2521 w2546 w2565 w2586 w2633 w2659 w2683 w2704 w2732 w2746 w2767 w2788 w2809 w2831 w2851 w2880 w2900 w2927 w2947 w2972 w2991 w3010 w3029 w3048 w3067 w3086] -> w1048
            tunnel: [w1135 w1154 w1173 w1196 w1256 w1339 w1386 w1438 w1470 w1518 w1584 w1599 w1624 w1648 w1685 w1717 w1748 w1773 w1799 w1824 w1862 w1883 w1914 w1935 w1954 w1973 w1992 w2027 w2073 w2098 w2127 w2148 w2167 w2186 w2205 w2235 w2283 w2300 w2334 w2370 w2398 w2419 w2446 w2470 w2493 w2520 w2545 w2564 w2585 w2632 w2658 w2682 w2703 w2731 w2745 w2766 w2787 w2808 w2830 w2850 w2879 w2899 w2926 w2946 w2971 w2990 w3009 w3028 w3047 w3066 w3085] -> w1047
            tunnel: w1046 -> [_ _ _ _ _ _ _ _ _ _ w1577 _ _ _ w1697 w1707 _ _ _ _ _ _ _ _ _ _ _ _ w2070 _ _ _ _ _ _ w2233 w2282 _ _ _ _ _ _ _ w2492 _ _ _ _ w2609 _ _ _ _ _ _ _ _ _ _ _ _ _ _ _ _ _ _ _ _ _]
            tunnel: w1045 -> [_ _ _ _ _ _ _ _ _ _ w1578 _ _ _ w1696 w1706 _ _ _ _ _ _ _ _ _ _ _ _ w2069 _ _ _ _ _ _ w2234 w2281 _ _ _ _ _ _ _ w2491 _ _ _ _ w2608 _ _ _ _ _ _ _ _ _ _ _ _ _ _ _ _ _ _ _ _ _]
            tunnel: w1043 -> [_ _ _ _ _ _ _ _ _ _ _ _ _ _ _ _ w1743 _ w1786 w1815 w1851 w1877 w1910 _ _ _ _ w2011 w2056 w2094 w2123 _ _ _ _ _ _ _ _ _ _ _ _ _ _ _ _ _ _ _ _ _ _ _ _ _ _ _ _ _ _ _ _ _ _ _ _ _ _ _ _]
            tunnel: [_ _ _ _ _ _ _ _ _ _ _ _ _ _ _ _ _ _ _ w1819 w1853 w1880 w1913 _ _ _ _ TRUE w2059 w2096 _ _ _ _ _ _ _ _ _ _ _ _ _ _ _ _ _ _ _ _ _ _ _ _ _ _ _ _ _ _ _ _ _ _ _ _ _ _ _ _ _] -> w1042
            tunnel: w1041 -> [_ _ _ _ _ _ _ _ _ _ _ _ _ _ _ _ w1742 _ _ w1818 w1857 w1882 w1911 _ _ _ _ w2019 w2064 w2093 w2126 _ _ _ _ _ _ _ _ _ _ _ _ _ _ _ _ _ _ _ _ _ _ _ _ _ _ _ _ _ _ _ _ _ _ _ _ _ _ _ _]
            tunnel: w1040 -> [_ _ _ _ _ _ _ _ _ _ _ _ _ _ _ _ w1741 _ _ w1817 w1856 w1881 w1912 _ _ _ _ w2018 w2063 w2092 w2125 _ _ _ _ _ _ _ _ _ _ _ _ _ _ _ _ _ _ _ _ _ _ _ _ _ _ _ _ _ _ _ _ _ _ _ _ _ _ _ _]
            tunnel: [_ _ _ _ _ _ _ _ _ _ _ _ _ _ _ _ w1742 _ w1789 w1818 w1857 w1882 w1911 _ _ _ _ w2019 w2064 w2093 w2126 _ _ _ _ _ _ _ _ _ _ _ _ _ _ _ _ _ _ _ _ _ _ _ _ _ _ _ _ _ _ _ _ _ _ _ _ _ _ _ _] -> w1039
            tunnel: [_ _ _ _ _ _ _ _ _ _ _ _ _ _ _ _ w1741 _ w1788 w1817 w1856 w1881 w1912 _ _ _ _ w2018 w2063 w2092 w2125 _ _ _ _ _ _ _ _ _ _ _ _ _ _ _ _ _ _ _ _ _ _ _ _ _ _ _ _ _ _ _ _ _ _ _ _ _ _ _ _] -> w1038
            tunnel: [_ _ _ _ _ _ _ _ _ _ _ _ _ _ _ _ w1744 w1767 w1787 w1816 w1852 w1878 w1909 _ _ _ _ w2012 w2057 w2095 w2124 _ _ _ _ _ _ _ _ _ _ _ _ _ _ _ _ _ _ _ _ _ _ _ _ _ _ _ _ _ _ _ _ _ _ _ _ _ _ _ _] -> w1037
            tunnel: [_ _ _ _ _ _ _ _ _ _ _ _ _ _ _ _ w1743 w1768 w1786 w1815 w1851 w1877 w1910 _ _ _ _ w2011 w2056 w2094 w2123 _ _ _ _ _ _ _ _ _ _ _ _ _ _ _ _ _ _ _ _ _ _ _ _ _ _ _ _ _ _ _ _ _ _ _ _ _ _ _ _] -> w1036
            tunnel: [_ _ _ _ _ _ _ _ _ _ _ _ _ _ _ _ _ _ _ _ w1850 _ _ _ _ _ _ _ w2061 _ _ _ _ _ _ _ _ _ _ _ _ _ _ _ _ _ _ _ _ _ _ _ _ _ _ _ _ _ _ _ _ _ _ _ _ _ _ _ _ _ _] -> w1033
            tunnel: [_ _ _ _ _ _ _ _ _ _ _ _ _ _ _ _ _ _ _ _ w1849 _ _ _ _ _ _ _ w2062 _ _ _ _ _ _ _ _ _ _ _ _ _ _ _ _ _ _ _ _ _ _ _ _ _ _ _ _ _ _ _ _ _ _ _ _ _ _ _ _ _ _] -> w1035
            tunnel: w1030 -> [_ _ _ _ _ _ _ _ _ _ _ _ _ _ _ _ _ _ _ w1814 w1848 w1879 w1908 _ _ _ _ w2014 w2058 w2097 _ _ _ _ _ _ _ _ _ _ _ _ _ _ _ _ _ _ _ _ _ _ _ _ _ _ _ _ _ _ _ _ _ _ _ _ _ _ _ _ _]
            tunnel: [_ _ _ _ _ _ _ _ _ _ _ _ _ _ _ _ _ _ _ w1814 w1848 w1879 w1908 _ _ _ _ w2014 w2060 w2097 _ _ _ _ _ _ _ _ _ _ _ _ _ _ _ _ _ _ _ _ _ _ _ _ _ _ _ _ _ _ _ _ _ _ _ _ _ _ _ _ _] -> w1029
            frame "Start1", Default {
            }
            frame "Start2" {
            }
            frame "Start3" {
            }
            frame "saveSettings1" {
              n572 = call "myRIO_BRig_RT_dataExp_Audio_freq__L.vi"() -> ("output_Audio_freq__L"=w1221:i32)  [unwired: 11 in]
              n573 = call "myRIO_BRig_RT_dataExp_Audio_freq__R.vi"() -> ("output_Audio_freq__R"=w1220:i32)  [unwired: 11 in]
              n574 = call "myRIO_BRig_RT_dataExp_Audio_amp__L.vi"() -> ("output_Audio_amp__L"=w1219:i32)  [unwired: 11 in]
              n575 = call "myRIO_BRig_RT_dataExp_Audio_amp__R.vi"() -> ("output_Audio_amp__R"=w1217:i32)  [unwired: 11 in]
              n576 = call "myRIO_BRig_RT_dataExp_TPB_min__L.vi"() -> ("output_TPB_min__L"=w1229:i32)  [unwired: 11 in]
              n577 = call "myRIO_BRig_RT_dataExp_TPB_min__R.vi"() -> ("output_TPB_min__R"=w1227:i32)  [unwired: 11 in]
              n578 = call "myRIO_BRig_RT_dataExp_TPB_max__L.vi"() -> ("output_TPB_max__L"=w1225:i32)  [unwired: 11 in]
              n579 = call "myRIO_BRig_RT_dataExp_TPB_max__R.vi"() -> ("output_TPB_max__R"=w1223:i32)  [unwired: 11 in]
              n580 = call "myRIO_BRig_RT_dataExp_ItrialUntilReward.vi"() -> ("output_I_trialUntilReward"=w1242:i32)  [unwired: 11 in]
              n581 = call "myRIO_BRig_RT_dataExp_IblockUntilReward.vi"() -> ("output_I_blockUntilReward"=w1238:i32)  [unwired: 11 in]
              n582 = call "myRIO_BRig_RT_dataExp_CueCycles.vi"() -> ("output_CueCycles"=w1237:i32)  [unwired: 11 in]
              n583 = call "myRIO_BRig_RT_dataExp_ENL_min.vi"() -> ("output_ENL_min"=w1235:i32)  [unwired: 11 in]
              n584 = call "myRIO_BRig_RT_dataExp_ENL_max.vi"() -> ("output_ENL_max"=w1233:i32)  [unwired: 11 in]
              n585 = call "myRIO_BRig_RT_dataExp_ENL_penalty.vi"() -> ("output_ENL_penalty"=w1231:i32)  [unwired: 11 in]
              n586 = local read "Audio_Freq__L"() -> (w1195:u8)
              n587 = local read "Audio_Freq__R"() -> (w1193:u8)
              n588 = local read "Audio_Amp__L"() -> (w1218:u16)
              n589 = local read "TpB_Min_L"() -> (w1228:u16)
              n590 = local read "TpB_Min_R"() -> (w1226:u16)
              n591 = local read "TpB_Max_L"() -> (w1224:u16)
              n592 = local read "TpB_Max_R"() -> (w1222:u16)
              n593 = local read "Audio_Amp__R"() -> (w1216:u16)
              n594 = local read "TrialUntilReward"() -> (w1241:bool)
              n595 = local read "CueCycles"() -> (w1236:u16)
              n596 = local read "Tcycle_ENL_min"() -> (w1234:u16)
              n597 = local read "Tcycle_ENL_max"() -> (w1232:u16)
              n598 = local read "Tcycle_ENLPenalty"() -> (w1230:u16)
              n599 = To Unsigned Word Integer(number=w1193) -> (unsigned 16bit integer=w1192:u16)
              n600 = To Unsigned Word Integer(number=w1195) -> (unsigned 16bit integer=w1194:u16)
              n601 = Boolean To (0,1)(Boolean=w1241) -> (0, 1=w1240:i16)
              n602 = To Unsigned Word Integer(number=w1240) -> (unsigned 16bit integer=w1239:u16)
              n603 = local read "BUR_min"() -> (w1210:u16)
              n604 = local read "BUR_max"() -> (w1211:u16)
              n605 = Not Equal To 0?(x=w1210) -> (x != 0?=w1209:bool)
              n606 = Not Equal To 0?(x=w1211) -> (x != 0?=w1208:bool)
              n607 = And(x=w1209, y=w1208) -> (x .and. y?=w1207:bool)
              n608 = Boolean To (0,1)(Boolean=w1207) -> (0, 1=w1212:i16)
              n609 = To Unsigned Word Integer(number=w1212) -> (unsigned 16bit integer=w1206:u16)
              n610 = Replace Array Subset(array=w1244, new element #1=w1239, index #1=w1242, new element #2=w1206, index #2=w1238, new element #3=w1236, index #3=w1237, new element #4=w1234, index #4=w1235, new element #5=w1232, index #5=w1233, new element #6=w1230, index #6=w1231, new element #7=w1228, index #7=w1229, new element #8=w1226, index #8=w1227, new element #9=w1224, index #9=w1225, new element #10=w1222, index #10=w1223, new element #11=w1194, index #11=w1221, new element #12=w1192, index #12=w1220, new element #13=w1218, index #13=w1219, new element #14=w1216, index #14=w1217) -> (w1243:u16[])
            }
            frame "saveSettings2" {
              n611 = call "myRIO_BRig_RT_dataExp_Tcycle_RewardPost.vi"() -> ("output_Tcycle_RewardPost"=w1281:i32)  [unwired: 11 in]
              n612 = call "myRIO_BRig_RT_dataExp_Tcycle_Wrong.vi"() -> ("output_Tcycle_Wrong"=w1279:i32)  [unwired: 11 in]
              n613 = call "myRIO_BRig_RT_dataExp_Tcycle_Timeout.vi"() -> ("output_Tcycle_Timeout"=w1277:i32)  [unwired: 11 in]
              n614 = call "myRIO_BRig_RT_dataExp_Tcycle_Cue_min.vi"() -> ("output_Tcycle_Cue_min"=w1275:i32)  [unwired: 11 in]
              n615 = call "myRIO_BRig_RT_dataExp_Tcycle_Cue_max.vi"() -> ("output_Tcycle_Cue_max"=w1274:i32)  [unwired: 11 in]
              n616 = call "myRIO_BRig_RT_dataExp_Tcycle_CuePenalty.vi"() -> ("output_Tcycle_CuePenalty"=w1273:i32)  [unwired: 11 in]
              n617 = call "myRIO_BRig_RT_dataExp_SolenoidProbability_L.vi"() -> ("output_SolenoidProbability_L"=w1253:i32)  [unwired: 11 in]
              n618 = call "myRIO_BRig_RT_dataExp_SolenoidProbability_R.vi"() -> ("output_SolenoidProbability_R"=w1252:i32)  [unwired: 11 in]
              n619 = call "myRIO_BRig_RT_dataExp_nBlock.vi"() -> ("output_nBlock"=w1290:i32)  [unwired: 11 in]
              n620 = call "myRIO_BRig_RT_dataExp_nTrial.vi"() -> ("output_nTrial"=w1289:i32)  [unwired: 11 in]
              n621 = call "myRIO_BRig_RT_dataExp_runTime_seconds.vi"() -> ("output_RunTime_minutes"=w1288:i32)  [unwired: 11 in]
              n622 = call "myRIO_BRig_RT_dataExp_Tcycle_Selection.vi"() -> ("output_Tcycle_Selection"=w1287:i32)  [unwired: 11 in]
              n623 = call "myRIO_BRig_RT_dataExp_Tcycle_Reward__L.vi"() -> ("output_Tcycle_Reward__L"=w1285:i32)  [unwired: 11 in]
              n624 = call "myRIO_BRig_RT_dataExp_Tcycle_Reward__R.vi"() -> ("output_Tcycle_Reward__R"=w1283:i32)  [unwired: 11 in]
              n625 = local read "Tcycle_RewardPost"() -> (w1280:u16)
              n626 = local read "Tcycle_Wrong"() -> (w1278:u16)
              n627 = local read "Tcycle_Timeout"() -> (w1276:u16)
              n628 = local read "Tcycle_CuePenalty"() -> (w1266:u16)
              n629 = local read "Tcycle_Cue_max"() -> (w1254:u16)
              n630 = local read "Tcycle_Cue_min"() -> (w1255:u16)
              n631 = local read "Tcycle_Selection"() -> (w1286:u16)
              n632 = local read "Tcycle_Reward_L"() -> (w1284:u16)
              n633 = local read "Tcycle_Reward_R"() -> (w1282:u16)
              n634 = local read "SolenoidProbability_R"() -> (w1250:u16)
              n635 = local read "SolenoidProbability_L"() -> (w1251:u16)
              n636 = Replace Array Subset(array=w1292, new element #1=u16 0, index #1=w1290, new element #2=u16 0, index #2=w1289, new element #3=u16 0, index #3=w1288, new element #4=w1286, index #4=w1287, new element #5=w1284, index #5=w1285, new element #6=w1282, index #6=w1283, new element #7=w1280, index #7=w1281, new element #8=w1278, index #8=w1279, new element #9=w1276, index #9=w1277, new element #10=w1255, index #10=w1275, new element #11=w1254, index #11=w1274, new element #12=w1266, index #12=w1273, new element #13=w1251, index #13=w1253, new element #14=w1250, index #14=w1252) -> (w1291:u16[])
            }
            frame "saveSettings3" {
              w1302 = 100.0 ("y")
              n637 = call "myRIO_BRig_RT_dataExp_laser_Freq.vi"() -> ("output_laser_Freq"=w1335:i32)  [unwired: 11 in]
              n638 = call "myRIO_BRig_RT_dataExp_laser_Tpeak.vi"() -> ("output_laser_Tpeak"=w1330:i32)  [unwired: 11 in]
              n639 = call "myRIO_BRig_RT_dataExp_laser_Tshutter.vi"() -> ("output_laser_Tshutter"=w1325:i32)  [unwired: 11 in]
              n640 = call "myRIO_BRig_RT_dataExp_laser_f_millisec2count.vi"() -> ("output_laser_f_millisec2count"=w1320:i32)  [unwired: 11 in]
              n641 = call "myRIO_BRig_RT_dataExp_laser_Power_min.vi"() -> ("output_laser_Power_min"=w1315:i32)  [unwired: 11 in]
              n642 = call "myRIO_BRig_RT_dataExp_laser_Power_max.vi"() -> ("output_laser_Power_max"=w1308:i32)  [unwired: 11 in]
              n643 = call "myRIO_BRig_RT_dataExp_laser_Power_step.vi"() -> ("output_laser_Power_step"=w1307:i32)  [unwired: 11 in]
              n644 = call "myRIO_BRig_RT_dataExp_laser_duration.vi"() -> ("output_laser_duration"=w1310:i32)  [unwired: 11 in]
              n645 = call "myRIO_BRig_RT_dataExp_BUR_min.vi"() -> ("output_BUR_min"=w1357:i32)  [unwired: 11 in]
              n646 = call "myRIO_BRig_RT_dataExp_BUR_max.vi"() -> ("output_BUR_max"=w1355:i32)  [unwired: 11 in]
              n647 = call "myRIO_BRig_RT_dataExp_Audio_sp__L.vi"() -> ("output_Audio_sp__L"=w1352:i32)  [unwired: 11 in]
              n648 = call "myRIO_BRig_RT_dataExp_Audio_sp__R.vi"() -> ("output_Audio_sp__R"=w1351:i32)  [unwired: 11 in]
              n649 = local read "laser_Tshutter"() -> (w1322:dbl)
              n650 = local read "f_millisec2count"() -> (w1317:dbl)
              n651 = local read "laser_Tpeak"() -> (w1327:dbl)
              n652 = local read "laser_power_min"() -> (w1312:dbl)
              n653 = local read "laser_power_max"() -> (w1301:dbl)
              n654 = local read "laser_power_step"() -> (w1300:dbl)
              n655 = local read "laser_Freq"() -> (w1334:dbl)
              n656 = local read "sp_LeftSpout"() -> (w1350:u16)
              n657 = local read "BUR_max"() -> (w1354:u16)
              n658 = local read "sp_RightSpout"() -> (w1349:u16)
              n659 = local read "BUR_min"() -> (w1356:u16)
              n660 = Multiply(x=w1334, y=w1302) -> (x*y=w1333:dbl)
              n661 = Multiply(x=w1327, y=w1302) -> (x*y=w1329:dbl)
              n662 = Multiply(x=w1322, y=w1302) -> (x*y=w1324:dbl)
              n663 = Multiply(x=w1317, y=w1302) -> (x*y=w1319:dbl)
              n664 = Multiply(x=w1312, y=w1302) -> (x*y=w1314:dbl)
              n665 = Multiply(x=w1301, y=w1302) -> (x*y=w1306:dbl)
              n666 = Multiply(x=w1300, y=w1302) -> (x*y=w1304:dbl)
              n667 = Round To Nearest(number=w1333) -> (nearest integer value=w1332:dbl)
              n668 = Round To Nearest(number=w1329) -> (nearest integer value=w1328:dbl)
              n669 = Round To Nearest(number=w1324) -> (nearest integer value=w1323:dbl)
              n670 = Round To Nearest(number=w1319) -> (nearest integer value=w1318:dbl)
              n671 = Round To Nearest(number=w1314) -> (nearest integer value=w1313:dbl)
              n672 = Round To Nearest(number=w1306) -> (nearest integer value=w1305:dbl)
              n673 = Round To Nearest(number=w1304) -> (nearest integer value=w1303:dbl)
              n674 = To Unsigned Word Integer(number=w1332) -> (unsigned 16bit integer=w1331:u16)
              n675 = To Unsigned Word Integer(number=w1328) -> (unsigned 16bit integer=w1326:u16)
              n676 = To Unsigned Word Integer(number=w1323) -> (unsigned 16bit integer=w1321:u16)
              n677 = To Unsigned Word Integer(number=w1318) -> (unsigned 16bit integer=w1316:u16)
              n678 = To Unsigned Word Integer(number=w1313) -> (unsigned 16bit integer=w1311:u16)
              n679 = To Unsigned Word Integer(number=w1305) -> (unsigned 16bit integer=w1299:u16)
              n680 = To Unsigned Word Integer(number=w1303) -> (unsigned 16bit integer=w1298:u16)
              n681 = local read "laser_duration"() -> (w1309:u16)
              n682 = call "myRIO_BRig_RT_dataCurrent_LaserPulse_duration.vi"() -> ("output_LaserPulse_duration"=w1336:i32)  [unwired: 11 in]
              n683 = Replace Array Subset(array=w1358, new element #1=w1356, index #1=w1357, new element #2=w1354, index #2=w1355, new element #3=w1350, index #3=w1352, new element #4=w1349, index #4=w1351, new element #5=w1331, index #5=w1335, new element #6=w1326, index #6=w1330, new element #7=w1321, index #7=w1325, new element #8=w1316, index #8=w1320, new element #9=w1311, index #9=w1315, new element #10=w1299, index #10=w1308, new element #11=w1298, index #11=w1307, new element #12=w1309, index #12=w1310) -> (w1353:u16[])
              n684 = Replace Array Subset(array=w1338, new element=w1309, index=w1336) -> (w1337:u16[])
            }
            frame "saveSettings4_LC_ENL" {
              # "delayOpt"
              # "Count"
              # "Tdelay"
              # "Probability"
              # "OnOff"
              # "Block"
              # "ENL1 All"
              # "delayOpt"
              # "Count"
              # "Tdelay"
              # "Probability"
              # "OnOff"
              # "Block"
              # "ENL1 First"
              n685 = call "myRIO_BRig_RT_dataLC_ENL1_All_Block.vi"() -> ("output_ENL1_All_Block"=w1381:i32)  [unwired: 11 in]
              n686 = call "myRIO_BRig_RT_dataLC_ENL1_All_OnOff.vi"() -> ("output_ENL1_All_OnOff"=w1370:i32)  [unwired: 11 in]
              n687 = call "myRIO_BRig_RT_dataLC_ENL1_All_Probability.vi"() -> ("output_ENL1_All_Probability"=w1369:i32)  [unwired: 11 in]
              n688 = call "myRIO_BRig_RT_dataLC_ENL1_All_Tdelay.vi"() -> ("output_ENL1_All_Tdelay"=w1368:i32)  [unwired: 11 in]
              n689 = call "myRIO_BRig_RT_dataLC_ENL1_All_Count.vi"() -> ("output_ENL1_All_Count"=w1367:i32)  [unwired: 11 in]
              n690 = call "myRIO_BRig_RT_dataLC_ENL1_All_delayOpt.vi"() -> ("output_ENL1_All_delayOpt"=w1366:i32)  [unwired: 11 in]
              n691 = call "myRIO_BRig_RT_dataLC_ENL1_First_Block.vi"() -> ("output_ENL1_First_Block"=w1407:i32)  [unwired: 11 in]
              n692 = call "myRIO_BRig_RT_dataLC_ENL1_First_OnOff.vi"() -> ("output_ENL1_First_OnOff"=w1405:i32)  [unwired: 11 in]
              n693 = call "myRIO_BRig_RT_dataLC_ENL1_First_Probability.vi"() -> ("output_ENL1_First_Probability"=w1401:i32)  [unwired: 11 in]
              n694 = call "myRIO_BRig_RT_dataLC_ENL1_First_Tdelay.vi"() -> ("output_ENL1_First_Tdelay"=w1399:i32)  [unwired: 11 in]
              n695 = call "myRIO_BRig_RT_dataLC_ENL1_First_Count.vi"() -> ("output_ENL1_First_Count"=w1397:i32)  [unwired: 11 in]
              n696 = call "myRIO_BRig_RT_dataLC_ENL1_First_delayOpt.vi"() -> ("output_ENL1_First_delayOpt"=w1383:i32)  [unwired: 11 in]
              n697 = local read "LC_ENL1_First_delayOpt"() -> (w1384:bool)
              n698 = local read "LC_ENL1_First_Count"() -> (w1396:u16)
              n699 = local read "LC_ENL1_First_Probability"() -> (w1400:u16)
              n700 = local read "LC_ENL1_First_Block"() -> (w1406:u16)
              n701 = local read "LC_ENL1_First_Tdelay"() -> (w1398:u16)
              n702 = local read "LC_ENL1_First_OnOff"() -> (w1404:bool)
              n703 = local read "LC_ENL1_All_OnOff"() -> (w1377:bool)
              n704 = local read "LC_ENL1_All_Probability"() -> (w1375:u16)
              n705 = local read "LC_ENL1_All_delayOpt"() -> (w1372:bool)
              n706 = local read "LC_ENL1_All_Tdelay"() -> (w1374:u16)
              n707 = local read "LC_ENL1_All_Block"() -> (w1378:u16)
              n708 = local read "LC_ENL1_All_Count"() -> (w1373:u16)
              n709 = Boolean To (0,1)(Boolean=w1384) -> (0, 1=w1385:i16)
              n710 = Boolean To (0,1)(Boolean=w1404) -> (0, 1=w1403:i16)
              n711 = Boolean To (0,1)(Boolean=w1377) -> (0, 1=w1380:i16)
              n712 = To Unsigned Word Integer(number=w1385) -> (unsigned 16bit integer=w1382:u16)
              n713 = To Unsigned Word Integer(number=w1403) -> (unsigned 16bit integer=w1402:u16)
              n714 = Boolean To (0,1)(Boolean=w1372) -> (0, 1=w1379:i16)
              n715 = To Unsigned Word Integer(number=w1380) -> (unsigned 16bit integer=w1376:u16)
              n716 = To Unsigned Word Integer(number=w1379) -> (unsigned 16bit integer=w1371:u16)
              n717 = Replace Array Subset(array=w1408, new element #1=w1406, index #1=w1407, new element #2=w1402, index #2=w1405, new element #3=w1400, index #3=w1401, new element #4=w1398, index #4=w1399, new element #5=w1396, index #5=w1397, new element #6=w1382, index #6=w1383, new element #7=w1378, index #7=w1381, new element #8=w1376, index #8=w1370, new element #9=w1375, index #9=w1369, new element #10=w1374, index #10=w1368, new element #11=w1373, index #11=w1367, new element #12=w1371, index #12=w1366) -> (w1409:u16[])
            }
            frame "saveSettings5_LC_Cue" {
              # "delayOpt"
              # "Count"
              # "Tdelay"
              # "Probability"
              # "OnOff"
              # "Block"
              # "Cue1 All"
              # "delayOpt"
              # "Count"
              # "Tdelay"
              # "Probability"
              # "OnOff"
              # "Block"
              # "Cue1 First"
              n718 = call "myRIO_BRig_RT_dataLC_Cue1_First_delayOpt.vi"() -> ("output_Cue1_First_delayOpt"=w1436:i32)  [unwired: 11 in]
              n719 = call "myRIO_BRig_RT_dataLC_Cue1_First_Block.vi"() -> ("output_Cue1_First_Block"=w1459:i32)  [unwired: 11 in]
              n720 = call "myRIO_BRig_RT_dataLC_Cue1_First_OnOff.vi"() -> ("output_Cue1_First_OnOff"=w1457:i32)  [unwired: 11 in]
              n721 = call "myRIO_BRig_RT_dataLC_Cue1_First_Probability.vi"() -> ("output_Cue1_First_Probability"=w1453:i32)  [unwired: 11 in]
              n722 = call "myRIO_BRig_RT_dataLC_Cue1_First_Tdelay.vi"() -> ("output_Cue1_First_Tdelay"=w1451:i32)  [unwired: 11 in]
              n723 = call "myRIO_BRig_RT_dataLC_Cue1_First_Count.vi"() -> ("output_Cue1_First_Count"=w1449:i32)  [unwired: 11 in]
              n724 = call "myRIO_BRig_RT_dataLC_Cue1_All_Block.vi"() -> ("output_Cue1_All_Block"=w1433:i32)  [unwired: 11 in]
              n725 = call "myRIO_BRig_RT_dataLC_Cue1_All_OnOff.vi"() -> ("output_Cue1_All_OnOff"=w1432:i32)  [unwired: 11 in]
              n726 = call "myRIO_BRig_RT_dataLC_Cue1_All_Probability.vi"() -> ("output_Cue1_All_Probability"=w1431:i32)  [unwired: 11 in]
              n727 = call "myRIO_BRig_RT_dataLC_Cue1_All_Tdelay.vi"() -> ("output_Cue1_All_Tdelay"=w1430:i32)  [unwired: 11 in]
              n728 = call "myRIO_BRig_RT_dataLC_Cue1_All_Count.vi"() -> ("output_Cue1_All_Count"=w1429:i32)  [unwired: 11 in]
              n729 = call "myRIO_BRig_RT_dataLC_Cue1_All_delayOpt.vi"() -> ("output_Cue1_All_delayOpt"=w1428:i32)  [unwired: 11 in]
              n730 = local read "LC_Cue1_First_delayOpt"() -> (w1435:bool)
              n731 = local read "LC_Cue1_First_Count"() -> (w1448:u16)
              n732 = local read "LC_Cue1_First_Probability"() -> (w1452:u16)
              n733 = local read "LC_Cue1_First_Block"() -> (w1458:u16)
              n734 = local read "LC_Cue1_First_Tdelay"() -> (w1450:u16)
              n735 = local read "LC_Cue1_First_OnOff"() -> (w1456:bool)
              n736 = local read "LC_Cue1_All_OnOff"() -> (w1424:bool)
              n737 = local read "LC_Cue1_All_delayOpt"() -> (w1425:bool)
              n738 = local read "LC_Cue1_All_Probability"() -> (w1421:u16)
              n739 = local read "LC_Cue1_All_Tdelay"() -> (w1420:u16)
              n740 = local read "LC_Cue1_All_Count"() -> (w1419:u16)
              n741 = local read "LC_Cue1_All_Block"() -> (w1423:u16)
              n742 = Boolean To (0,1)(Boolean=w1435) -> (0, 1=w1437:i16)
              n743 = Boolean To (0,1)(Boolean=w1456) -> (0, 1=w1455:i16)
              n744 = Boolean To (0,1)(Boolean=w1424) -> (0, 1=w1427:i16)
              n745 = To Unsigned Word Integer(number=w1437) -> (unsigned 16bit integer=w1434:u16)
              n746 = To Unsigned Word Integer(number=w1455) -> (unsigned 16bit integer=w1454:u16)
              n747 = To Unsigned Word Integer(number=w1427) -> (unsigned 16bit integer=w1422:u16)
              n748 = Boolean To (0,1)(Boolean=w1425) -> (0, 1=w1426:i16)
              n749 = To Unsigned Word Integer(number=w1426) -> (unsigned 16bit integer=w1418:u16)
              n750 = Replace Array Subset(array=w1460, new element #1=w1458, index #1=w1459, new element #2=w1454, index #2=w1457, new element #3=w1452, index #3=w1453, new element #4=w1450, index #4=w1451, new element #5=w1448, index #5=w1449, new element #6=w1434, index #6=w1436, new element #7=w1423, index #7=w1433, new element #8=w1422, index #8=w1432, new element #9=w1421, index #9=w1431, new element #10=w1420, index #10=w1430, new element #11=w1419, index #11=w1429, new element #12=w1418, index #12=w1428) -> (w1461:u16[])
            }
            frame "saveSettings6_LC_Other" {
              # "Trial"
              # "Tdelay"
              # "Probability"
              # "OnOff"
              # "Block"
              # "Wrong"
              # "Trial"
              # "Tdelay"
              # "Probability"
              # "OnOff"
              # "Block"
              # "Reward"
              n751 = call "myRIO_BRig_RT_dataLC_Wrong_Block.vi"() -> ("output_Wrong_Block"=w1491:i32)  [unwired: 11 in]
              n752 = call "myRIO_BRig_RT_dataLC_Wrong_OnOff.vi"() -> ("output_Wrong_OnOff"=w1490:i32)  [unwired: 11 in]
              n753 = call "myRIO_BRig_RT_dataLC_Wrong_Probability.vi"() -> ("output_Wrong_Probability"=w1489:i32)  [unwired: 11 in]
              n754 = call "myRIO_BRig_RT_dataLC_Wrong_Tdelay.vi"() -> ("output_Wrong_Tdelay"=w1488:i32)  [unwired: 11 in]
              n755 = call "myRIO_BRig_RT_dataLC_Wrong_Trial.vi"() -> ("output_Wrong_Trial"=w1487:i32)  [unwired: 11 in]
              n756 = call "myRIO_BRig_RT_dataLC_Reward_Block.vi"() -> ("output_Reward_Block"=w1503:i32)  [unwired: 11 in]
              n757 = call "myRIO_BRig_RT_dataLC_Reward_OnOff.vi"() -> ("output_Reward_OnOff"=w1501:i32)  [unwired: 11 in]
              n758 = call "myRIO_BRig_RT_dataLC_Reward_Probability.vi"() -> ("output_Reward_Probability"=w1497:i32)  [unwired: 11 in]
              n759 = call "myRIO_BRig_RT_dataLC_Reward_Tdelay.vi"() -> ("output_Reward_Tdelay"=w1495:i32)  [unwired: 11 in]
              n760 = call "myRIO_BRig_RT_dataLC_Reward_Trial.vi"() -> ("output_Reward_Trial"=w1493:i32)  [unwired: 11 in]
              n761 = local read "LC_Wrong_OnOff"() -> (w1485:bool)
              n762 = local read "LC_Wrong_Probability"() -> (w1482:u16)
              n763 = local read "LC_Wrong_Block"() -> (w1484:u16)
              n764 = local read "LC_Wrong_Tdelay"() -> (w1481:u16)
              n765 = local read "LC_Wrong_Trial"() -> (w1480:u16)
              n766 = local read "LC_Reward_Probability"() -> (w1496:u16)
              n767 = local read "LC_Reward_Block"() -> (w1502:u16)
              n768 = local read "LC_Reward_Tdelay"() -> (w1494:u16)
              n769 = local read "LC_Reward_OnOff"() -> (w1500:bool)
              n770 = local read "LC_Reward_Trial"() -> (w1492:u16)
              n771 = Boolean To (0,1)(Boolean=w1485) -> (0, 1=w1486:i16)
              n772 = Boolean To (0,1)(Boolean=w1500) -> (0, 1=w1499:i16)
              n773 = To Unsigned Word Integer(number=w1486) -> (unsigned 16bit integer=w1483:u16)
              n774 = To Unsigned Word Integer(number=w1499) -> (unsigned 16bit integer=w1498:u16)
              n775 = Replace Array Subset(array=w1504, new element #1=w1502, index #1=w1503, new element #2=w1498, index #2=w1501, new element #3=w1496, index #3=w1497, new element #4=w1494, index #4=w1495, new element #5=w1492, index #5=w1493, new element #6=w1484, index #6=w1491, new element #7=w1483, index #7=w1490, new element #8=w1482, index #8=w1489, new element #9=w1481, index #9=w1488, new element #10=w1480, index #10=w1487) -> (w1505:u16[])
            }
            frame "setSettings_Audio" {
              # "amp_L"
              # "amp_R"
              # "freq_L"
              # "freq_R"
              n776 = call "myRIO_BRig_RT_dataExp_Audio_amp__L.vi"() -> ("output_Audio_amp__L"=w1530:i32)  [unwired: 11 in]
              n777 = call "myRIO_BRig_RT_dataExp_Audio_amp__R.vi"() -> ("output_Audio_amp__R"=w1529:i32)  [unwired: 11 in]
              n778 = call "myRIO_BRig_RT_dataExp_Audio_freq__L.vi"() -> ("output_Audio_freq__L"=w1528:i32)  [unwired: 11 in]
              n779 = call "myRIO_BRig_RT_dataExp_Audio_freq__R.vi"() -> ("output_Audio_freq__R"=w1527:i32)  [unwired: 11 in]
              n780 = Index Array(array=w1526, index #1=w1530, index #2=w1529, index #3=w1528, index #4=w1527) -> (element #1=w1525:u16, element #2=w1524:u16, element #3=w1517:u16, element #4=w1515:u16)
              n781 = To Unsigned Byte Integer(number=w1517) -> (unsigned 8bit integer=w1516:u8)
              n782 = To Unsigned Byte Integer(number=w1515) -> (unsigned 8bit integer=w1514:u8)
            }
            frame "setSettings_Laser" {
              (unwired) u32 0 ("tDelay_laser_rew")
              # "Wrong tDelay"
              # "Reward tDelay"
              n783 = call "myRIO_BRig_RT_dataLC_Reward_Tdelay.vi"() -> ("output_Reward_Tdelay"=w1557:i32)  [unwired: 11 in]
              n784 = call "myRIO_BRig_RT_dataLC_Wrong_Tdelay.vi"() -> ("output_Wrong_Tdelay"=w1558:i32)  [unwired: 11 in]
              n785 = Index Array(array=w1554, index #1=w1557, index #2=w1558) -> (element #1=w1556:u16, element #2=w1555:u16)
              n786 = call "myRIO_BRig_RT__calc_Tvalley.vi"("input_peakWidth"="laser_Tpeak", "input_freq"="laser_Freq") -> ("output_Tvalley"=w1564:dbl)  [unwired: 9 in]
              n787 = To Double Precision Float(number=w1556) -> (double precision float=w1551:dbl)
              n788 = To Double Precision Float(number=w1555) -> (double precision float=w1548:dbl)
              n789 = Multiply(x="f_millisec2count", y="laser_Tpeak") -> (x*y=w1573:dbl)
              n790 = Multiply(x="f_millisec2count", y=w1564) -> (x*y=w1570:dbl)
              n791 = Multiply(x="f_millisec2count", y="laser_Tshutter") -> (x*y=w1568:dbl)
              n792 = Round Toward +Infinity(x="laser_Tshutter") -> (ceil(x): smallest int >= x=w1559:dbl)
              n793 = Multiply(x="f_millisec2count", y=w1551) -> (x*y=w1552:dbl)
              n794 = Multiply(x="f_millisec2count", y=w1548) -> (x*y=w1549:dbl)
              n795 = To Unsigned Word Integer(number="f_millisec2count") -> (unsigned 16bit integer=w1539:u16)
              n796 = Round Toward +Infinity(x=w1573) -> (ceil(x): smallest int >= x=w1574:dbl)
              n797 = Round Toward +Infinity(x=w1570) -> (ceil(x): smallest int >= x=w1571:dbl)
              n798 = Round Toward +Infinity(x=w1568) -> (ceil(x): smallest int >= x=w1563:dbl)
              n799 = Round Toward +Infinity(x=w1552) -> (ceil(x): smallest int >= x=w1553:dbl)
              n800 = Round Toward +Infinity(x=w1549) -> (ceil(x): smallest int >= x=w1550:dbl)
              n801 = To Unsigned Long Integer(number=w1574) -> (unsigned 32bit integer=w1572:u32)
              n802 = To Unsigned Long Integer(number=w1571) -> (unsigned 32bit integer=w1569:u32)
              n803 = To Unsigned Long Integer(number=w1563) -> (unsigned 32bit integer=w1567:u32)
              n804 = To Unsigned Word Integer(number=w1559) -> (unsigned 16bit integer=w1562:u16)
              n805 = To Unsigned Long Integer(number=w1553) -> (unsigned 32bit integer=w1547:u32)
              n806 = To Unsigned Long Integer(number=w1550) -> (unsigned 32bit integer=w1546:u32)
              n807 = Add(x="laser_duration", y=w1562) -> (x+y=w1543:u16)
              n808 = To Double Precision Float(number=w1543) -> (double precision float=w1542:dbl)
              n809 = Multiply(x=w1542, y="f_millisec2count") -> (x*y=w1544:dbl)
              n810 = call "myRIO_BRig_RT_dataCurrent_LaserPulse_duration.vi"() -> ("output_LaserPulse_duration"=w1575:i32)  [unwired: 11 in]
              n811 = Round Toward +Infinity(x=w1544) -> (ceil(x): smallest int >= x=w1545:dbl)
              n812 = To Unsigned Long Integer(number=w1545) -> (unsigned 32bit integer=w1541:u32)
              n813 = xnode "Read/Write Control"("FPGA VI Reference In"=w1577, "error in"=w1578, "laser_Npeak"=w1572, "laser_Nvalley"=w1569, "laser_Nshutter"=w1567, "laser_selRew_Ndelay"=w1547, "laser_selWro_NDelay"=w1546, "laser_selRew_Ntotal"=w1541, "laser_selWro_Ntotal"=w1541, "k1__counter_per_ms"=w1539) -> ("error out"=→"error out":errorcluster)  [unwired: 1 out]
              n814 = Replace Array Subset(array=w1554, new element=w1543, index=w1575) -> (w1576:u16[])
            }
            frame "initBlock" {
              n815 = call "myRIO_Brig_RT__Case_Exp_State_initBlock.vi"("input_spout"=w1621, "input_dataExp"=w1619, "input_dataCurrent"=w1620) -> ("output_spout"=w1598:enum16{"Left", "Right"}, "output_state"=w1622:T2, "output_dataExp"=w1618:u16[], "output_dataCurrent"=w1604:u16[], "output_TpB_target"=→"TpB_target":u16)  [unwired: 4 in]
              "cSpout" <- w1598
              n816 = call "myRIO_BRig_RT_dataCurrent_iBlock.vi"() -> ("output_iBlock"=w1603:i32)  [unwired: 11 in]
              n817 = Index Array(array=w1604, index=w1603) -> (element=→"iBlock":u16)
            }
            frame "initBlock2" {
              n818 = local write "nRewards_cur"(u16 0 ("nRewards_cur")) -> ()
              n819 = call "myRIO_BRig_RT__Case_Exp_State_initBlock2.vi"("input_spout"=w1630, "input_dataBlock"=w1631, "input_dataCurrent"=w1629) -> ("idxDataBlock"=w1626:i32, "output_dataBlock"=w1628:u16[][])  [unwired: 7 in]
            }
            frame "initTrial" {
              n820 = call "myRIO_Brig_RT__Case_Exp_State_initTrial.vi"("input_spout"=w1647, "input_dataExp"=w1664, "input_dataCurrent"=w1665) -> ("output_state"=w1666:T2, "output_dataExp"=w1663:u16[], "output_dataCurrent"=w1653:u16[])  [unwired: 6 in]
              n821 = call "myRIO_BRig_RT_dataCurrent_iTrial.vi"() -> ("output_iTrial"=w1652:i32)  [unwired: 11 in]
              n822 = call "myRIO_BRig_RT_dataCurrent_SolenoidReward.vi"() -> ("output_SolenoidReward"=w1646:i32)  [unwired: 11 in]
              n823 = Index Array(array=w1653, index #1=w1652, index #2=w1646) -> (element #1=→"iTrial":u16, element #2=w1645:u16)
              n824 = Not Equal To 0?(x=w1645) -> (x != 0?=→"SolenoidReward":bool)
            }
            frame "initTrial2" {
              # "trialUntilReward"
              n825 = call "myRIO_BRig_RT__Case_Exp_subState_LC__initTrial.vi"("input_dataTrial"=w1673, "input_spout"=w1682, "input_dataCurrent"=w1671, "input_dataLC"=w1670) -> ("output_LC_Wrong"=w1683:bool, "output_LC_led_Wrong"=w1675:bool, "output_LC_Reward"=w1684:bool, "output_LC_led_Reward"=w1674:bool, "output_dataTrial"=w1672:u16[][])  [unwired: 2 in]
              n826 = Equal?(x=w1682, y=enum16{"Left", "Right"}."Right") -> (x = y?=w1680:bool)
              n827 = call "myRIO_BRig_RT_dataExp_ItrialUntilReward.vi"() -> ("output_I_trialUntilReward"=w1678:i32)  [unwired: 11 in]
              n828 = Index Array(array=w1679, index=w1678) -> (element=w1677:u16)
              n829 = Not Equal To 0?(x=w1677) -> (x != 0?=w1676:bool)
              n830 = xnode "Read/Write Control"("FPGA VI Reference In"=w1697, "error in"=w1696, "SelectionState"=FALSE, "laserResponse_reward"=w1684, "laserResponse_wrong"=w1683, "laserResponse_reward_LED"=w1674, "laserResponse_wrong_LED"=w1675, "Left(F)_or_Right(T)"=w1680, "ignoreWrong"=w1676) -> ("error out"=→"error_initTrial":errorcluster)  [unwired: 1 out]
            }
            frame "initTrial3" {
              n831 = call "myRIO_BRig_RT__Case_Exp_State_initTrial_dataTrial.vi"("input_spout"=w1712, "input_dataCurrent"=w1713, "input_dataExp"=w1711, "input_dataTrial"=w1715) -> ("output_dataTrial"=w1714:u16[][], "output_laserPower"=w1708:u16)  [unwired: 6 in]
              n832 = To Double Precision Float(number=w1708) -> (double precision float=w1710:dbl)
              n833 = Divide(x=w1710, y=100.0 ("x")) -> (x/y=w1704:dbl)
              "output_PortA" <- w1704
              n834 = call "myRIO_Brig_RT__covert_Voltage_to_FPGAvalue.vi"("input_voltage"=w1704) -> ("output_PortC"=w1703:i16)  [unwired: 9 in, 1 out]
              n835 = xnode "Read/Write Control"("FPGA VI Reference In"=w1707, "error in"=w1706, "AnaOut_0"=w1703) -> ("error out"=→"error out 4":errorcluster)  [unwired: 1 out]
            }
            frame "initTrial4" {
              n836 = call "myRIO_BRig_RT_dataCurrent_idxDataTrial.vi"() -> ("output_idxDataTrial"=w1738:i32)  [unwired: 11 in]
              n837 = call "myRIO_BRig_RT_dataTrial_activeRecording.vi"() -> ("output_activeRecording"=w1735:i32)  [unwired: 11 in]
              n838 = Index Array(array=w1740, index=w1738) -> (element=w1737:u16)
              n839 = Boolean To (0,1)(Boolean="Recording") -> (0, 1=w1734:i16)
              n840 = To Long Integer(number=w1737) -> (32bit integer=w1736:i32)
              n841 = To Unsigned Word Integer(number=w1734) -> (unsigned 16bit integer=w1733:u16)
              n842 = Replace Array Subset(array=w1739, new element=w1733, index (row)=w1736, index (col)=w1735) -> (w1732:u16[][])
              n843 = local write "Recording_p2"("Recording") -> ()
            }
            frame "initTrial_LC_ENL1" {
              n844 = call "myRIO_BRig_RT__Case_Exp_State_initTrial_LC_ENL1__v2.vi"("input_dataTrial"=w1764, "input_spout"=w1769, "input_dataBlock"=w1762, "input_dataLC"=w1770, "input_dataCurrent"=w1766) -> ("output_LC__ENL1"=w1768:bool, "output_LC_led__ENL1"=w1767:bool, "output_dataTrial"=w1763:u16[][], "output_dataCurrent"=w1765:u16[])  [unwired: 3 in]
            }
            frame "initTrial_LC_Cue1" {
              n845 = local write "Recording_p2"(FALSE ("Recording_p2")) -> ()
              n846 = call "myRIO_BRig_RT__Case_Exp_State_initTrial_LC_Cue1__v2.vi"("input_dataTrial"=w1792, "input_spout"=w1795, "input_dataBlock"=w1790, "input_dataLC"=w1796, "input_dataCurrent"=w1794) -> ("output_LC__Cue1"=w1788:bool, "output_LC_led__Cue1"=w1789:bool, "output_dataTrial"=w1791:u16[][], "output_dataCurrent"=w1793:u16[])  [unwired: 3 in]
            }
            frame "ENL1_pre" {
              # "ENL1_n"
              # "Tcycle"
              # "counter"
              n847 = call "myRIO_BRig_RT_dataCurrent_Tcycle_generic.vi"() -> ("output_Tcycle_generic"=w1842:i32)  [unwired: 11 in]
              n848 = call "myRIO_BRig_RT_dataCurrent_count_generic.vi"() -> ("output_count_generic"=w1844:i32)  [unwired: 11 in]
              n849 = call "myRIO_BRig_RT_dataCurrent_ENL.vi"() -> ("output_ENL"=w1841:i32)  [unwired: 11 in]
              n850 = call "myRIO_BRig_RT_dataCurrent_ENL1_n.vi"() -> ("output_ENL1_n"=w1813:i32)  [unwired: 11 in]
              n851 = Index Array(array=w1835, index #1=w1841, index #2=w1813) -> (element #1=w1840:u16, element #2=w1812:u16)
              n852 = Increment(x=w1812) -> (x+1=w1811:u16)
              n853 = Replace Array Subset(array=w1835, new element #1=u16 0 ("new element/subarray"), index #1=w1844, new element #2=w1840, index #2=w1842, new element #3=w1811, index #3=w1813) -> (w1839:u16[])
              n854 = Select(t=myRIO_BRig_RT__Case_Exp_stateList."ENL1Penalty_pre" ("Enum"), s=w1823, f=myRIO_BRig_RT__Case_Exp_stateList."ENL1" ("Enum")) -> (s? t:f=w1820:T2)
            }
            frame "ENL1" {
              n855 = call "myRIO_BRig_RT__Case_Exp_State_ENL1__v2.vi"("input_LC"=w1851, "I_lick"=w1855, "input_LC_led"=w1852, "input_laserOccurred"=w1847, "input_state"=w1861, "input_dataCurrent"=w1860) -> ("output_trigger_laser_led"=w1850:bool, "output_state"=w1858:T2, "output_dataCurrent"=w1859:u16[], "output_trigger_laser"=w1849:bool)  [unwired: 2 in]
              n856 = Or(x=w1850, y=w1847) -> (x .or. y?=w1853:bool)
            }
            frame "ENL1Penalty_pre" {
              # "Tcycle"
              # "counter"
              n857 = call "myRIO_BRig_RT_dataCurrent_Tcycle_generic.vi"() -> ("output_Tcycle_generic"=w1901:i32)  [unwired: 11 in]
              n858 = call "myRIO_BRig_RT_dataCurrent_count_generic.vi"() -> ("output_count_generic"=w1903:i32)  [unwired: 11 in]
              n859 = call "myRIO_BRig_RT_dataExp_ENL_penalty.vi"() -> ("output_ENL_penalty"=w1896:i32)  [unwired: 11 in]
              n860 = Index Array(array=w1897, index=w1896) -> (element=w1900:u16)
              n861 = Replace Array Subset(array=w1898, new element #1=u16 0 ("new element/subarray"), index #1=w1903, new element #2=w1900, index #2=w1901) -> (w1899:u16[])
            }
            frame "ENL1Penalty" {
              n862 = call "myRIO_BRig_RT__Case_Exp_State_ENL1Penalty.vi"("input_state"=w1926, "input_dataCurrent"=w1930) -> ("output_state"=w1927:T2, "output_dataCurrent"=w1929:u16[])  [unwired: 8 in]
            }
            frame "ENL2_pre" {
            }
            frame "ENL2" {
            }
            frame "ENL2Penalty_pre" {
            }
            frame "ENL2Penalty" {
            }
            frame "Cue1_pre" {
              # "Cue1_n"
              # "Tcycle_Cue1"
              # "0 = L, 1 = R, 2 = both"
              # "sp_R"
              # "sp_L"
              # "Tcycle"
              # "counter"
              n863 = Equal?(x=w2041, y=enum16{"Left", "Right"}."Left") -> (x = y?=w2040:bool)
              n864 = call "myRIO_BRig_RT_dataExp_Audio_sp__L.vi"() -> ("output_Audio_sp__L"=w2039:i32)  [unwired: 11 in]
              n865 = call "myRIO_BRig_RT_dataExp_Audio_sp__R.vi"() -> ("output_Audio_sp__R"=w2038:i32)  [unwired: 11 in]
              n866 = call "myRIO_BRig_RT_dataCurrent_Tcycle_generic.vi"() -> ("output_Tcycle_generic"=w2051:i32)  [unwired: 11 in]
              n867 = call "myRIO_BRig_RT_dataCurrent_count_generic.vi"() -> ("output_count_generic"=w2053:i32)  [unwired: 11 in]
              n868 = Select(t=w2039, s=w2040, f=w2038) -> (s? t:f=w2037:i32)
              n869 = call "myRIO_BRig_RT_dataCurrent_Cue1_n.vi"() -> ("output_Cue1_n"=w2015:i32)  [unwired: 11 in]
              n870 = call "myRIO_BRig_RT_dataCurrent_Tcycle_cue.vi"() -> ("output_Tcycle_cue"=w2024:i32)  [unwired: 11 in]
              n871 = Index Array(array=w2043, index=w2037) -> (element=w2035:u16)
              n872 = Index Array(array=w2025, index #1=w2024, index #2=w2015) -> (element #1=w2026:u16, element #2=w2017:u16)
              n873 = Increment(x=w2017) -> (x+1=w2016:u16)
              n874 = Not Equal To 0?(x=w2035) -> (x != 0?=w2033:bool)
              n875 = Not Equal?(x=w2035, y=u16 1) -> (x != y?=w2034:bool)
              n876 = Replace Array Subset(array=w2025, new element #1=u16 0 ("new element/subarray"), index #1=w2053, new element #2=w2026, index #2=w2051, new element #3=w2016, index #3=w2015) -> (w2050:u16[])
              n877 = Select(t=myRIO_BRig_RT__Case_Exp_stateList."Cue1Penalty_pre" ("Enum"), s=w2021, f=myRIO_BRig_RT__Case_Exp_stateList."Cue1" ("Enum")) -> (s? t:f=w2022:T2)
            }
            frame "Cue1" {
              n878 = call "myRIO_BRig_RT__Case_Exp_State_Cue1__v2.vi"("input_LC"=w2063, "I_lick"=w2066, "input_LC_led"=w2064, "input_laserOccurred"=w2058, "input_state"=w2068, "input_dataCurrent"=w2086) -> ("output_trigger_laser_led"=w2061:bool, "output_state"=w2067:T2, "output_dataCurrent"=w2085:u16[], "output_trigger_laser"=w2062:bool)  [unwired: 2 in]
              n879 = Or(x=w2061, y=w2058) -> (x .or. y?=w2060:bool)
              n880 = Equal?(x=myRIO_BRig_RT__Case_Exp_stateList."Selection_pre", y=w2067) -> (x = y?=w2071:bool)
              n881 = xnode "Read/Write Control"("FPGA VI Reference In"=w2070, "error in"=w2069, "SelectionState"=w2071) -> ()  [unwired: 2 out]
            }
            frame "Cue1Penalty_pre" {
              # "Tcycle"
              # "counter"
              n882 = call "myRIO_BRig_RT_dataCurrent_Tcycle_generic.vi"() -> ("output_Tcycle_generic"=w2117:i32)  [unwired: 11 in]
              n883 = call "myRIO_BRig_RT_dataCurrent_count_generic.vi"() -> ("output_count_generic"=w2119:i32)  [unwired: 11 in]
              n884 = call "myRIO_BRig_RT_dataExp_Tcycle_CuePenalty.vi"() -> ("output_Tcycle_CuePenalty"=w2116:i32)  [unwired: 11 in]
              n885 = Index Array(array=w2111, index=w2116) -> (element=w2115:u16)
              n886 = Replace Array Subset(array=w2113, new element #1=u16 0 ("new element/subarray"), index #1=w2119, new element #2=w2115, index #2=w2117) -> (w2112:u16[])
            }
            frame "Cue1Penalty" {
              # "reset laserOccurred"
              n887 = call "myRIO_BRig_RT__Case_Exp_State_Cue1Penalty.vi"("input_state"=w2143, "input_dataCurrent"=w2144) -> ("output_state"=w2141:T2, "output_dataCurrent"=w2142:u16[])  [unwired: 8 in]
            }
            frame "Cue2_pre" {
              n888 = call "myRIO_BRig_RT__Case_Exp_subState_LC__Cue2.vi"("input_spout"=w2161, "input_dataCurrent"=w2162, "input_dataLC"=w2160) -> ()  [unwired: 6 in, 2 out]
            }
            frame "Cue2" {
            }
            frame "Cue2Penalty_pre" {
            }
            frame "Cue2Penalty" {
            }
            frame "Selection_pre" {
              # "Tcycle"
              # "counter"
              n889 = xnode "Read/Write Control"("FPGA VI Reference In"=w2233, "error in"=w2234) -> ("error out"=→"error_Selection_pre":errorcluster, "SelectReward"=w2226:bool, "SelectWrong"=w2228:bool)  [unwired: 1 out]
              n890 = call "myRIO_BRig_RT_dataCurrent_Tcycle_generic.vi"() -> ("output_Tcycle_generic"=w2255:i32)  [unwired: 11 in]
              n891 = call "myRIO_BRig_RT_dataCurrent_count_generic.vi"() -> ("output_count_generic"=w2257:i32)  [unwired: 11 in]
              n892 = call "myRIO_BRig_RT_dataExp_Tcycle_Selection.vi"() -> ("output_Tcycle_Selection"=w2254:i32)  [unwired: 11 in]
              n893 = Index Array(array=w2251, index=w2254) -> (element=w2253:u16)
              n894 = Replace Array Subset(array=w2249, new element #1=u16 0 ("new element/subarray"), index #1=w2257, new element #2=w2253, index #2=w2255) -> (w2252:u16[])
              n895 = Or(x=w2226, y=w2228) -> (x .or. y?=w2227:bool)
              n896 = Select(t=myRIO_BRig_RT__Case_Exp_stateList."SelectReward_pre" ("Enum"), s=w2226, f=myRIO_BRig_RT__Case_Exp_stateList."SelectWrong_pre" ("Enum")) -> (s? t:f=w2232:T2)
              n897 = Select(t=w2232, s=w2227, f=myRIO_BRig_RT__Case_Exp_stateList."Selection" ("Enum")) -> (s? t:f=w2229:T2)
            }
            frame "Selection" {
              # "counter\nSelection"
              # "increment"
              # "get Tcycle"
              # "get count"
              n898 = xnode "Read/Write Control"("FPGA VI Reference In"=w2282, "error in"=w2281) -> ("error out"=→"error_Selection":errorcluster, "SelectReward"=w2278:bool, "SelectWrong"=w2279:bool)  [unwired: 1 out]
              n899 = call "myRIO_BRig_RT_dataCurrent_Tcycle_generic.vi"() -> ("output_Tcycle_generic"=w2275:i32)  [unwired: 11 in]
              n900 = call "myRIO_BRig_RT_dataCurrent_count_generic.vi"() -> ("output_count_generic"=w2268:i32)  [unwired: 11 in]
              n901 = Index Array(array=w2276, index #1=w2275, index #2=w2268) -> (element #1=w2267:u16, element #2=w2274:u16)
              n902 = call "myRIO_BRig_RT__increment_u16.vi"() -> ("output_increment__u16"=w2273:u16)  [unwired: 11 in]
              n903 = Add(x=w2274, y=w2273) -> (x+y=w2269:u16)
              n904 = Greater?(x=w2267, y=w2269) -> (0:w2261:bool)
              n905 = Select(t=w2272, s=w2261, f=myRIO_BRig_RT__Case_Exp_stateList."SelectTimeout_pre" ("Enum")) -> (s? t:f=w2262:T2)
              n906 = Select(t=w2269, s=w2261, f=w2267) -> (s? t:f=w2265:u16)
              n907 = call "myRIO_BRig_RT_dataCurrent_count_selection.vi"() -> ("output_count_generic"=w2266:i32)  [unwired: 11 in]
              n908 = Select(t=myRIO_BRig_RT__Case_Exp_stateList."SelectReward_pre" ("Enum"), s=w2278, f=myRIO_BRig_RT__Case_Exp_stateList."SelectWrong_pre" ("Enum")) -> (s? t:f=w2277:T2)
              n909 = Replace Array Subset(array=w2276, new element #1=w2265, index #1=w2268, new element #2=w2265, index #2=w2266) -> (w2271:u16[])
              n910 = Or(x=w2278, y=w2279) -> (x .or. y?=w2260:bool)
              n911 = Select(t=w2277, s=w2260, f=w2262) -> (s? t:f=w2280:T2)
            }
            frame "SelectReward_pre" {
              # "iState"
              # "Tcycle\nReward"
              # "nRewTrials"
              # "Tcycle\nGeneric"
              # "counter"
              n912 = call "myRIO_BRig_RT_dataCurrent_nRewTrials.vi"() -> ("output_nRewTrials"=w2314:i32)  [unwired: 11 in]
              n913 = Equal?(x=w2323, y=enum16{"Left", "Right"}."Left") -> (x = y?=w2324:bool)
              n914 = Index Array(array=w2315, index=w2314) -> (element=w2313:u16)
              n915 = call "myRIO_BRig_RT_dataExp_Tcycle_Reward__L.vi"() -> ("output_Tcycle_Reward__L"=w2327:i32)  [unwired: 11 in]
              n916 = call "myRIO_BRig_RT_dataExp_Tcycle_Reward__R.vi"() -> ("output_Tcycle_Reward__R"=w2328:i32)  [unwired: 11 in]
              n917 = Increment(x=w2313) -> (x+1=w2312:u16)
              n918 = Select(t=w2327, s=w2324, f=w2328) -> (s? t:f=w2326:i32)
              n919 = call "myRIO_BRig_RT__Case_Exp_subState_LC__Reward.vi"("input_spout"=w2323, "input_dataCurrent"=w2315, "input_dataLC"=w2322) -> ()  [unwired: 6 in, 2 out]
              n920 = call "myRIO_BRig_RT_dataCurrent_count_generic.vi"() -> ("output_count_generic"=w2317:i32)  [unwired: 11 in]
              n921 = call "myRIO_BRig_RT_dataCurrent_Tcycle_generic.vi"() -> ("output_Tcycle_generic"=w2318:i32)  [unwired: 11 in]
              n922 = Index Array(array=w2329, index=w2326) -> (element=w2319:u16)
              n923 = call "myRIO_BRig_RT_dataCurrent_iState.vi"() -> ("output_iState"=w2307:i32)  [unwired: 11 in]
              n924 = Replace Array Subset(array=w2315, new element #1=w2312, index #1=w2314, new element #2=u16 0 ("new element/subarray"), index #2=w2317, new element #3=w2319, index #3=w2318, new element #4=u16 1 ("new element/subarray"), index #4=w2307) -> (w2330:u16[])
            }
            frame "SelectReward" {
              n925 = call "myRIO_BRig_RT__Case_Exp_State_Reward.vi"("input_dataCurrent"=w2351, "input_state"=w2348, "input_spout"=w2346) -> ("output_dataCurrent"=w2350:u16[], "output_state"=w2349:T2, "output__L"=w2344:bool, "output__R"=w2345:bool)  [unwired: 9 in]
            }
            frame "SelectRewardPost_pre" {
              # "nRewards"
              # "nRewTrials"
              # "Tcycle"
              # "counter"
              n926 = call "myRIO_BRig_RT_dataBlock_nRewards__L.vi"() -> ("output_nRewards__L"=w2367:i32)  [unwired: 11 in]
              n927 = call "myRIO_BRig_RT_dataBlock_nRewards__R.vi"() -> ("output_nRewards__R"=w2366:i32)  [unwired: 11 in]
              n928 = call "myRIO_BRig_RT_dataCurrent_Tcycle_generic.vi"() -> ("output_Tcycle_generic"=w2386:i32)  [unwired: 11 in]
              n929 = call "myRIO_BRig_RT_dataCurrent_count_generic.vi"() -> ("output_count_generic"=w2388:i32)  [unwired: 11 in]
              n930 = case shown="\"Left\", Default" w2360 {
                tunnel: w2372 -> [w2393 w2397]
                tunnel: [w2392 w2397] -> w2371
                tunnel: [w2394 w2395] -> w2370
                tunnel: w2369 -> [w2394 w2396]
                frame "Left", Default {
                  n931 = Increment(x=w2393) -> (x+1=w2392:u16)
                }
                frame "Right" {
                  n932 = Increment(x=w2396) -> (x+1=w2395:u16)
                }
              }
              "nRewards_Left" <- w2371
              "nRewards_Right" <- w2370
              n933 = Equal?(x=w2360, y=enum16{"Left", "Right"}."Left") -> (x = y?=w2359:bool)
              n934 = Select(t=w2367, s=w2359, f=w2366) -> (s? t:f=w2365:i32)
              n935 = call "myRIO_BRig_RT_dataExp_Tcycle_RewardPost.vi"() -> ("output_Tcycle_RewardPost"=w2382:i32)  [unwired: 11 in]
              n936 = call "myRIO_BRig_RT_dataCurrent_nRewTrials.vi"() -> ("output_nRewTrials"=w2368:i32)  [unwired: 11 in]
              n937 = Index Array(array=w2383, index=w2382) -> (element=w2385:u16)
              n938 = Index Array(array=w2362, index=w2368) -> (element=w2357:u16)
              n939 = Replace Array Subset(array=w2362, new element #1=u16 0 ("new element/subarray"), index #1=w2388, new element #2=w2385, index #2=w2386) -> (w2384:u16[])
              n940 = Replace Array Subset(array=w2364, new element=w2357, index (row)=w2358, index (col)=w2365) -> (w2363:u16[][])
              n941 = local write "nRewards_cur"(w2357) -> ()
            }
            frame "SelectRewardPost" {
              n942 = call "myRIO_BRig_RT__Case_Exp_State_RewardPost.vi"("input_state"=w2412, "input_dataCurrent"=w2415) -> ("output_state"=w2413:T2, "output_dataCurrent"=w2414:u16[])  [unwired: 8 in]
            }
            frame "SelectWrong_pre" {
              # "iState"
              # "Tcycle"
              # "counter"
              n943 = call "myRIO_BRig_RT_dataCurrent_Tcycle_generic.vi"() -> ("output_Tcycle_generic"=w2440:i32)  [unwired: 11 in]
              n944 = call "myRIO_BRig_RT_dataCurrent_count_generic.vi"() -> ("output_count_generic"=w2442:i32)  [unwired: 11 in]
              n945 = call "myRIO_BRig_RT_dataExp_Tcycle_Wrong.vi"() -> ("output_Tcycle_Wrong"=w2438:i32)  [unwired: 11 in]
              n946 = call "myRIO_BRig_RT__Case_Exp_subState_LC__Wrong.vi"("input_spout"=w2434, "input_dataCurrent"=w2435, "input_dataLC"=w2432) -> ()  [unwired: 6 in, 2 out]
              n947 = Index Array(array=w2436, index=w2438) -> (element=w2439:u16)
              n948 = call "myRIO_BRig_RT_dataCurrent_iState.vi"() -> ("output_iState"=w2426:i32)  [unwired: 11 in]
              n949 = Replace Array Subset(array=w2435, new element #1=u16 0 ("new element/subarray"), index #1=w2442, new element #2=w2439, index #2=w2440, new element #3=u16 2 ("new element/subarray"), index #3=w2426) -> (w2437:u16[])
            }
            frame "SelectWrong" {
              n950 = call "myRIO_BRig_RT__Case_Exp_State_Wrong.vi"("input_state"=w2456, "input_dataCurrent"=w2465) -> ("output_state"=w2453:T2, "output_dataCurrent"=w2464:u16[])  [unwired: 8 in]
              n951 = Not Equal?(x=w2456, y=w2453) -> (x != y?=w2455:bool)
              n952 = Select(t=myRIO_BRig_RT__Case_Exp_stateList."SelectWrong_post" ("Enum"), s=w2455, f=w2453) -> (s? t:f=w2452:T2)
            }
            frame "SelectWrong_post" {
            }
            frame "SelectTimeout_pre" {
              # "iState"
              # "Tcycle"
              # "counter"
              n953 = xnode "Read/Write Control"("FPGA VI Reference In"=w2492, "error in"=w2491, "SelectionState"=FALSE) -> ("error out"=→"error out 3":errorcluster)  [unwired: 1 out]
              n954 = call "myRIO_BRig_RT_dataCurrent_Tcycle_generic.vi"() -> ("output_Tcycle_generic"=w2514:i32)  [unwired: 11 in]
              n955 = call "myRIO_BRig_RT_dataCurrent_count_generic.vi"() -> ("output_count_generic"=w2512:i32)  [unwired: 11 in]
              n956 = call "myRIO_BRig_RT_dataExp_Tcycle_Timeout.vi"() -> ("output_Tcycle_Timeout"=w2516:i32)  [unwired: 11 in]
              n957 = call "myRIO_BRig_RT__Case_Exp_subState_LC__Timeout.vi"("input_spout"=w2507, "input_dataCurrent"=w2508, "input_dataLC"=w2506) -> ()  [unwired: 6 in, 2 out]
              n958 = Index Array(array=w2510, index=w2516) -> (element=w2515:u16)
              n959 = call "myRIO_BRig_RT_dataCurrent_iState.vi"() -> ("output_iState"=w2500:i32)  [unwired: 11 in]
              n960 = Replace Array Subset(array=w2508, new element #1=u16 0 ("new element/subarray"), index #1=w2512, new element #2=w2515, index #2=w2514, new element #3=u16 3 ("new element/subarray"), index #3=w2500) -> (w2511:u16[])
            }
            frame "SelectTimeout" {
              n961 = call "myRIO_BRig_RT__Case_Exp_State_Timeout.vi"("input_dataLC"=w2535, "input_LC"=w2536, "input_state"=w2526, "input_dataCurrent"=w2541) -> ("output_state"=w2527:T2, "output_dataCurrent"=w2540:u16[])  [unwired: 5 in, 1 out]
              n962 = Not Equal?(x=w2526, y=w2527) -> (x != y?=w2530:bool)
              n963 = Select(t=myRIO_BRig_RT__Case_Exp_stateList."SelectTimeout_post" ("Enum"), s=w2530, f=w2527) -> (s? t:f=w2528:T2)
            }
            frame "SelectTimeout_post" {
            }
            frame "endTrial1" {
              # "Update dataBlock"
              n964 = call "myRIO_BRig_RT__Case_Exp_State_endTrial1.vi"("input_spout"=w2574, "input_dataBlock"=w2573, "input_dataCurrent"=w2571) -> ("output_dataBlock"=w2572:u16[][], "output_dataCurrent"=w2570:u16[])  [unwired: 7 in]
            }
            frame "endTrial2" {
              # "update dataTrial"
              n965 = call "myRIO_BRig_RT__Case_Exp_State_endTrial2.vi"("input_spout"=w2593, "input_dataTrial"=w2597, "input_dataCurrent"=w2595) -> ("output_dataTrial"=w2596:u16[][], "output_dataCurrent"=w2594:u16[])  [unwired: 7 in]
            }
            frame "endTrial3" {
              w2623 = myRIO_BRig_RT__Case_Exp_stateList."endBlock" ("Enum")
              # "nRewTrials"
              # "iTrial"
              # "I_blockUntilReward"
              # "TPB"
              # "end block?"
              n966 = local read "STOP_endTrial"() -> (w2621:bool)
              n967 = local read "STOP_abort"() -> (w2620:bool)
              n968 = xnode "Read/Write Control"("FPGA VI Reference In"=w2609, "error in"=w2608, "SelectionState"=FALSE) -> ("error out"=→"error out 2":errorcluster)  [unwired: 1 out]
              n969 = local read "START"() -> (w2618:bool)
              n970 = call "myRIO_BRig_RT_dataExp_IblockUntilReward.vi"() -> ("output_I_blockUntilReward"=w2630:i32)  [unwired: 11 in]
              n971 = Index Array(array=w2614, index=w2630) -> (element=w2610:u16)
              n972 = Not(x=w2618) -> (.not. x?=w2619:bool)
              n973 = Not Equal To 0?(x=w2610) -> (x != 0?=w2628:bool)
              n974 = Compound Arithmetic op=OR(w2621, w2619, w2620) -> (w2622:bool)
              n975 = call "myRIO_BRig_RT_dataCurrent_nRewTrials.vi"() -> ("output_nRewTrials"=w2626:i32)  [unwired: 11 in]
              n976 = call "myRIO_BRig_RT_dataCurrent_iTrial.vi"() -> ("output_iTrial"=w2627:i32)  [unwired: 11 in]
              n977 = Select(t=w2626, s=w2628, f=w2627) -> (s? t:f=w2625:i32)
              n978 = call "myRIO_BRig_RT_dataCurrent_TpB.vi"() -> ("output_TpB"=w2629:i32)  [unwired: 11 in]
              n979 = Index Array(array=w2615, index #1=w2629, index #2=w2625) -> (element #1=w2616:u16, element #2=w2617:u16)
              n980 = Less Or Equal?(x=w2616, y=w2617) -> (x <= y?=w2613:bool)
              n981 = Select(t=w2623, s=w2613, f=myRIO_BRig_RT__Case_Exp_stateList."empty_endTrial1" ("Enum")) -> (s? t:f=w2624:T2)
              n982 = Select(t=w2623, s=w2622, f=w2624) -> (s? t:f=w2611:T2)
            }
            frame "endBlock" {
              # "R"
              # "L"
              # "idxDataBlock"
              n983 = Equal?(x=w2654, y=enum16{"Left", "Right"}."Left") -> (x = y?=w2653:bool)
              n984 = call "myRIO_BRig_RT_dataCurrent_idxDataBlockL.vi"() -> ("output_idxDataBlock__L"=w2657:i32)  [unwired: 11 in]
              n985 = call "myRIO_BRig_RT_dataCurrent_idxDataBlockR.vi"() -> ("output_idxDataBlock__R"=w2656:i32)  [unwired: 11 in]
              n986 = Increment(x=w2648) -> (x+1=w2647:i32)
              n987 = Select(t=w2657, s=w2653, f=w2656) -> (s? t:f=w2651:i32)
              n988 = To Unsigned Word Integer(number=w2647) -> (unsigned 16bit integer=w2649:u16)
              n989 = local read "START"() -> (w2677:bool)
              n990 = local read "STOP_endBlock"() -> (w2672:bool)
              n991 = local read "STOP_endTrial"() -> (w2675:bool)
              n992 = local read "STOP_abort"() -> (w2674:bool)
              n993 = Replace Array Subset(array=w2652, new element=w2649, index=w2651) -> (w2650:u16[])
              n994 = Not(x=w2677) -> (.not. x?=w2676:bool)
              n995 = Compound Arithmetic op=OR(w2676, w2672, w2675, w2674) -> (w2673:bool)
              n996 = Select(t=myRIO_BRig_RT__Case_Exp_stateList."endExp" ("Enum"), s=w2673, f=myRIO_BRig_RT__Case_Exp_stateList."empty_endBlock1" ("Enum")) -> (s? t:f=w2681:T2)
            }
            frame "endExp" {
            }
            frame "commConnect" {
              n997 = call "myRIO_BRig_RT_comm_webdav_connect.vi"("input_password"="Host Password", "input_username"="Host UserName") -> ("output_Iconnected"=w2702:bool, "output_hSession"=w2720:T6)  [unwired: 7 in, 1 out]
              "Connected To Host?" <- w2702
              n998 = case shown="False" w2702 {
                frame False {
                  n999 = One Button Dialog(message="Connection Failed!\nData not being saved!") -> ()  [unwired: 1 in, 1 out]
                }
                frame True {
                }
              }
            }
            frame "commUpload_pre" {
              n1000 = Select(t=myRIO_BRig_RT__Case_Exp_stateList."commUpload_dataBlock" ("Enum"), s=w2727, f=myRIO_BRig_RT__Case_Exp_stateList."endTrial3") -> (s? t:f=w2725:T2)
            }
            frame "commUpload_dataBlock" {
              n1001 = call "myRIO_BRig_RT_comm_webdav_uploadFile__data.vi"("input_fileName_prefix"=w2748, "input_fileName"="dataBlock" ("input_filename"), "input_hSession"=w2750) -> ()  [unwired: 8 in, 1 out]
            }
            frame "commUpload_dataCurrent" {
              n1002 = call "myRIO_BRig_RT_comm_webdav_uploadFile__data.vi"("input_fileName_prefix"=w2769, "input_fileName"="dataCurrent" ("input_filename"), "input_hSession"=w2771) -> ()  [unwired: 8 in, 1 out]
            }
            frame "commUpload_dataExp" {
              n1003 = call "myRIO_BRig_RT_comm_webdav_uploadFile__data.vi"("input_fileName_prefix"=w2790, "input_fileName"="dataExp" ("input_filename"), "input_hSession"=w2792) -> ()  [unwired: 8 in, 1 out]
            }
            frame "commUpload_dataLC" {
              n1004 = call "myRIO_BRig_RT_comm_webdav_uploadFile__data.vi"("input_fileName_prefix"=w2811, "input_fileName"="dataLC" ("input_filename"), "input_hSession"=w2813) -> ()  [unwired: 8 in, 1 out]
            }
            frame "commUpload_dataTrial" {
              n1005 = call "myRIO_BRig_RT_comm_webdav_uploadFile__data.vi"("input_fileName_prefix"=w2835, "input_fileName"="dataTrial" ("input_filename"), "input_hSession"=w2837) -> ()  [unwired: 8 in, 1 out]
            }
            frame "saveData_dataBlock" {
              # "idxDataBlockR"
              # "idxDataBlockL"
              n1006 = call "myRIO_BRig_RT_dataCurrent_idxDataBlockL.vi"() -> ("output_idxDataBlock__L"=w2861:i32)  [unwired: 11 in]
              n1007 = call "myRIO_BRig_RT_dataCurrent_idxDataBlockR.vi"() -> ("output_idxDataBlock__R"=w2862:i32)  [unwired: 11 in]
              n1008 = Index Array(array=w2863, index #1=w2861, index #2=w2862) -> (element #1=w2860:u16, element #2=w2859:u16)
              n1009 = Greater?(x=w2860, y=w2859) -> (0:w2858:bool)
              n1010 = Select(t=w2860, s=w2858, f=w2859) -> (s? t:f=w2856:u16)
              n1011 = Increment(x=w2856) -> (x+1=w2855:u16)
              n1012 = To Long Integer(number=w2855) -> (32bit integer=w2854:i32)
              n1013 = Array Subset(array=w2857, length (row)=w2854) -> (w2853:u16[][])  [unwired: 3 in]
              n1014 = call "myRIO_BRig_RT_comm_webdav_saveArrayToFile__2D_u16.vi"("Array"=w2853, "input_filename"="dataBlock") -> ()  [unwired: 10 in]
            }
            frame "saveData_dataCurrent" {
              n1015 = call "myRIO_BRig_RT_comm_webdav_saveArrayToFile__1D_u16.vi"("Array"=w2882, "input_filename"="dataCurrent") -> ()  [unwired: 10 in]
            }
            frame "saveData_dataExp" {
              # "runTime"
              n1016 = Get Date/Time In Seconds() -> (seconds since 1Jan1904=w2910:timestamp)
              n1017 = To Double Precision Float(number=w2910) -> (double precision float=w2909:dbl)
              n1018 = call "myRIO_BRig_RT_dataExp_runTime_seconds.vi"() -> ("output_RunTime_minutes"=w2908:i32)  [unwired: 11 in]
              n1019 = Subtract(x=w2909, y=w2907) -> (x-y=w2904:dbl)
              n1020 = To Unsigned Word Integer(number=w2904) -> (unsigned 16bit integer=w2903:u16)
              n1021 = Replace Array Subset(array=w2902, new element=w2903, index=w2908) -> (w2905:u16[])
              n1022 = call "myRIO_BRig_RT_comm_webdav_saveArrayToFile__1D_u16.vi"("Array"=w2905, "input_filename"="dataExp") -> ()  [unwired: 10 in]
            }
            frame "saveData_dataLC" {
              n1023 = call "myRIO_BRig_RT_comm_webdav_saveArrayToFile__1D_u16.vi"("Array"=w2929, "input_filename"="dataLC") -> ()  [unwired: 10 in]
            }
            frame "saveData_dataTrial" {
              # "idxTrial"
              n1024 = call "myRIO_BRig_RT_dataCurrent_idxDataTrial.vi"() -> ("output_idxDataTrial"=w2954:i32)  [unwired: 11 in]
              n1025 = Index Array(array=w2955, index=w2954) -> (element=w2951:u16)
              n1026 = Increment(x=w2951) -> (x+1=w2950:u16)
              n1027 = To Long Integer(number=w2950) -> (32bit integer=w2949:i32)
              n1028 = Array Subset(array=w2952, length (row)=w2949) -> (w2953:u16[][])  [unwired: 3 in]
              n1029 = call "myRIO_BRig_RT_comm_webdav_saveArrayToFile__2D_u16.vi"("Array"=w2953, "input_filename"="dataTrial") -> ()  [unwired: 10 in]
            }
            frame "empty_endBlock1" {
            }
            frame "empty_endBlock2" {
            }
            frame "empty_endTrial1" {
            }
            frame "empty_endTrial2" {
            }
            frame "empty_endTrial3" {
            }
            frame "empty_endTrial4" {
            }
            frame "empty_endTrial5" {
            }
          }
          n1030 = case shown="True" w1103 {
            tunnel: w1099 -> [w1126 w1134]
            tunnel: w1102 -> [_ w1130]
            tunnel: w1101 -> [_ w1129]
            tunnel: w1100 -> [_ w1128]
            tunnel: w1069 -> [_ w1127]
            tunnel: [w1126 w1133] -> w1098
            tunnel: w1097 -> [w1125 w1132]
            tunnel: [w1125 w1131] -> w1096
            frame False {
            }
            frame True {
              n1031 = call "myRIO_BRig_RT__Case_Exp__recordLick.vi"("intput_state__trialEnd"=w1127, "intput_state__trialStart"=w1128, "input_lick__R"=w1129, "input_lick__L"=w1130, "input_dataCurrent"=w1132, "input_dataLick"=w1134) -> ("output_dataCurrent"=w1131:u16[], "output_dataLick"=w1133:u16[][])  [unwired: 4 in]
            }
          }
          n1032 = Or(x=w1071, y=w1072) -> (x .or. y?=w1058:bool)
          n1033 = Or(x=w1075, y=w1055) -> (x .or. y?=w1044:bool)
          n1034 = Or(x=w1054, y=w1076) -> (x .or. y?=w1070:bool)
          n1035 = Or(x=w1074, y=w1073) -> (x .or. y?=w1059:bool)
          n1036 = Or(x=w1104, y="STOP_abort") -> (x .or. y?=w1106:bool)
          n1037 = Or(x=w1033, y=w1034) -> (x .or. y?=w1031:bool)
          n1038 = Or(x=w1035, y=w1034) -> (x .or. y?=w1032:bool)
          n1039 = xnode "Read/Write Control"("FPGA VI Reference In"=w1046, "error in"=w1045, "A1_SR"=w1059, "A3_SL"=w1058, "A6_Act"="Recording_p2", "audioTrigger_L"=w1044, "audioAmp_L"=w1085, "audioFreq_L_kHz"=w1053, "audioTrigger_R"=w1070, "audioAmp_R"=w1086, "audioFreq_R_kHz"=w1087, "laserledMTrig"=w1031, "laserMTrig"=w1032) -> ("FPGA VI Reference Out"=w1095:refnum<k20>, "error out"=w1094:errorcluster)
          n1040 = node-c288() -> ()  [unwired: 1 in, 1 out]
          "cState" <- w1100
        }
        n1041 = node-c288(w989) -> ()  [unwired: 1 out]
        n1042 = flat-sequence {
          tunnel: w985 -> [w1023]
          tunnel: w984 -> [w1022]
          tunnel: [w1021] -> w977
          tunnel: [w1020] -> w976
          tunnel: [w1026] -> w978
          tunnel: [w1027] -> w983
          tunnel: w977 -> [w1027]
          tunnel: w976 -> [w1026]
          frame #0 {
            w1017 = u8 0
            w1018 = u16 0 ("AudioLeft_phase_inc")
            w1019 = FALSE
            n1043 = xnode "Read/Write Control"("FPGA VI Reference In"=w1023, "error in"=w1022, "Counts_Reset"=TRUE, "audioTrigger_L"=w1019, "audioFreq_L_kHz"=w1017, "audioAmp_L"=w1018, "audioTrigger_R"=w1019, "audioFreq_R_kHz"=w1017, "audioAmp_R"=w1018, "A3_SL"=w1019, "A1_SR"=w1019, "A6_Act"=w1019) -> ("FPGA VI Reference Out"=w1021:refnum<k20>, "error out"=w1020:errorcluster)
          }
          frame #1 {
            w1025 = FALSE ("START")
            n1044 = local write "START"(w1025) -> ()
            n1045 = local write "STOP_endTrial"(w1025) -> ()
            n1046 = local write "STOP_endBlock"(w1025) -> ()
          }
        }
        n1047 = stacked-sequence {
          tunnel: w961 -> [w997 _]
          tunnel: w959 -> [w998 _]
          tunnel: w958 -> [_ w1003]
          tunnel: w957 -> [_ w1002]
          tunnel: w956 -> [_ w1001]
          tunnel: w955 -> [w991 _]
          frame #0 {
            n1048 = call "myRIO_BRig_RT_dataCurrent_idxDataLick.vi"() -> ("output_idxDataLick"=w992:i32)  [unwired: 11 in]
            n1049 = Index Array(array=w991, index=w992) -> (element=w994:u16)
            n1050 = Increment(x=w994) -> (x+1=w995:u16)
            n1051 = call "myRIO_BRig_RT_comm_webdav_saveArrayToFile__1D_u16.vi"("Array"=w998, "input_filename"="dataMTrig") -> ()  [unwired: 10 in]
            n1052 = To Long Integer(number=w995) -> (32bit integer=w993:i32)
            n1053 = Array Subset(array=w997, length (row)=w993) -> (w996:u16[][])  [unwired: 3 in]
            n1054 = call "myRIO_BRig_RT_comm_webdav_saveArrayToFile__2D_u16.vi"("Array"=w996, "input_filename"="dataLick") -> ()  [unwired: 10 in]
          }
          frame #1 {
            n1055 = case shown="True" w1003 {
              tunnel: w1002 -> [_ w1005]
              tunnel: w1001 -> [_ w1004]
              frame False {
              }
              frame True {
                n1056 = stacked-sequence {
                  tunnel: w1005 -> [w1007 w1014 w1016]
                  tunnel: w1004 -> [w1008 w1013 _]
                  frame #0 {
                    n1057 = call "myRIO_BRig_RT_comm_webdav_uploadFile__announce.vi"("input_addText"=TRUE, "input_fileName_prefix"=w1008, "intput_fileName"="curExp_end", "intput_hSession"=w1007) -> ("output_Isuccess"=w1006:bool)  [unwired: 6 in, 1 out]
                    n1058 = case shown="True" w1006 {
                      frame False {
                        n1059 = One Button Dialog(message="!!! Warning !!! Your data is located at C:\\BehaviorRig\\commTransfer") -> ()  [unwired: 1 in, 1 out]
                      }
                      frame True {
                        n1060 = Wait (ms)(milliseconds to wait=u32 20) -> ()  [unwired: 1 out]
                      }
                    }
                  }
                  frame #1 {
                    n1061 = call "myRIO_BRig_RT__endExp_sendData.vi"("input_fileName_prefix"=w1013, "input_hSession"=w1014) -> ()  [unwired: 8 in, 2 out]
                  }
                  frame #2 {
                    n1062 = local write "Connected To Host?"(FALSE ("Connected To Host?")) -> ()
                    n1063 = call <vilib>:"Close Session.vi"("session handle"=w1016) -> ()  [unwired: 14 in, 1 out]
                  }
                }
              }
            }
          }
        }
      }
    }
    n1064 = local read "STOP_abort"() -> (w30:bool)
  }
  n1065 = xnode "Read/Write Control"("FPGA VI Reference In"=w8, "error in"=w7, "FPGA_Stop"=TRUE) -> ("FPGA VI Reference Out"=w13:refnum<k20>, "error out"=w14:errorcluster)
  n1066 = xnode "Close FPGA VI Reference"("FPGA VI Reference In"=w13, "error in"=w14) -> ("error out"=w12:errorcluster)
  n1067 = call <vilib>:"Reset myRIO.vi"("error in (no error)"=w12) -> ()  [unwired: 10 in, 1 out]
